vi "单体采集信息-new1.vi"(0 "can卡类型":u8, 1 "设备索引号":u8, 2 "CAN端口":u8, 3 "VIC_Receive":refnum<vi>, 4 "数据":refnum<vi>, 5 "数据位置":refnum<vi>) -> ()   [LabVIEW 2013]
panel:
  out "Life:":dbl=25.0
  in  "213":bool
  in  "一次置位":bool
  in  "刷新":bool
  out "VCI_Receive 2":T1
  in  "板号":u8
  out "电池信息":T2
  in  "电池信息读取":bool
  out "时间":string
  in  "充电均衡":u32(colorbox)=6618880
  in  "放电均衡":u32(colorbox)=16711680
  out "均衡信息":string[][](table)=[["第1串", "1", "单体检测其它故障", "第25串", "1", "单体检测其它故障", "第49串", "1", "单体检测其它故障", "第73串", "1", "单体检测其它故障", "第97串", "1", "单体检测其它故障", "第121串", "1", "单体检测其它故障", "第145串", "1", "单体检测其它故障", "第169串", "1", "单体检测其它故障", "第193串", "1", "单体检测其它故障", "第217串", "1", "单体检测其它故障", "第241串", "1", "单体检测其它故障", "第265串", "1", "单体检测其它故障", "第289串", "1", "单体检测其它故障", ""], ["第2串", "", "", "第26串", "", "", "第50串", "", "", "第74串", "", "", "第98串", "", "", "第122串", "", "", "第146串", "", "", "第170串", "", "", "第194串", "", "", "第218串", "", "", "第242串", "", "", "第266串", "", "", "第290串", "", "", ""], ["第3串", "", "", "第27串", "", "", "第51串", "", "", "第75串", "", "", "第99串", "", "", "第123串", "", "", "第147串", "", "", "第171串", "", "", "第195串", "", "", "第219串", "", "", "第243串", "", "", "第267串", "", "", "第291串", "", "", ""], ["第4串", "", "", "第28串", "", "", "第52串", "", "", "第76串", "", "", "第100串", "", "", "第124串", "", "", "第148串", "", "", "第172串", "", "", "第196串", "", "", "第220串", "", "", "第244串", "", "", "第268串", "", "", "第292串", "", "", ""], ["第5串", "", "", "第29串", "", "", "第53串", "", "", "第77串", "", "", "第101串", "", "", "第125串", "", "", "第149串", "", "", "第173串", "", "", "第197串", "", "", "第221串", "", "", "第245串", "", "", "第269串", "", "", "第293串", "", "", ""], ["第6串", "", "", "第30串", "", "", "第54串", "", "", "第78串", "", "", "第102串", "", "", "第126串", "", "", "第150串", "", "", "第174串", "", "", "第198串", "", "", "第222串", "", "", "第246串", "", "", "第270串", "", "", "第294串", "", "", ""], ["第7串", "", "", "第31串", "", "", "第55串", "", "", "第79串", "", "", "第103串", "", "", "第127串", "", "", "第151串", "", "", "第175串", "", "", "第199串", "", "", "第223串", "", "", "第247串", "", "", "第271串", "", "", "第295串", "", "", ""], ["第8串", "", "", "第32串", "", "", "第56串", "", "", "第80串", "", "", "第104串", "", "", "第128串", "", "", "第152串", "", "", "第176串", "", "", "第200串", "", "", "第224串", "", "", "第248串", "", "", "第272串", "", "", "第296串", "", "", ""], ["第9串", "", "", "第33串", "", "", "第57串", "", "", "第81串", "", "", "第105串", "", "", "第129串", "", "", "第153串", "", "", "第177串", "", "", "第201串", "", "", "第225串", "", "", "第249串", "", "", "第273串", "", "", "第297串", "", "", ""], ["第10串", "", "", "第34串", "", "", "第58串", "", "", "第82串", "", "", "第106串", "", "", "第130串", "", "", "第154串", "", "", "第178串", "", "", "第202串", "", "", "第226串", "", "", "第250串", "", "", "第274串", "", "", "第298串", "", "", ""], ["第11串", "", "", "第35串", "", "", "第59串", "", "", "第83串", "", "", "第107串", "", "", "第131串", "", "", "第155串", "", "", "第179串", "", "", "第203串", "", "", "第227串", "", "", "第251串", "", "", "第275串", "", "", "第299串", "", "", ""], ["第12串", "", "", "第36串", "", "", "第60串", "", "", "第84串", "", "", "第108串", "", "", "第132串", "", "", "第156串", "", "", "第180串", "", "", "第204串", "", "", "第228串", "", "", "第252串", "", "", "第276串", "", "", "第300串", "", "", ""], ["第13串", "", "", "第37串", "", "", "第61串", "", "", "第85串", "", "", "第109串", "", "", "第133串", "", "", "第157串", "", "", "第181串", "", "", "第205串", "", "", "第229串", "", "", "第253串", "", "", "第277串", "", "", "", "", "", ""], ["第14串", "", "", "第38串", "", "", "第62串", "", "", "第86串", "", "", "第110串", "", "", "第134串", "", "", "第158串", "", "", "第182串", "", "", "第206串", "", "", "第230串", "", "", "第254串", "", "", "第278串", "", "", "", "", "", ""], ["第15串", "", "", "第39串", "", "", "第63串", "", "", "第87串", "", "", "第111串", "", "", "第135串", "", "", "第159串", "", "", "第183串", "", "", "第207串", "", "", "第231串", "", "", "第255串", "", "", "第279串", "", "", "", "", "", ""], ["第16串", "", "", "第40串", "", "", "第64串", "", "", "第88串", "", "", "第112串", "", "", "第136串", "", "", "第160串", "", "", "第184串", "", "", "第208串", "", "", "第232串", "", "", "第256串", "", "", "第280串", "", "", "", "", "", ""], ["第17串", "", "", "第41串", "", "", "第65串", "", "", "第89串", "", "", "第113串", "", "", "第137串", "", "", "第161串", "", "", "第185串", "", "", "第209串", "", "", "第233串", "", "", "第257串", "", "", "第281串", "", "", "", "", "", ""], ["第18串", "", "", "第42串", "", "", "第66串", "", "", "第90串", "", "", "第114串", "", "", "第138串", "", "", "第162串", "", "", "第186串", "", "", "第210串", "", "", "第234串", "", "", "第258串", "", "", "第282串", "", "", "", "", "", ""], ["第19串", "", "", "第43串", "", "", "第67串", "", "", "第91串", "", "", "第115串", "", "", "第139串", "", "", "第163串", "", "", "第187串", "", "", "第211串", "", "", "第235串", "", "", "第259串", "", "", "第283串", "", "", "", "", "", ""], ["第20串", "", "", "第44串", "", "", "第68串", "", "", "第92串", "", "", "第116串", "", "", "第140串", "", "", "第164串", "", "", "第188串", "", "", "第212串", "", "", "第236串", "", "", "第260串", "", "", "第284串", "", "", "", "", "", ""], ["第21串", "", "", "第45串", "", "", "第69串", "", "", "第93串", "", "", "第117串", "", "", "第141串", "", "", "第165串", "", "", "第189串", "", "", "第213串", "", "", "第237串", "", "", "第261串", "", "", "第285串", "", "", "", "", "", ""], ["第22串", "", "", "第46串", "", "", "第70串", "", "", "第94串", "", "", "第118串", "", "", "第142串", "", "", "第166串", "", "", "第190串", "", "", "第214串", "", "", "第238串", "", "", "第262串", "", "", "第286串", "", "", "", "", "", ""], ["第23串", "", "", "第47串", "", "", "第71串", "", "", "第95串", "", "", "第119串", "", "", "第143串", "", "", "第167串", "", "", "第191串", "", "", "第215串", "", "", "第239串", "", "", "第263串", "", "", "第287串", "", "", "", "", "", ""], ["第24串", "", "", "第48串", "", "", "第72串", "", "", "第96串", "", "", "第120串", "", "", "第144串", "", "", "第168串", "", "", "第192串", "", "", "第216串", "", "", "第240串", "", "", "第264串", "", "", "第288串", "", "", "", "", "", ""]]
  out "SOC":string[][](table)=[["第1串", "", "", "第25串", "", "", "第49串", "", "", "第73串", "", "", "第97串", "", "", "第121串", "", "", "第145串", "", "", "第169串", "", "", "第193串", "", "", "第217串", "", "", "第241串", "", "", "第265串", "", "", "第289串", "", "", ""], ["第2串", "", "", "第26串", "", "", "第50串", "", "", "第74串", "", "", "第98串", "", "", "第122串", "", "", "第146串", "", "", "第170串", "", "", "第194串", "", "", "第218串", "", "", "第242串", "", "", "第266串", "", "", "第290串", "", "", ""], ["第3串", "", "", "第27串", "", "", "第51串", "", "", "第75串", "", "", "第99串", "", "", "第123串", "", "", "第147串", "", "", "第171串", "", "", "第195串", "", "", "第219串", "", "", "第243串", "", "", "第267串", "", "", "第291串", "", "", ""], ["第4串", "", "", "第28串", "", "", "第52串", "", "", "第76串", "", "", "第100串", "", "", "第124串", "", "", "第148串", "", "", "第172串", "", "", "第196串", "", "", "第220串", "", "", "第244串", "", "", "第268串", "", "", "第292串", "", "", ""], ["第5串", "", "", "第29串", "", "", "第53串", "", "", "第77串", "", "", "第101串", "", "", "第125串", "", "", "第149串", "", "", "第173串", "", "", "第197串", "", "", "第221串", "", "", "第245串", "", "", "第269串", "", "", "第293串", "", "", ""], ["第6串", "", "", "第30串", "", "", "第54串", "", "", "第78串", "", "", "第102串", "", "", "第126串", "", "", "第150串", "", "", "第174串", "", "", "第198串", "", "", "第222串", "", "", "第246串", "", "", "第270串", "", "", "第294串", "", "", ""], ["第7串", "", "", "第31串", "", "", "第55串", "", "", "第79串", "", "", "第103串", "", "", "第127串", "", "", "第151串", "", "", "第175串", "", "", "第199串", "", "", "第223串", "", "", "第247串", "", "", "第271串", "", "", "第295串", "", "", ""], ["第8串", "", "", "第32串", "", "", "第56串", "", "", "第80串", "", "", "第104串", "", "", "第128串", "", "", "第152串", "", "", "第176串", "", "", "第200串", "", "", "第224串", "", "", "第248串", "", "", "第272串", "", "", "第296串", "", "", ""], ["第9串", "", "", "第33串", "", "", "第57串", "", "", "第81串", "", "", "第105串", "", "", "第129串", "", "", "第153串", "", "", "第177串", "", "", "第201串", "", "", "第225串", "", "", "第249串", "", "", "第273串", "", "", "第297串", "", "", ""], ["第10串", "", "", "第34串", "", "", "第58串", "", "", "第82串", "", "", "第106串", "", "", "第130串", "", "", "第154串", "", "", "第178串", "", "", "第202串", "", "", "第226串", "", "", "第250串", "", "", "第274串", "", "", "第298串", "", "", ""], ["第11串", "", "", "第35串", "", "", "第59串", "", "", "第83串", "", "", "第107串", "", "", "第131串", "", "", "第155串", "", "", "第179串", "", "", "第203串", "", "", "第227串", "", "", "第251串", "", "", "第275串", "", "", "第299串", "", "", ""], ["第12串", "", "", "第36串", "", "", "第60串", "", "", "第84串", "", "", "第108串", "", "", "第132串", "", "", "第156串", "", "", "第180串", "", "", "第204串", "", "", "第228串", "", "", "第252串", "", "", "第276串", "", "", "第300串", "", "", ""], ["第13串", "", "", "第37串", "", "", "第61串", "", "", "第85串", "", "", "第109串", "", "", "第133串", "", "", "第157串", "", "", "第181串", "", "", "第205串", "", "", "第229串", "", "", "第253串", "", "", "第277串", "", "", "", "", "", ""], ["第14串", "", "", "第38串", "", "", "第62串", "", "", "第86串", "", "", "第110串", "", "", "第134串", "", "", "第158串", "", "", "第182串", "", "", "第206串", "", "", "第230串", "", "", "第254串", "", "", "第278串", "", "", "", "", "", ""], ["第15串", "", "", "第39串", "", "", "第63串", "", "", "第87串", "", "", "第111串", "", "", "第135串", "", "", "第159串", "", "", "第183串", "", "", "第207串", "", "", "第231串", "", "", "第255串", "", "", "第279串", "", "", "", "", "", ""], ["第16串", "", "", "第40串", "", "", "第64串", "", "", "第88串", "", "", "第112串", "", "", "第136串", "", "", "第160串", "", "", "第184串", "", "", "第208串", "", "", "第232串", "", "", "第256串", "", "", "第280串", "", "", "", "", "", ""], ["第17串", "", "", "第41串", "", "", "第65串", "", "", "第89串", "", "", "第113串", "", "", "第137串", "", "", "第161串", "", "", "第185串", "", "", "第209串", "", "", "第233串", "", "", "第257串", "", "", "第281串", "", "", "", "", "", ""], ["第18串", "", "", "第42串", "", "", "第66串", "", "", "第90串", "", "", "第114串", "", "", "第138串", "", "", "第162串", "", "", "第186串", "", "", "第210串", "", "", "第234串", "", "", "第258串", "", "", "第282串", "", "", "", "", "", ""], ["第19串", "", "", "第43串", "", "", "第67串", "", "", "第91串", "", "", "第115串", "", "", "第139串", "", "", "第163串", "", "", "第187串", "", "", "第211串", "", "", "第235串", "", "", "第259串", "", "", "第283串", "", "", "", "", "", ""], ["第20串", "", "", "第44串", "", "", "第68串", "", "", "第92串", "", "", "第116串", "", "", "第140串", "", "", "第164串", "", "", "第188串", "", "", "第212串", "", "", "第236串", "", "", "第260串", "", "", "第284串", "", "", "", "", "", ""], ["第21串", "", "", "第45串", "", "", "第69串", "", "", "第93串", "", "", "第117串", "", "", "第141串", "", "", "第165串", "", "", "第189串", "", "", "第213串", "", "", "第237串", "", "", "第261串", "", "", "第285串", "", "", "", "", "", ""], ["第22串", "", "", "第46串", "", "", "第70串", "", "", "第94串", "", "", "第118串", "", "", "第142串", "", "", "第166串", "", "", "第190串", "", "", "第214串", "", "", "第238串", "", "", "第262串", "", "", "第286串", "", "", "", "", "", ""], ["第23串", "", "", "第47串", "", "", "第71串", "", "", "第95串", "", "", "第119串", "", "", "第143串", "", "", "第167串", "", "", "第191串", "", "", "第215串", "", "", "第239串", "", "", "第263串", "", "", "第287串", "", "", "", "", "", ""], ["第24串", "", "", "第48串", "", "", "第72串", "", "", "第96串", "", "", "第120串", "", "", "第144串", "", "", "第168串", "", "", "第192串", "", "", "第216串", "", "", "第240串", "", "", "第264串", "", "", "第288串", "", "", "", "", "", ""]]
  out "内阻":string[][](table)=[["第1串", "", "", "第25串", "", "", "第49串", "", "", "第73串", "", "", "第97串", "", "", "第121串", "", "", "第145串", "", "", "第169串", "", "", "第193串", "", "", "第217串", "", "", "第241串", "", "", "第265串", "", "", "第289串", "", "", ""], ["第2串", "", "", "第26串", "", "", "第50串", "", "", "第74串", "", "", "第98串", "", "", "第122串", "", "", "第146串", "", "", "第170串", "", "", "第194串", "", "", "第218串", "", "", "第242串", "", "", "第266串", "", "", "第290串", "", "", ""], ["第3串", "", "", "第27串", "", "", "第51串", "", "", "第75串", "", "", "第99串", "", "", "第123串", "", "", "第147串", "", "", "第171串", "", "", "第195串", "", "", "第219串", "", "", "第243串", "", "", "第267串", "", "", "第291串", "", "", ""], ["第4串", "", "", "第28串", "", "", "第52串", "", "", "第76串", "", "", "第100串", "", "", "第124串", "", "", "第148串", "", "", "第172串", "", "", "第196串", "", "", "第220串", "", "", "第244串", "", "", "第268串", "", "", "第292串", "", "", ""], ["第5串", "", "", "第29串", "", "", "第53串", "", "", "第77串", "", "", "第101串", "", "", "第125串", "", "", "第149串", "", "", "第173串", "", "", "第197串", "", "", "第221串", "", "", "第245串", "", "", "第269串", "", "", "第293串", "", "", ""], ["第6串", "", "", "第30串", "", "", "第54串", "", "", "第78串", "", "", "第102串", "", "", "第126串", "", "", "第150串", "", "", "第174串", "", "", "第198串", "", "", "第222串", "", "", "第246串", "", "", "第270串", "", "", "第294串", "", "", ""], ["第7串", "", "", "第31串", "", "", "第55串", "", "", "第79串", "", "", "第103串", "", "", "第127串", "", "", "第151串", "", "", "第175串", "", "", "第199串", "", "", "第223串", "", "", "第247串", "", "", "第271串", "", "", "第295串", "", "", ""], ["第8串", "", "", "第32串", "", "", "第56串", "", "", "第80串", "", "", "第104串", "", "", "第128串", "", "", "第152串", "", "", "第176串", "", "", "第200串", "", "", "第224串", "", "", "第248串", "", "", "第272串", "", "", "第296串", "", "", ""], ["第9串", "", "", "第33串", "", "", "第57串", "", "", "第81串", "", "", "第105串", "", "", "第129串", "", "", "第153串", "", "", "第177串", "", "", "第201串", "", "", "第225串", "", "", "第249串", "", "", "第273串", "", "", "第297串", "", "", ""], ["第10串", "", "", "第34串", "", "", "第58串", "", "", "第82串", "", "", "第106串", "", "", "第130串", "", "", "第154串", "", "", "第178串", "", "", "第202串", "", "", "第226串", "", "", "第250串", "", "", "第274串", "", "", "第298串", "", "", ""], ["第11串", "", "", "第35串", "", "", "第59串", "", "", "第83串", "", "", "第107串", "", "", "第131串", "", "", "第155串", "", "", "第179串", "", "", "第203串", "", "", "第227串", "", "", "第251串", "", "", "第275串", "", "", "第299串", "", "", ""], ["第12串", "", "", "第36串", "", "", "第60串", "", "", "第84串", "", "", "第108串", "", "", "第132串", "", "", "第156串", "", "", "第180串", "", "", "第204串", "", "", "第228串", "", "", "第252串", "", "", "第276串", "", "", "第300串", "", "", ""], ["第13串", "", "", "第37串", "", "", "第61串", "", "", "第85串", "", "", "第109串", "", "", "第133串", "", "", "第157串", "", "", "第181串", "", "", "第205串", "", "", "第229串", "", "", "第253串", "", "", "第277串", "", "", "", "", "", ""], ["第14串", "", "", "第38串", "", "", "第62串", "", "", "第86串", "", "", "第110串", "", "", "第134串", "", "", "第158串", "", "", "第182串", "", "", "第206串", "", "", "第230串", "", "", "第254串", "", "", "第278串", "", "", "", "", "", ""], ["第15串", "", "", "第39串", "", "", "第63串", "", "", "第87串", "", "", "第111串", "", "", "第135串", "", "", "第159串", "", "", "第183串", "", "", "第207串", "", "", "第231串", "", "", "第255串", "", "", "第279串", "", "", "", "", "", ""], ["第16串", "", "", "第40串", "", "", "第64串", "", "", "第88串", "", "", "第112串", "", "", "第136串", "", "", "第160串", "", "", "第184串", "", "", "第208串", "", "", "第232串", "", "", "第256串", "", "", "第280串", "", "", "", "", "", ""], ["第17串", "", "", "第41串", "", "", "第65串", "", "", "第89串", "", "", "第113串", "", "", "第137串", "", "", "第161串", "", "", "第185串", "", "", "第209串", "", "", "第233串", "", "", "第257串", "", "", "第281串", "", "", "", "", "", ""], ["第18串", "", "", "第42串", "", "", "第66串", "", "", "第90串", "", "", "第114串", "", "", "第138串", "", "", "第162串", "", "", "第186串", "", "", "第210串", "", "", "第234串", "", "", "第258串", "", "", "第282串", "", "", "", "", "", ""], ["第19串", "", "", "第43串", "", "", "第67串", "", "", "第91串", "", "", "第115串", "", "", "第139串", "", "", "第163串", "", "", "第187串", "", "", "第211串", "", "", "第235串", "", "", "第259串", "", "", "第283串", "", "", "", "", "", ""], ["第20串", "", "", "第44串", "", "", "第68串", "", "", "第92串", "", "", "第116串", "", "", "第140串", "", "", "第164串", "", "", "第188串", "", "", "第212串", "", "", "第236串", "", "", "第260串", "", "", "第284串", "", "", "", "", "", ""], ["第21串", "", "", "第45串", "", "", "第69串", "", "", "第93串", "", "", "第117串", "", "", "第141串", "", "", "第165串", "", "", "第189串", "", "", "第213串", "", "", "第237串", "", "", "第261串", "", "", "第285串", "", "", "", "", "", ""], ["第22串", "", "", "第46串", "", "", "第70串", "", "", "第94串", "", "", "第118串", "", "", "第142串", "", "", "第166串", "", "", "第190串", "", "", "第214串", "", "", "第238串", "", "", "第262串", "", "", "第286串", "", "", "", "", "", ""], ["第23串", "", "", "第47串", "", "", "第71串", "", "", "第95串", "", "", "第119串", "", "", "第143串", "", "", "第167串", "", "", "第191串", "", "", "第215串", "", "", "第239串", "", "", "第263串", "", "", "第287串", "", "", "", "", "", ""], ["第24串", "", "", "第48串", "", "", "第72串", "", "", "第96串", "", "", "第120串", "", "", "第144串", "", "", "第168串", "", "", "第192串", "", "", "第216串", "", "", "第240串", "", "", "第264串", "", "", "第288串", "", "", "", "", "", ""]]
  out "温度表格":string[][](table)=[["第1串", "", "", "第25串", "", "", "第49串", "", "", "第73串", "", "", "第97串", "", "", "第121串", "", "", "第145串", "", "", "第169串", "", "", "第193串", "", "", "第217串", "", "", "第241串", "", "", "第265串", "", "", "第289串", "", "", ""], ["第2串", "", "", "第26串", "", "", "第50串", "", "", "第74串", "", "", "第98串", "", "", "第122串", "", "", "第146串", "", "", "第170串", "", "", "第194串", "", "", "第218串", "", "", "第242串", "", "", "第266串", "", "", "第290串", "", "", ""], ["第3串", "", "", "第27串", "", "", "第51串", "", "", "第75串", "", "", "第99串", "", "", "第123串", "", "", "第147串", "", "", "第171串", "", "", "第195串", "", "", "第219串", "", "", "第243串", "", "", "第267串", "", "", "第291串", "", "", ""], ["第4串", "", "", "第28串", "", "", "第52串", "", "", "第76串", "", "", "第100串", "", "", "第124串", "", "", "第148串", "", "", "第172串", "", "", "第196串", "", "", "第220串", "", "", "第244串", "", "", "第268串", "", "", "第292串", "", "", ""], ["第5串", "", "", "第29串", "", "", "第53串", "", "", "第77串", "", "", "第101串", "", "", "第125串", "", "", "第149串", "", "", "第173串", "", "", "第197串", "", "", "第221串", "", "", "第245串", "", "", "第269串", "", "", "第293串", "", "", ""], ["第6串", "", "", "第30串", "", "", "第54串", "", "", "第78串", "", "", "第102串", "", "", "第126串", "", "", "第150串", "", "", "第174串", "", "", "第198串", "", "", "第222串", "", "", "第246串", "", "", "第270串", "", "", "第294串", "", "", ""], ["第7串", "", "", "第31串", "", "", "第55串", "", "", "第79串", "", "", "第103串", "", "", "第127串", "", "", "第151串", "", "", "第175串", "", "", "第199串", "", "", "第223串", "", "", "第247串", "", "", "第271串", "", "", "第295串", "", "", ""], ["第8串", "", "", "第32串", "", "", "第56串", "", "", "第80串", "", "", "第104串", "", "", "第128串", "", "", "第152串", "", "", "第176串", "", "", "第200串", "", "", "第224串", "", "", "第248串", "", "", "第272串", "", "", "第296串", "", "", ""], ["第9串", "", "", "第33串", "", "", "第57串", "", "", "第81串", "", "", "第105串", "", "", "第129串", "", "", "第153串", "", "", "第177串", "", "", "第201串", "", "", "第225串", "", "", "第249串", "", "", "第273串", "", "", "第297串", "", "", ""], ["第10串", "", "", "第34串", "", "", "第58串", "", "", "第82串", "", "", "第106串", "", "", "第130串", "", "", "第154串", "", "", "第178串", "", "", "第202串", "", "", "第226串", "", "", "第250串", "", "", "第274串", "", "", "第298串", "", "", ""], ["第11串", "", "", "第35串", "", "", "第59串", "", "", "第83串", "", "", "第107串", "", "", "第131串", "", "", "第155串", "", "", "第179串", "", "", "第203串", "", "", "第227串", "", "", "第251串", "", "", "第275串", "", "", "第299串", "", "", ""], ["第12串", "", "", "第36串", "", "", "第60串", "", "", "第84串", "", "", "第108串", "", "", "第132串", "", "", "第156串", "", "", "第180串", "", "", "第204串", "", "", "第228串", "", "", "第252串", "", "", "第276串", "", "", "第300串", "", "", ""], ["第13串", "", "", "第37串", "", "", "第61串", "", "", "第85串", "", "", "第109串", "", "", "第133串", "", "", "第157串", "", "", "第181串", "", "", "第205串", "", "", "第229串", "", "", "第253串", "", "", "第277串", "", "", "", "", "", ""], ["第14串", "", "", "第38串", "", "", "第62串", "", "", "第86串", "", "", "第110串", "", "", "第134串", "", "", "第158串", "", "", "第182串", "", "", "第206串", "", "", "第230串", "", "", "第254串", "", "", "第278串", "", "", "", "", "", ""], ["第15串", "", "", "第39串", "", "", "第63串", "", "", "第87串", "", "", "第111串", "", "", "第135串", "", "", "第159串", "", "", "第183串", "", "", "第207串", "", "", "第231串", "", "", "第255串", "", "", "第279串", "", "", "", "", "", ""], ["第16串", "", "", "第40串", "", "", "第64串", "", "", "第88串", "", "", "第112串", "", "", "第136串", "", "", "第160串", "", "", "第184串", "", "", "第208串", "", "", "第232串", "", "", "第256串", "", "", "第280串", "", "", "", "", "", ""], ["第17串", "", "", "第41串", "", "", "第65串", "", "", "第89串", "", "", "第113串", "", "", "第137串", "", "", "第161串", "", "", "第185串", "", "", "第209串", "", "", "第233串", "", "", "第257串", "", "", "第281串", "", "", "", "", "", ""], ["第18串", "", "", "第42串", "", "", "第66串", "", "", "第90串", "", "", "第114串", "", "", "第138串", "", "", "第162串", "", "", "第186串", "", "", "第210串", "", "", "第234串", "", "", "第258串", "", "", "第282串", "", "", "", "", "", ""], ["第19串", "", "", "第43串", "", "", "第67串", "", "", "第91串", "", "", "第115串", "", "", "第139串", "", "", "第163串", "", "", "第187串", "", "", "第211串", "", "", "第235串", "", "", "第259串", "", "", "第283串", "", "", "", "", "", ""], ["第20串", "", "", "第44串", "", "", "第68串", "", "", "第92串", "", "", "第116串", "", "", "第140串", "", "", "第164串", "", "", "第188串", "", "", "第212串", "", "", "第236串", "", "", "第260串", "", "", "第284串", "", "", "", "", "", ""], ["第21串", "", "", "第45串", "", "", "第69串", "", "", "第93串", "", "", "第117串", "", "", "第141串", "", "", "第165串", "", "", "第189串", "", "", "第213串", "", "", "第237串", "", "", "第261串", "", "", "第285串", "", "", "", "", "", ""], ["第22串", "", "", "第46串", "", "", "第70串", "", "", "第94串", "", "", "第118串", "", "", "第142串", "", "", "第166串", "", "", "第190串", "", "", "第214串", "", "", "第238串", "", "", "第262串", "", "", "第286串", "", "", "", "", "", ""], ["第23串", "", "", "第47串", "", "", "第71串", "", "", "第95串", "", "", "第119串", "", "", "第143串", "", "", "第167串", "", "", "第191串", "", "", "第215串", "", "", "第239串", "", "", "第263串", "", "", "第287串", "", "", "", "", "", ""], ["第24串", "", "", "第48串", "", "", "第72串", "", "", "第96串", "", "", "第120串", "", "", "第144串", "", "", "第168串", "", "", "第192串", "", "", "第216串", "", "", "第240串", "", "", "第264串", "", "", "第288串", "", "", "", "", "", ""]]
  in  "主界面选项":T3(radio)
  in  "电池信息选项":enum16{"电池信息", "历史信息"}(ring)
  out "位置":dbl[](array[numeric])
  out "输出数据":dbl[](array[numeric])
  in  "命令":u32=133
  in  "VCI_Receive":T1 {"Rsv3" max=0 format="%x"; "Rsv2" min=101 format="%x"; "Rsv1" format="%x"; "Data8" format="%x"; "Data7" format="%x"; "Data6" format="%x"; "Data5" format="%x"; "Data4" format="%x"; "Data3" format="%x"; "Data2" format="%x"; "Data1" format="%x"; "DataLen" format="%x"; "ExternFlag" format="%x"; "RemoteFlag" format="%x"; "SendType" format="%x"; "TimeFlag" format="%x"; "TimeStamp" format="%x"; "ID" format="%x"}
  out "状态":bool
  in  "停止":bool
  in  "选项卡控件":enum32{"单体电压", "单体温度", "单体内阻", "单体SOC"}(tab)
  in  "偏差":dbl=0.008 format="%.3f"
  in  "基准":dbl=3.3 format="%.3f"
  out "等待均衡":u32(colorbox)=16776770
  in  "故障信息选择按键 2":enum32{"单选选项2", "单选选项2 2", "单选选项2 3", "单选选项1"}(radio)=enum."单选选项1"
  out "电压选择":enum32{"1-96", "97-192", "193-288", "289-300"}(tab)
  out "1":T4={"1 102"={"第1串"=0.0, "第2串"=0.0, "第3串"=0.0, "第4串"=0.0, "第5串"=0.0, "第6串"=0.0, "第7串"=0.0, "第8串"=0.0, "第9串"=0.0, "第10串"=0.0, "第11串"=0.0, "第12串"=0.0, "第一串 2"=0.0, "第一串 4"=0.0, "第一串 6"=0.0, "第一串 8"=0.0, "第一串 10"=0.0, "第一串 12"=0.0, "第一串 14"=0.0, "第一串 16"=0.0, "第一串 18"=0.0, "第一串 20"=0.0, "第一串 22"=0.0, "第一串 24"=0.0}, "1 3"={"第13串"=0.0, "第14串"=0.0, "第15串"=0.0, "第16串"=0.0, "第17串"=0.0, "第18串"=0.0, "第19串"=0.0, "第20串"=0.0, "第21串"=0.0, "第22串"=0.0, "第23串"=0.0, "第24串"=0.0, "第一串 2"=0.0, "第一串 4"=0.0, "第一串 6"=0.0, "第一串 8"=0.0, "第一串 10"=0.0, "第一串 12"=0.0, "第一串 14"=0.0, "第一串 16"=0.0, "第一串 18"=0.0, "第一串 20"=0.0, "第一串 22"=0.0, "第一串 24"=0.0}, "1 4"={"第25串"=0.0, "第26串"=0.0, "第27串"=0.0, "第28串"=0.0, "第29串"=0.0, "第30串"=0.0, "第31串"=0.0, "第32串"=0.0, "第33串"=0.0, "第34串"=0.0, "第35串"=0.0, "第36串"=0.0, "第一串 2"=0.0, "第一串 4"=0.0, "第一串 6"=0.0, "第一串 8"=0.0, "第一串 10"=0.0, "第一串 12"=0.0, "第一串 14"=0.0, "第一串 16"=0.0, "第一串 18"=0.0, "第一串 20"=0.0, "第一串 22"=0.0, "第一串 24"=0.0}, "1 6"={"第37串"=0.0, "第38串"=0.0, "第39串"=0.0, "第40串"=0.0, "第41串"=0.0, "第42串"=0.0, "第43串"=0.0, "第44串"=0.0, "第45串"=0.0, "第46串"=0.0, "第47串"=0.0, "第48串"=0.0, "第一串 2"=0.0, "第一串 4"=0.0, "第一串 6"=0.0, "第一串 8"=0.0, "第一串 10"=0.0, "第一串 12"=0.0, "第一串 14"=0.0, "第一串 16"=0.0, "第一串 18"=0.0, "第一串 20"=0.0, "第一串 22"=0.0, "第一串 24"=0.0}, "1 7"={"第49串"=0.0, "第50串"=0.0, "第51串"=0.0, "第52串"=0.0, "第53串"=0.0, "第54串"=0.0, "第55串"=0.0, "第56串"=0.0, "第57串"=0.0, "第58串"=0.0, "第59串"=0.0, "第60串"=0.0, "第一串 2"=0.0, "第一串 4"=0.0, "第一串 6"=0.0, "第一串 8"=0.0, "第一串 10"=0.0, "第一串 12"=0.0, "第一串 14"=0.0, "第一串 16"=0.0, "第一串 18"=0.0, "第一串 20"=0.0, "第一串 22"=0.0, "第一串 24"=0.0}, "1 8"={"第61串"=0.0, "第62串"=0.0, "第63串"=0.0, "第64串"=0.0, "第65串"=0.0, "第66串"=0.0, "第67串"=0.0, "第68串"=0.0, "第69串"=0.0, "第70串"=0.0, "第71串"=0.0, "第72串"=0.0, "第一串 2"=0.0, "第一串 4"=0.0, "第一串 6"=0.0, "第一串 8"=0.0, "第一串 10"=0.0, "第一串 12"=0.0, "第一串 14"=0.0, "第一串 16"=0.0, "第一串 18"=0.0, "第一串 20"=0.0, "第一串 22"=0.0, "第一串 24"=0.0}, "1 9"={"第73串"=0.0, "第74串"=0.0, "第75串"=0.0, "第76串"=0.0, "第77串"=0.0, "第78串"=0.0, "第79串"=0.0, "第80串"=0.0, "第81串"=0.0, "第82串"=0.0, "第83串"=0.0, "第84串"=0.0, "第一串 2"=0.0, "第一串 4"=0.0, "第一串 6"=0.0, "第一串 8"=0.0, "第一串 10"=0.0, "第一串 12"=0.0, "第一串 14"=0.0, "第一串 16"=0.0, "第一串 18"=0.0, "第一串 20"=0.0, "第一串 22"=0.0, "第一串 24"=0.0}, "1 10"={"第85串"=0.0, "第86串"=0.0, "第87串"=0.0, "第88串"=0.0, "第89串"=0.0, "第90串"=0.0, "第91串"=0.0, "第92串"=0.0, "第93串"=0.0, "第94串"=0.0, "第95串"=0.0, "第96串"=0.0, "第一串 2"=0.0, "第一串 4"=0.0, "第一串 6"=0.0, "第一串 8"=0.0, "第一串 10"=0.0, "第一串 12"=0.0, "第一串 14"=0.0, "第一串 16"=0.0, "第一串 18"=0.0, "第一串 20"=0.0, "第一串 22"=0.0, "第一串 24"=0.0}, "1 12"={"充电1"=13816530, "充电1"=13816530, "充电1"=13816530, "充电1"=13816530, "充电1"=13816530, "充电1"=13816530, "充电1"=13816530, "充电1"=13816530, "充电1"=13816530, "充电1"=13816530, "充电1"=13816530, "充电1"=13816530}, "1 28"={"充电1"=13816530, "充电1"=13816530, "充电1"=13816530, "充电1"=13816530, "充电1"=13816530, "充电1"=13816530, "充电1"=13816530, "充电1"=13816530, "充电1"=13816530, "充电1"=13816530, "充电1"=13816530, "充电1"=13816530}, "1 25"={"充电1"=0, "充电1"=0, "充电1"=0, "充电1"=0, "充电1"=0, "充电1"=0, "充电1"=0, "充电1"=0, "充电1"=0, "充电1"=0, "充电1"=0, "充电1"=0}, "1 31"={"充电1"=0, "充电1"=0, "充电1"=0, "充电1"=0, "充电1"=0, "充电1"=0, "充电1"=0, "充电1"=0, "充电1"=0, "充电1"=0, "充电1"=0, "充电1"=0}, "1 16"={"充电1"=0, "充电1"=0, "充电1"=0, "充电1"=0, "充电1"=0, "充电1"=0, "充电1"=0, "充电1"=0, "充电1"=0, "充电1"=0, "充电1"=0, "充电1"=0}, "1 19"={"充电1"=0, "充电1"=0, "充电1"=0, "充电1"=0, "充电1"=0, "充电1"=0, "充电1"=0, "充电1"=0, "充电1"=0, "充电1"=0, "充电1"=0, "充电1"=0}, "1 22"={"充电1"=0, "充电1"=0, "充电1"=0, "充电1"=0, "充电1"=0, "充电1"=0, "充电1"=0, "充电1"=0, "充电1"=0, "充电1"=0, "充电1"=0, "充电1"=0}, "1 34"={"充电1"=0, "充电1"=0, "充电1"=0, "充电1"=0, "充电1"=0, "充电1"=0, "充电1"=0, "充电1"=0, "充电1"=0, "充电1"=0, "充电1"=0, "充电1"=0}, "1 11"={"充电1"=13816530, "充电1"=13816530, "充电1"=13816530, "充电1"=13816530, "充电1"=13816530, "充电1"=13816530, "充电1"=13816530, "充电1"=13816530, "充电1"=13816530, "充电1"=13816530, "充电1"=13816530, "充电1"=13816530}, "1 27"={"充电1"=0, "充电1"=0, "充电1"=0, "充电1"=0, "充电1"=0, "充电1"=0, "充电1"=0, "充电1"=0, "充电1"=0, "充电1"=0, "充电1"=0, "充电1"=0}, "1 24"={"充电1"=0, "充电1"=0, "充电1"=0, "充电1"=0, "充电1"=0, "充电1"=0, "充电1"=0, "充电1"=0, "充电1"=0, "充电1"=0, "充电1"=0, "充电1"=0}, "1 30"={"充电1"=0, "充电1"=0, "充电1"=0, "充电1"=0, "充电1"=0, "充电1"=0, "充电1"=0, "充电1"=0, "充电1"=0, "充电1"=0, "充电1"=0, "充电1"=0}, "1 15"={"充电1"=0, "充电1"=0, "充电1"=0, "充电1"=0, "充电1"=0, "充电1"=0, "充电1"=0, "充电1"=0, "充电1"=0, "充电1"=0, "充电1"=0, "充电1"=0}, "1 18"={"充电1"=0, "充电1"=0, "充电1"=0, "充电1"=0, "充电1"=0, "充电1"=0, "充电1"=0, "充电1"=0, "充电1"=0, "充电1"=0, "充电1"=0, "充电1"=0}, "1 21"={"充电1"=0, "充电1"=0, "充电1"=0, "充电1"=0, "充电1"=0, "充电1"=0, "充电1"=0, "充电1"=0, "充电1"=0, "充电1"=0, "充电1"=0, "充电1"=0}, "1 33"={"充电1"=0, "充电1"=0, "充电1"=0, "充电1"=0, "充电1"=0, "充电1"=0, "充电1"=0, "充电1"=0, "充电1"=0, "充电1"=0, "充电1"=0, "充电1"=0}, "1 13"={"均衡故障"=0, "均衡故障 2"=0.0, "均衡故障 3"=0.0, "均衡故障 4"=0.0, "均衡故障 5"=0.0, "均衡故障 6"=0.0, "均衡故障 7"=0.0, "均衡故障 8"=0.0, "均衡故障 9"=0.0, "均衡故障 10"=0.0, "均衡故障 11"=0.0, "均衡故障 12"=0.0}, "1 26"={"均衡故障"=0, "均衡故障 2"=0.0, "均衡故障 3"=0.0, "均衡故障 4"=0.0, "均衡故障 5"=0.0, "均衡故障 6"=0.0, "均衡故障 7"=0.0, "均衡故障 8"=0.0, "均衡故障 9"=0.0, "均衡故障 10"=0.0, "均衡故障 11"=0.0, "均衡故障 12"=0.0}, "1 23"={"均衡故障"=0, "均衡故障 2"=0.0, "均衡故障 3"=0.0, "均衡故障 4"=0.0, "均衡故障 5"=0.0, "均衡故障 6"=0.0, "均衡故障 7"=0.0, "均衡故障 8"=0.0, "均衡故障 9"=0.0, "均衡故障 10"=0.0, "均衡故障 11"=0.0, "均衡故障 12"=0.0}, "1 29"={"均衡故障"=0, "均衡故障 2"=0.0, "均衡故障 3"=0.0, "均衡故障 4"=0.0, "均衡故障 5"=0.0, "均衡故障 6"=0.0, "均衡故障 7"=0.0, "均衡故障 8"=0.0, "均衡故障 9"=0.0, "均衡故障 10"=0.0, "均衡故障 11"=0.0, "均衡故障 12"=0.0}, "1 14"={"均衡故障"=0, "均衡故障 2"=0.0, "均衡故障 3"=0.0, "均衡故障 4"=0.0, "均衡故障 5"=0.0, "均衡故障 6"=0.0, "均衡故障 7"=0.0, "均衡故障 8"=0.0, "均衡故障 9"=0.0, "均衡故障 10"=0.0, "均衡故障 11"=0.0, "均衡故障 12"=0.0}, "1 17"={"均衡故障"=0, "均衡故障 2"=0.0, "均衡故障 3"=0.0, "均衡故障 4"=0.0, "均衡故障 5"=0.0, "均衡故障 6"=0.0, "均衡故障 7"=0.0, "均衡故障 8"=0.0, "均衡故障 9"=0.0, "均衡故障 10"=0.0, "均衡故障 11"=0.0, "均衡故障 12"=0.0}, "1 20"={"均衡故障"=0, "均衡故障 2"=0.0, "均衡故障 3"=0.0, "均衡故障 4"=0.0, "均衡故障 5"=0.0, "均衡故障 6"=0.0, "均衡故障 7"=0.0, "均衡故障 8"=0.0, "均衡故障 9"=0.0, "均衡故障 10"=0.0, "均衡故障 11"=0.0, "均衡故障 12"=0.0}, "1 32"={"均衡故障"=0, "均衡故障 2"=0.0, "均衡故障 3"=0.0, "均衡故障 4"=0.0, "均衡故障 5"=0.0, "均衡故障 6"=0.0, "均衡故障 7"=0.0, "均衡故障 8"=0.0, "均衡故障 9"=0.0, "均衡故障 10"=0.0, "均衡故障 11"=0.0, "均衡故障 12"=0.0}} {"1 102"."第一串 24" format="%#.2f"; "1 102"."第12串" format="%.3f"; "1 102"."第一串 22" format="%#.2f"; "1 102"."第11串" format="%.3f"; "1 102"."第一串 20" format="%#.2f"; "1 102"."第10串" format="%.3f"; "1 102"."第一串 18" format="%#.2f"; "1 102"."第9串" format="%.3f"; "1 102"."第一串 16" format="%#.2f"; "1 102"."第8串" format="%.3f"; "1 102"."第一串 14" format="%#.2f"; "1 102"."第7串" format="%.3f"; "1 102"."第一串 12" format="%#.2f"; "1 102"."第6串" format="%.3f"; "1 102"."第一串 10" format="%#.2f"; "1 102"."第5串" format="%.3f"; "1 102"."第一串 8" format="%#.2f"; "1 102"."第4串" format="%.3f"; "1 102"."第一串 6" format="%#.2f"; "1 102"."第3串" format="%.3f"; "1 102"."第一串 4" format="%#.2f"; "1 102"."第2串" format="%.3f"; "1 102"."第一串 2" format="%#.2f"; "1 102"."第1串" format="%.3f"; "1 10"."第96串" format="%.3f"; "1 10"."第95串" format="%.3f"; "1 10"."第94串" format="%.3f"; "1 10"."第93串" format="%.3f"; "1 10"."第92串" format="%.3f"; "1 10"."第91串" format="%.3f"; "1 10"."第90串" format="%.3f"; "1 10"."第89串" format="%.3f"; "1 10"."第88串" format="%.3f"; "1 10"."第87串" format="%.3f"; "1 10"."第86串" format="%.3f"; "1 10"."第85串" format="%.3f"; "1 9"."第84串" format="%.3f"; "1 9"."第83串" format="%.3f"; "1 9"."第82串" format="%.3f"; "1 9"."第81串" format="%.3f"; "1 9"."第80串" format="%.3f"; "1 9"."第79串" format="%.3f"; "1 9"."第78串" format="%.3f"; "1 9"."第77串" format="%.3f"; "1 9"."第76串" format="%.3f"; "1 9"."第75串" format="%.3f"; "1 9"."第74串" format="%.3f"; "1 9"."第73串" format="%.3f"; "1 8"."第72串" format="%.3f"; "1 8"."第71串" format="%.3f"; "1 8"."第70串" format="%.3f"; "1 8"."第69串" format="%.3f"; "1 8"."第68串" format="%.3f"; "1 8"."第67串" format="%.3f"; "1 8"."第66串" format="%.3f"; "1 8"."第65串" format="%.3f"; "1 8"."第64串" format="%.3f"; "1 8"."第63串" format="%.3f"; "1 8"."第62串" format="%.3f"; "1 8"."第61串" format="%.3f"; "1 7"."第60串" format="%.3f"; "1 7"."第59串" format="%.3f"; "1 7"."第58串" format="%.3f"; "1 7"."第57串" format="%.3f"; "1 7"."第56串" format="%.3f"; "1 7"."第55串" format="%.3f"; "1 7"."第54串" format="%.3f"; "1 7"."第53串" format="%.3f"; "1 7"."第52串" format="%.3f"; "1 7"."第51串" format="%.3f"; "1 7"."第50串" format="%.3f"; "1 7"."第49串" format="%.3f"; "1 6"."第48串" format="%.3f"; "1 6"."第47串" format="%.3f"; "1 6"."第46串" format="%.3f"; "1 6"."第45串" format="%.3f"; "1 6"."第44串" format="%.3f"; "1 6"."第43串" format="%.3f"; "1 6"."第42串" format="%.3f"; "1 6"."第41串" format="%.3f"; "1 6"."第40串" format="%.3f"; "1 6"."第39串" format="%.3f"; "1 6"."第38串" format="%.3f"; "1 6"."第37串" format="%.3f"; "1 4"."第36串" format="%.3f"; "1 4"."第35串" format="%.3f"; "1 4"."第34串" format="%.3f"; "1 4"."第33串" format="%.3f"; "1 4"."第32串" format="%.3f"; "1 4"."第31串" format="%.3f"; "1 4"."第30串" format="%.3f"; "1 4"."第29串" format="%.3f"; "1 4"."第28串" format="%.3f"; "1 4"."第27串" format="%.3f"; "1 4"."第26串" format="%.3f"; "1 4"."第25串" format="%.3f"; "1 3"."第24串" format="%.3f"; "1 3"."第23串" format="%.3f"; "1 3"."第22串" format="%.3f"; "1 3"."第21串" format="%.3f"; "1 3"."第20串" format="%.3f"; "1 3"."第19串" format="%.3f"; "1 3"."第18串" format="%.3f"; "1 3"."第17串" format="%.3f"; "1 3"."第16串" format="%.3f"; "1 3"."第15串" format="%.3f"; "1 3"."第14串" format="%.3f"; "1 3"."第13串" format="%.3f"}
  out "2":T5={"1 26"={"第97串"=0.0, "第98串"=0.0, "第99串"=0.0, "第100串"=0.0, "第101串"=0.0, "第102串"=0.0, "第103串"=0.0, "第104串"=0.0, "第105串"=0.0, "第106串"=0.0, "第107串"=0.0, "第108串"=0.0, "第一串 2"=0.0, "第一串 4"=0.0, "第一串 6"=0.0, "第一串 8"=0.0, "第一串 10"=0.0, "第一串 12"=0.0, "第一串 14"=0.0, "第一串 16"=0.0, "第一串 18"=0.0, "第一串 20"=0.0, "第一串 22"=0.0, "第一串 24"=0.0}, "1 27"={"第109串"=0.0, "第110串"=0.0, "第111串"=0.0, "第112串"=0.0, "第113串"=0.0, "第114串"=0.0, "第115串"=0.0, "第116串"=0.0, "第117串"=0.0, "第118串"=0.0, "第119串"=0.0, "第120串"=0.0, "第一串 2"=0.0, "第一串 4"=0.0, "第一串 6"=0.0, "第一串 8"=0.0, "第一串 10"=0.0, "第一串 12"=0.0, "第一串 14"=0.0, "第一串 16"=0.0, "第一串 18"=0.0, "第一串 20"=0.0, "第一串 22"=0.0, "第一串 24"=0.0}, "1 28"={"第121串"=0.0, "第122串"=0.0, "第123串"=0.0, "第124串"=0.0, "第125串"=0.0, "第126串"=0.0, "第127串"=0.0, "第128串"=0.0, "第129串"=0.0, "第130串"=0.0, "第131串"=0.0, "第132串"=0.0, "第一串 2"=0.0, "第一串 4"=0.0, "第一串 6"=0.0, "第一串 8"=0.0, "第一串 10"=0.0, "第一串 12"=0.0, "第一串 14"=0.0, "第一串 16"=0.0, "第一串 18"=0.0, "第一串 20"=0.0, "第一串 22"=0.0, "第一串 24"=0.0}, "1 29"={"第133串"=0.0, "第134串"=0.0, "第135串"=0.0, "第136串"=0.0, "第137串"=0.0, "第138串"=0.0, "第139串"=0.0, "第140串"=0.0, "第141串"=0.0, "第142串"=0.0, "第143串"=0.0, "第144串"=0.0, "第一串 2"=0.0, "第一串 4"=0.0, "第一串 6"=0.0, "第一串 8"=0.0, "第一串 10"=0.0, "第一串 12"=0.0, "第一串 14"=0.0, "第一串 16"=0.0, "第一串 18"=0.0, "第一串 20"=0.0, "第一串 22"=0.0, "第一串 24"=0.0}, "1 30"={"第145串"=0.0, "第146串"=0.0, "第147串"=0.0, "第148串"=0.0, "第149串"=0.0, "第150串"=0.0, "第151串"=0.0, "第152串"=0.0, "第153串"=0.0, "第154串"=0.0, "第155串"=0.0, "第156串"=0.0, "第一串 2"=0.0, "第一串 4"=0.0, "第一串 6"=0.0, "第一串 8"=0.0, "第一串 10"=0.0, "第一串 12"=0.0, "第一串 14"=0.0, "第一串 16"=0.0, "第一串 18"=0.0, "第一串 20"=0.0, "第一串 22"=0.0, "第一串 24"=0.0}, "1 31"={"第157串"=0.0, "第158串"=0.0, "第159串"=0.0, "第160串"=0.0, "第161串"=0.0, "第162串"=0.0, "第163串"=0.0, "第164串"=0.0, "第165串"=0.0, "第166串"=0.0, "第167串"=0.0, "第168串"=0.0, "第一串 2"=0.0, "第一串 4"=0.0, "第一串 6"=0.0, "第一串 8"=0.0, "第一串 10"=0.0, "第一串 12"=0.0, "第一串 14"=0.0, "第一串 16"=0.0, "第一串 18"=0.0, "第一串 20"=0.0, "第一串 22"=0.0, "第一串 24"=0.0}, "1 32"={"第169串"=0.0, "第170串"=0.0, "第171串"=0.0, "第172串"=0.0, "第173串"=0.0, "第174串"=0.0, "第175串"=0.0, "第176串"=0.0, "第177串"=0.0, "第178串"=0.0, "第179串"=0.0, "第180串"=0.0, "第一串 2"=0.0, "第一串 4"=0.0, "第一串 6"=0.0, "第一串 8"=0.0, "第一串 10"=0.0, "第一串 12"=0.0, "第一串 14"=0.0, "第一串 16"=0.0, "第一串 18"=0.0, "第一串 20"=0.0, "第一串 22"=0.0, "第一串 24"=0.0}, "1 33"={"第181串"=0.0, "第182串"=0.0, "第183串"=0.0, "第184串"=0.0, "第185串"=0.0, "第186串"=0.0, "第187串"=0.0, "第188串"=0.0, "第189串"=0.0, "第190串"=0.0, "第191串"=0.0, "第192串"=0.0, "第一串 2"=0.0, "第一串 4"=0.0, "第一串 6"=0.0, "第一串 8"=0.0, "第一串 10"=0.0, "第一串 12"=0.0, "第一串 14"=0.0, "第一串 16"=0.0, "第一串 18"=0.0, "第一串 20"=0.0, "第一串 22"=0.0, "第一串 24"=0.0}, "1 16"={"充电1"=13816530, "充电1"=13816530, "充电1"=13816530, "充电1"=13816530, "充电1"=13816530, "充电1"=13816530, "充电1"=13816530, "充电1"=13816530, "充电1"=13816530, "充电1"=13816530, "充电1"=13816530, "充电1"=13816530}, "1 44"={"充电1"=13816530, "充电1"=13816530, "充电1"=13816530, "充电1"=13816530, "充电1"=13816530, "充电1"=13816530, "充电1"=13816530, "充电1"=13816530, "充电1"=13816530, "充电1"=13816530, "充电1"=13816530, "充电1"=13816530}, "1 36"={"充电1"=13816530, "充电1"=13816530, "充电1"=13816530, "充电1"=13816530, "充电1"=13816530, "充电1"=13816530, "充电1"=13816530, "充电1"=13816530, "充电1"=13816530, "充电1"=13816530, "充电1"=13816530, "充电1"=13816530}, "1 47"={"充电1"=13816530, "充电1"=13816530, "充电1"=13816530, "充电1"=13816530, "充电1"=13816530, "充电1"=13816530, "充电1"=13816530, "充电1"=13816530, "充电1"=13816530, "充电1"=13816530, "充电1"=13816530, "充电1"=13816530}, "1 19"={"充电1"=13816530, "充电1"=13816530, "充电1"=13816530, "充电1"=13816530, "充电1"=13816530, "充电1"=13816530, "充电1"=13816530, "充电1"=13816530, "充电1"=13816530, "充电1"=13816530, "充电1"=13816530, "充电1"=13816530}, "1 38"={"充电1"=13816530, "充电1"=13816530, "充电1"=13816530, "充电1"=13816530, "充电1"=13816530, "充电1"=13816530, "充电1"=13816530, "充电1"=13816530, "充电1"=13816530, "充电1"=13816530, "充电1"=13816530, "充电1"=13816530}, "1 41"={"充电1"=13816530, "充电1"=13816530, "充电1"=13816530, "充电1"=13816530, "充电1"=13816530, "充电1"=13816530, "充电1"=13816530, "充电1"=13816530, "充电1"=13816530, "充电1"=13816530, "充电1"=13816530, "充电1"=13816530}, "1 50"={"充电1"=13816530, "充电1"=13816530, "充电1"=13816530, "充电1"=13816530, "充电1"=13816530, "充电1"=13816530, "充电1"=13816530, "充电1"=13816530, "充电1"=13816530, "充电1"=13816530, "充电1"=13816530, "充电1"=13816530}, "1 15"={"充电1"=13816530, "充电1"=13816530, "充电1"=13816530, "充电1"=13816530, "充电1"=13816530, "充电1"=13816530, "充电1"=13816530, "充电1"=13816530, "充电1"=13816530, "充电1"=13816530, "充电1"=13816530, "充电1"=13816530}, "1 43"={"充电1"=13816530, "充电1"=13816530, "充电1"=13816530, "充电1"=13816530, "充电1"=13816530, "充电1"=13816530, "充电1"=13816530, "充电1"=13816530, "充电1"=13816530, "充电1"=13816530, "充电1"=13816530, "充电1"=13816530}, "1 35"={"充电1"=13816530, "充电1"=13816530, "充电1"=13816530, "充电1"=13816530, "充电1"=13816530, "充电1"=13816530, "充电1"=13816530, "充电1"=13816530, "充电1"=13816530, "充电1"=13816530, "充电1"=13816530, "充电1"=13816530}, "1 46"={"充电1"=13816530, "充电1"=13816530, "充电1"=13816530, "充电1"=13816530, "充电1"=13816530, "充电1"=13816530, "充电1"=13816530, "充电1"=13816530, "充电1"=13816530, "充电1"=13816530, "充电1"=13816530, "充电1"=13816530}, "1 18"={"充电1"=13816530, "充电1"=13816530, "充电1"=13816530, "充电1"=13816530, "充电1"=13816530, "充电1"=13816530, "充电1"=13816530, "充电1"=13816530, "充电1"=13816530, "充电1"=13816530, "充电1"=13816530, "充电1"=13816530}, "1 37"={"充电1"=13816530, "充电1"=13816530, "充电1"=13816530, "充电1"=13816530, "充电1"=13816530, "充电1"=13816530, "充电1"=13816530, "充电1"=13816530, "充电1"=13816530, "充电1"=13816530, "充电1"=13816530, "充电1"=13816530}, "1 40"={"充电1"=13816530, "充电1"=13816530, "充电1"=13816530, "充电1"=13816530, "充电1"=13816530, "充电1"=13816530, "充电1"=13816530, "充电1"=13816530, "充电1"=13816530, "充电1"=13816530, "充电1"=13816530, "充电1"=13816530}, "1 49"={"充电1"=13816530, "充电1"=13816530, "充电1"=13816530, "充电1"=13816530, "充电1"=13816530, "充电1"=13816530, "充电1"=13816530, "充电1"=13816530, "充电1"=13816530, "充电1"=13816530, "充电1"=13816530, "充电1"=13816530}, "1 14"={"均衡故障"=15, "均衡故障 2"=0.0, "均衡故障 3"=0.0, "均衡故障 4"=0.0, "均衡故障 5"=0.0, "均衡故障 6"=0.0, "均衡故障 7"=0.0, "均衡故障 8"=0.0, "均衡故障 9"=0.0, "均衡故障 10"=0.0, "均衡故障 11"=0.0, "均衡故障 12"=0.0}, "1 42"={"均衡故障"=15, "均衡故障 2"=0.0, "均衡故障 3"=0.0, "均衡故障 4"=0.0, "均衡故障 5"=0.0, "均衡故障 6"=0.0, "均衡故障 7"=0.0, "均衡故障 8"=0.0, "均衡故障 9"=0.0, "均衡故障 10"=0.0, "均衡故障 11"=0.0, "均衡故障 12"=0.0}, "1 34"={"均衡故障"=15, "均衡故障 2"=0.0, "均衡故障 3"=0.0, "均衡故障 4"=0.0, "均衡故障 5"=0.0, "均衡故障 6"=0.0, "均衡故障 7"=0.0, "均衡故障 8"=0.0, "均衡故障 9"=0.0, "均衡故障 10"=0.0, "均衡故障 11"=0.0, "均衡故障 12"=0.0}, "1 45"={"均衡故障"=15, "均衡故障 2"=0.0, "均衡故障 3"=0.0, "均衡故障 4"=0.0, "均衡故障 5"=0.0, "均衡故障 6"=0.0, "均衡故障 7"=0.0, "均衡故障 8"=0.0, "均衡故障 9"=0.0, "均衡故障 10"=0.0, "均衡故障 11"=0.0, "均衡故障 12"=0.0}, "1 17"={"均衡故障"=15, "均衡故障 2"=0.0, "均衡故障 3"=0.0, "均衡故障 4"=0.0, "均衡故障 5"=0.0, "均衡故障 6"=0.0, "均衡故障 7"=0.0, "均衡故障 8"=0.0, "均衡故障 9"=0.0, "均衡故障 10"=0.0, "均衡故障 11"=0.0, "均衡故障 12"=0.0}, "1 20"={"均衡故障"=15, "均衡故障 2"=0.0, "均衡故障 3"=0.0, "均衡故障 4"=0.0, "均衡故障 5"=0.0, "均衡故障 6"=0.0, "均衡故障 7"=0.0, "均衡故障 8"=0.0, "均衡故障 9"=0.0, "均衡故障 10"=0.0, "均衡故障 11"=0.0, "均衡故障 12"=0.0}, "1 39"={"均衡故障"=15, "均衡故障 2"=0.0, "均衡故障 3"=0.0, "均衡故障 4"=0.0, "均衡故障 5"=0.0, "均衡故障 6"=0.0, "均衡故障 7"=0.0, "均衡故障 8"=0.0, "均衡故障 9"=0.0, "均衡故障 10"=0.0, "均衡故障 11"=0.0, "均衡故障 12"=0.0}, "1 48"={"均衡故障"=15, "均衡故障 2"=0.0, "均衡故障 3"=0.0, "均衡故障 4"=0.0, "均衡故障 5"=0.0, "均衡故障 6"=0.0, "均衡故障 7"=0.0, "均衡故障 8"=0.0, "均衡故障 9"=0.0, "均衡故障 10"=0.0, "均衡故障 11"=0.0, "均衡故障 12"=0.0}} {"1 33"."第192串" format="%.3f"; "1 33"."第191串" format="%.3f"; "1 33"."第190串" format="%.3f"; "1 33"."第189串" format="%.3f"; "1 33"."第188串" format="%.3f"; "1 33"."第187串" format="%.3f"; "1 33"."第186串" format="%.3f"; "1 33"."第185串" format="%.3f"; "1 33"."第184串" format="%.3f"; "1 33"."第183串" format="%.3f"; "1 33"."第182串" format="%.3f"; "1 33"."第181串" format="%.3f"; "1 32"."第180串" format="%.3f"; "1 32"."第179串" format="%.3f"; "1 32"."第178串" format="%.3f"; "1 32"."第177串" format="%.3f"; "1 32"."第176串" format="%.3f"; "1 32"."第175串" format="%.3f"; "1 32"."第174串" format="%.3f"; "1 32"."第173串" format="%.3f"; "1 32"."第172串" format="%.3f"; "1 32"."第171串" format="%.3f"; "1 32"."第170串" format="%.3f"; "1 32"."第169串" format="%.3f"; "1 31"."第168串" format="%.3f"; "1 31"."第167串" format="%.3f"; "1 31"."第166串" format="%.3f"; "1 31"."第165串" format="%.3f"; "1 31"."第164串" format="%.3f"; "1 31"."第163串" format="%.3f"; "1 31"."第162串" format="%.3f"; "1 31"."第161串" format="%.3f"; "1 31"."第160串" format="%.3f"; "1 31"."第159串" format="%.3f"; "1 31"."第158串" format="%.3f"; "1 31"."第157串" format="%.3f"; "1 30"."第156串" format="%.3f"; "1 30"."第155串" format="%.3f"; "1 30"."第154串" format="%.3f"; "1 30"."第153串" format="%.3f"; "1 30"."第152串" format="%.3f"; "1 30"."第151串" format="%.3f"; "1 30"."第150串" format="%.3f"; "1 30"."第149串" format="%.3f"; "1 30"."第148串" format="%.3f"; "1 30"."第147串" format="%.3f"; "1 30"."第146串" format="%.3f"; "1 30"."第145串" format="%.3f"; "1 29"."第144串" format="%.3f"; "1 29"."第143串" format="%.3f"; "1 29"."第142串" format="%.3f"; "1 29"."第141串" format="%.3f"; "1 29"."第140串" format="%.3f"; "1 29"."第139串" format="%.3f"; "1 29"."第138串" format="%.3f"; "1 29"."第137串" format="%.3f"; "1 29"."第136串" format="%.3f"; "1 29"."第135串" format="%.3f"; "1 29"."第134串" format="%.3f"; "1 29"."第133串" format="%.3f"; "1 28"."第132串" format="%.3f"; "1 28"."第131串" format="%.3f"; "1 28"."第130串" format="%.3f"; "1 28"."第129串" format="%.3f"; "1 28"."第128串" format="%.3f"; "1 28"."第127串" format="%.3f"; "1 28"."第126串" format="%.3f"; "1 28"."第125串" format="%.3f"; "1 28"."第124串" format="%.3f"; "1 28"."第123串" format="%.3f"; "1 28"."第122串" format="%.3f"; "1 28"."第121串" format="%.3f"; "1 27"."第120串" format="%.3f"; "1 27"."第119串" format="%.3f"; "1 27"."第118串" format="%.3f"; "1 27"."第117串" format="%.3f"; "1 27"."第116串" format="%.3f"; "1 27"."第115串" format="%.3f"; "1 27"."第114串" format="%.3f"; "1 27"."第113串" format="%.3f"; "1 27"."第112串" format="%.3f"; "1 27"."第111串" format="%.3f"; "1 27"."第110串" format="%.3f"; "1 27"."第109串" format="%.3f"; "1 26"."第一串 24" format="%#.2f"; "1 26"."第108串" format="%.3f"; "1 26"."第一串 22" format="%#.2f"; "1 26"."第107串" format="%.3f"; "1 26"."第一串 20" format="%#.2f"; "1 26"."第106串" format="%.3f"; "1 26"."第一串 18" format="%#.2f"; "1 26"."第105串" format="%.3f"; "1 26"."第一串 16" format="%#.2f"; "1 26"."第104串" format="%.3f"; "1 26"."第一串 14" format="%#.2f"; "1 26"."第103串" format="%.3f"; "1 26"."第一串 12" format="%#.2f"; "1 26"."第102串" format="%.3f"; "1 26"."第一串 10" format="%#.2f"; "1 26"."第101串" format="%.3f"; "1 26"."第一串 8" format="%#.2f"; "1 26"."第100串" format="%.3f"; "1 26"."第一串 6" format="%#.2f"; "1 26"."第99串" format="%.3f"; "1 26"."第一串 4" format="%#.2f"; "1 26"."第98串" format="%.3f"; "1 26"."第一串 2" format="%#.2f"; "1 26"."第97串" format="%.3f"}
  out "3":T6={"1 18"={"第193串"=0.0, "第194串"=0.0, "第195串"=0.0, "第196串"=0.0, "第197串"=0.0, "第198串"=0.0, "第199串"=0.0, "第200串"=0.0, "第201串"=0.0, "第202串"=0.0, "第203串"=0.0, "第204串"=0.0, "第一串 2"=0.0, "第一串 4"=0.0, "第一串 6"=0.0, "第一串 8"=0.0, "第一串 10"=0.0, "第一串 12"=0.0, "第一串 14"=0.0, "第一串 16"=0.0, "第一串 18"=0.0, "第一串 20"=0.0, "第一串 22"=0.0, "第一串 24"=0.0}, "1 19"={"第205串"=0.0, "第206串"=0.0, "第207串"=0.0, "第208串"=0.0, "第209串"=0.0, "第210串"=0.0, "第211串"=0.0, "第212串"=0.0, "第213串"=0.0, "第214串"=0.0, "第215串"=0.0, "第216串"=0.0, "第一串 2"=0.0, "第一串 4"=0.0, "第一串 6"=0.0, "第一串 8"=0.0, "第一串 10"=0.0, "第一串 12"=0.0, "第一串 14"=0.0, "第一串 16"=0.0, "第一串 18"=0.0, "第一串 20"=0.0, "第一串 22"=0.0, "第一串 24"=0.0}, "1 20"={"第217串"=0.0, "第218串"=0.0, "第219串"=0.0, "第220串"=0.0, "第221串"=0.0, "第222串"=0.0, "第223串"=0.0, "第224串"=0.0, "第225串"=0.0, "第226串"=0.0, "第227串"=0.0, "第228串"=0.0, "第一串 2"=0.0, "第一串 4"=0.0, "第一串 6"=0.0, "第一串 8"=0.0, "第一串 10"=0.0, "第一串 12"=0.0, "第一串 14"=0.0, "第一串 16"=0.0, "第一串 18"=0.0, "第一串 20"=0.0, "第一串 22"=0.0, "第一串 24"=0.0}, "1 21"={"第229串"=0.0, "第230串"=0.0, "第231串"=0.0, "第232串"=0.0, "第233串"=0.0, "第234串"=0.0, "第235串"=0.0, "第236串"=0.0, "第237串"=0.0, "第238串"=0.0, "第239串"=0.0, "第240串"=0.0, "第一串 2"=0.0, "第一串 4"=0.0, "第一串 6"=0.0, "第一串 8"=0.0, "第一串 10"=0.0, "第一串 12"=0.0, "第一串 14"=0.0, "第一串 16"=0.0, "第一串 18"=0.0, "第一串 20"=0.0, "第一串 22"=0.0, "第一串 24"=0.0}, "1 22"={"第241串"=0.0, "第242串"=0.0, "第243串"=0.0, "第244串"=0.0, "第245串"=0.0, "第246串"=0.0, "第247串"=0.0, "第248串"=0.0, "第249串"=0.0, "第250串"=0.0, "第251串"=0.0, "第252串"=0.0, "第一串 2"=0.0, "第一串 4"=0.0, "第一串 6"=0.0, "第一串 8"=0.0, "第一串 10"=0.0, "第一串 12"=0.0, "第一串 14"=0.0, "第一串 16"=0.0, "第一串 18"=0.0, "第一串 20"=0.0, "第一串 22"=0.0, "第一串 24"=0.0}, "1 23"={"第253串"=0.0, "第254串"=0.0, "第255串"=0.0, "第256串"=0.0, "第257串"=0.0, "第258串"=0.0, "第259串"=0.0, "第260串"=0.0, "第261串"=0.0, "第262串"=0.0, "第263串"=0.0, "第264串"=0.0, "第一串 2"=0.0, "第一串 4"=0.0, "第一串 6"=0.0, "第一串 8"=0.0, "第一串 10"=0.0, "第一串 12"=0.0, "第一串 14"=0.0, "第一串 16"=0.0, "第一串 18"=0.0, "第一串 20"=0.0, "第一串 22"=0.0, "第一串 24"=0.0}, "1 24"={"第265串"=0.0, "第266串"=0.0, "第267串"=0.0, "第268串"=0.0, "第269串"=0.0, "第270串"=0.0, "第271串"=0.0, "第272串"=0.0, "第273串"=0.0, "第274串"=0.0, "第275串"=0.0, "第276串"=0.0, "第一串 2"=0.0, "第一串 4"=0.0, "第一串 6"=0.0, "第一串 8"=0.0, "第一串 10"=0.0, "第一串 12"=0.0, "第一串 14"=0.0, "第一串 16"=0.0, "第一串 18"=0.0, "第一串 20"=0.0, "第一串 22"=0.0, "第一串 24"=0.0}, "1 25"={"第277串"=0.0, "第278串"=0.0, "第279串"=0.0, "第280串"=0.0, "第281串"=0.0, "第282串"=0.0, "第283串"=0.0, "第284串"=0.0, "第285串"=0.0, "第286串"=0.0, "第287串"=0.0, "第288串"=0.0, "第一串 2"=0.0, "第一串 4"=0.0, "第一串 6"=0.0, "第一串 8"=0.0, "第一串 10"=0.0, "第一串 12"=0.0, "第一串 14"=0.0, "第一串 16"=0.0, "第一串 18"=0.0, "第一串 20"=0.0, "第一串 22"=0.0, "第一串 24"=0.0}, "1 12"={"充电1"=13816530, "充电1"=13816530, "充电1"=13816530, "充电1"=13816530, "充电1"=13816530, "充电1"=13816530, "充电1"=13816530, "充电1"=13816530, "充电1"=13816530, "充电1"=13816530, "充电1"=13816530, "充电1"=13816530}, "1 39"={"充电1"=13816530, "充电1"=13816530, "充电1"=13816530, "充电1"=13816530, "充电1"=13816530, "充电1"=13816530, "充电1"=13816530, "充电1"=13816530, "充电1"=13816530, "充电1"=13816530, "充电1"=13816530, "充电1"=13816530}, "1 28"={"充电1"=13816530, "充电1"=13816530, "充电1"=13816530, "充电1"=13816530, "充电1"=13816530, "充电1"=13816530, "充电1"=13816530, "充电1"=13816530, "充电1"=13816530, "充电1"=13816530, "充电1"=13816530, "充电1"=13816530}, "1 42"={"充电1"=13816530, "充电1"=13816530, "充电1"=13816530, "充电1"=13816530, "充电1"=13816530, "充电1"=13816530, "充电1"=13816530, "充电1"=13816530, "充电1"=13816530, "充电1"=13816530, "充电1"=13816530, "充电1"=13816530}, "1 16"={"充电1"=13816530, "充电1"=13816530, "充电1"=13816530, "充电1"=13816530, "充电1"=13816530, "充电1"=13816530, "充电1"=13816530, "充电1"=13816530, "充电1"=13816530, "充电1"=13816530, "充电1"=13816530, "充电1"=13816530}, "1 30"={"充电1"=13816530, "充电1"=13816530, "充电1"=13816530, "充电1"=13816530, "充电1"=13816530, "充电1"=13816530, "充电1"=13816530, "充电1"=13816530, "充电1"=13816530, "充电1"=13816530, "充电1"=13816530, "充电1"=13816530}, "1 33"={"充电1"=13816530, "充电1"=13816530, "充电1"=13816530, "充电1"=13816530, "充电1"=13816530, "充电1"=13816530, "充电1"=13816530, "充电1"=13816530, "充电1"=13816530, "充电1"=13816530, "充电1"=13816530, "充电1"=13816530}, "1 36"={"充电1"=13816530, "充电1"=13816530, "充电1"=13816530, "充电1"=13816530, "充电1"=13816530, "充电1"=13816530, "充电1"=13816530, "充电1"=13816530, "充电1"=13816530, "充电1"=13816530, "充电1"=13816530, "充电1"=13816530}, "1 11"={"充电1"=13816530, "充电1"=13816530, "充电1"=13816530, "充电1"=13816530, "充电1"=13816530, "充电1"=13816530, "充电1"=13816530, "充电1"=13816530, "充电1"=13816530, "充电1"=13816530, "充电1"=13816530, "充电1"=13816530}, "1 38"={"充电1"=13816530, "充电1"=13816530, "充电1"=13816530, "充电1"=13816530, "充电1"=13816530, "充电1"=13816530, "充电1"=13816530, "充电1"=13816530, "充电1"=13816530, "充电1"=13816530, "充电1"=13816530, "充电1"=13816530}, "1 27"={"充电1"=13816530, "充电1"=13816530, "充电1"=13816530, "充电1"=13816530, "充电1"=13816530, "充电1"=13816530, "充电1"=13816530, "充电1"=13816530, "充电1"=13816530, "充电1"=13816530, "充电1"=13816530, "充电1"=13816530}, "1 41"={"充电1"=13816530, "充电1"=13816530, "充电1"=13816530, "充电1"=13816530, "充电1"=13816530, "充电1"=13816530, "充电1"=13816530, "充电1"=13816530, "充电1"=13816530, "充电1"=13816530, "充电1"=13816530, "充电1"=13816530}, "1 15"={"充电1"=13816530, "充电1"=13816530, "充电1"=13816530, "充电1"=13816530, "充电1"=13816530, "充电1"=13816530, "充电1"=13816530, "充电1"=13816530, "充电1"=13816530, "充电1"=13816530, "充电1"=13816530, "充电1"=13816530}, "1 29"={"充电1"=13816530, "充电1"=13816530, "充电1"=13816530, "充电1"=13816530, "充电1"=13816530, "充电1"=13816530, "充电1"=13816530, "充电1"=13816530, "充电1"=13816530, "充电1"=13816530, "充电1"=13816530, "充电1"=13816530}, "1 32"={"充电1"=13816530, "充电1"=13816530, "充电1"=13816530, "充电1"=13816530, "充电1"=13816530, "充电1"=13816530, "充电1"=13816530, "充电1"=13816530, "充电1"=13816530, "充电1"=13816530, "充电1"=13816530, "充电1"=13816530}, "1 35"={"充电1"=13816530, "充电1"=13816530, "充电1"=13816530, "充电1"=13816530, "充电1"=13816530, "充电1"=13816530, "充电1"=13816530, "充电1"=13816530, "充电1"=13816530, "充电1"=13816530, "充电1"=13816530, "充电1"=13816530}, "1 13"={"均衡故障"=0, "均衡故障 2"=0.0, "均衡故障 3"=0.0, "均衡故障 4"=0.0, "均衡故障 5"=0.0, "均衡故障 6"=0.0, "均衡故障 7"=0.0, "均衡故障 8"=0.0, "均衡故障 9"=0.0, "均衡故障 10"=0.0, "均衡故障 11"=0.0, "均衡故障 12"=0.0}, "1 37"={"均衡故障"=0, "均衡故障 2"=0.0, "均衡故障 3"=0.0, "均衡故障 4"=0.0, "均衡故障 5"=0.0, "均衡故障 6"=0.0, "均衡故障 7"=0.0, "均衡故障 8"=0.0, "均衡故障 9"=0.0, "均衡故障 10"=0.0, "均衡故障 11"=0.0, "均衡故障 12"=0.0}, "1 26"={"均衡故障"=0, "均衡故障 2"=0.0, "均衡故障 3"=0.0, "均衡故障 4"=0.0, "均衡故障 5"=0.0, "均衡故障 6"=0.0, "均衡故障 7"=0.0, "均衡故障 8"=0.0, "均衡故障 9"=0.0, "均衡故障 10"=0.0, "均衡故障 11"=0.0, "均衡故障 12"=0.0}, "1 40"={"均衡故障"=0, "均衡故障 2"=0.0, "均衡故障 3"=0.0, "均衡故障 4"=0.0, "均衡故障 5"=0.0, "均衡故障 6"=0.0, "均衡故障 7"=0.0, "均衡故障 8"=0.0, "均衡故障 9"=0.0, "均衡故障 10"=0.0, "均衡故障 11"=0.0, "均衡故障 12"=0.0}, "1 14"={"均衡故障"=0, "均衡故障 2"=0.0, "均衡故障 3"=0.0, "均衡故障 4"=0.0, "均衡故障 5"=0.0, "均衡故障 6"=0.0, "均衡故障 7"=0.0, "均衡故障 8"=0.0, "均衡故障 9"=0.0, "均衡故障 10"=0.0, "均衡故障 11"=0.0, "均衡故障 12"=0.0}, "1 17"={"均衡故障"=0, "均衡故障 2"=0.0, "均衡故障 3"=0.0, "均衡故障 4"=0.0, "均衡故障 5"=0.0, "均衡故障 6"=0.0, "均衡故障 7"=0.0, "均衡故障 8"=0.0, "均衡故障 9"=0.0, "均衡故障 10"=0.0, "均衡故障 11"=0.0, "均衡故障 12"=0.0}, "1 31"={"均衡故障"=0, "均衡故障 2"=0.0, "均衡故障 3"=0.0, "均衡故障 4"=0.0, "均衡故障 5"=0.0, "均衡故障 6"=0.0, "均衡故障 7"=0.0, "均衡故障 8"=0.0, "均衡故障 9"=0.0, "均衡故障 10"=0.0, "均衡故障 11"=0.0, "均衡故障 12"=0.0}, "1 34"={"均衡故障"=0, "均衡故障 2"=0.0, "均衡故障 3"=0.0, "均衡故障 4"=0.0, "均衡故障 5"=0.0, "均衡故障 6"=0.0, "均衡故障 7"=0.0, "均衡故障 8"=0.0, "均衡故障 9"=0.0, "均衡故障 10"=0.0, "均衡故障 11"=0.0, "均衡故障 12"=0.0}} {"1 25"."第288串" format="%.3f"; "1 25"."第287串" format="%.3f"; "1 25"."第286串" format="%.3f"; "1 25"."第285串" format="%.3f"; "1 25"."第284串" format="%.3f"; "1 25"."第283串" format="%.3f"; "1 25"."第282串" format="%.3f"; "1 25"."第281串" format="%.3f"; "1 25"."第280串" format="%.3f"; "1 25"."第279串" format="%.3f"; "1 25"."第278串" format="%.3f"; "1 25"."第277串" format="%.3f"; "1 24"."第276串" format="%.3f"; "1 24"."第275串" format="%.3f"; "1 24"."第274串" format="%.3f"; "1 24"."第273串" format="%.3f"; "1 24"."第272串" format="%.3f"; "1 24"."第271串" format="%.3f"; "1 24"."第270串" format="%.3f"; "1 24"."第269串" format="%.3f"; "1 24"."第268串" format="%.3f"; "1 24"."第267串" format="%.3f"; "1 24"."第266串" format="%.3f"; "1 24"."第265串" format="%.3f"; "1 23"."第264串" format="%.3f"; "1 23"."第263串" format="%.3f"; "1 23"."第262串" format="%.3f"; "1 23"."第261串" format="%.3f"; "1 23"."第260串" format="%.3f"; "1 23"."第259串" format="%.3f"; "1 23"."第258串" format="%.3f"; "1 23"."第257串" format="%.3f"; "1 23"."第256串" format="%.3f"; "1 23"."第255串" format="%.3f"; "1 23"."第254串" format="%.3f"; "1 23"."第253串" format="%.3f"; "1 22"."第252串" format="%.3f"; "1 22"."第251串" format="%.3f"; "1 22"."第250串" format="%.3f"; "1 22"."第249串" format="%.3f"; "1 22"."第248串" format="%.3f"; "1 22"."第247串" format="%.3f"; "1 22"."第246串" format="%.3f"; "1 22"."第245串" format="%.3f"; "1 22"."第244串" format="%.3f"; "1 22"."第243串" format="%.3f"; "1 22"."第242串" format="%.3f"; "1 22"."第241串" format="%.3f"; "1 21"."第240串" format="%.3f"; "1 21"."第239串" format="%.3f"; "1 21"."第238串" format="%.3f"; "1 21"."第237串" format="%.3f"; "1 21"."第236串" format="%.3f"; "1 21"."第235串" format="%.3f"; "1 21"."第234串" format="%.3f"; "1 21"."第233串" format="%.3f"; "1 21"."第232串" format="%.3f"; "1 21"."第231串" format="%.3f"; "1 21"."第230串" format="%.3f"; "1 21"."第229串" format="%.3f"; "1 20"."第228串" format="%.3f"; "1 20"."第227串" format="%.3f"; "1 20"."第226串" format="%.3f"; "1 20"."第225串" format="%.3f"; "1 20"."第224串" format="%.3f"; "1 20"."第223串" format="%.3f"; "1 20"."第222串" format="%.3f"; "1 20"."第221串" format="%.3f"; "1 20"."第220串" format="%.3f"; "1 20"."第219串" format="%.3f"; "1 20"."第218串" format="%.3f"; "1 20"."第217串" format="%.3f"; "1 19"."第216串" format="%.3f"; "1 19"."第215串" format="%.3f"; "1 19"."第214串" format="%.3f"; "1 19"."第213串" format="%.3f"; "1 19"."第212串" format="%.3f"; "1 19"."第211串" format="%.3f"; "1 19"."第210串" format="%.3f"; "1 19"."第209串" format="%.3f"; "1 19"."第208串" format="%.3f"; "1 19"."第207串" format="%.3f"; "1 19"."第206串" format="%.3f"; "1 19"."第205串" format="%.3f"; "1 18"."第一串 24" format="%#.2f"; "1 18"."第204串" format="%.3f"; "1 18"."第一串 22" format="%#.2f"; "1 18"."第203串" format="%.3f"; "1 18"."第一串 20" format="%#.2f"; "1 18"."第202串" format="%.3f"; "1 18"."第一串 18" format="%#.2f"; "1 18"."第201串" format="%.3f"; "1 18"."第一串 16" format="%#.2f"; "1 18"."第200串" format="%.3f"; "1 18"."第一串 14" format="%#.2f"; "1 18"."第199串" format="%.3f"; "1 18"."第一串 12" format="%#.2f"; "1 18"."第198串" format="%.3f"; "1 18"."第一串 10" format="%#.2f"; "1 18"."第197串" format="%.3f"; "1 18"."第一串 8" format="%#.2f"; "1 18"."第196串" format="%.3f"; "1 18"."第一串 6" format="%#.2f"; "1 18"."第195串" format="%.3f"; "1 18"."第一串 4" format="%#.2f"; "1 18"."第194串" format="%.3f"; "1 18"."第一串 2" format="%#.2f"; "1 18"."第193串" format="%.3f"}
  out "1 5":T7 {"第一串 24" format="%#.2f"; "第300串" format="%.3f"; "第一串 22" format="%#.2f"; "第299串" format="%.3f"; "第一串 20" format="%#.2f"; "第298串" format="%.3f"; "第一串 18" format="%#.2f"; "第297串" format="%.3f"; "第一串 16" format="%#.2f"; "第296串" format="%.3f"; "第一串 14" format="%#.2f"; "第295串" format="%.3f"; "第一串 12" format="%#.2f"; "第294串" format="%.3f"; "第一串 10" format="%#.2f"; "第293串" format="%.3f"; "第一串 8" format="%#.2f"; "第292串" format="%.3f"; "第一串 6" format="%#.2f"; "第291串" format="%.3f"; "第一串 4" format="%#.2f"; "第290串" format="%.3f"; "第一串 2" format="%#.2f"; "第289串" format="%.3f"}
  out "1 13":T8
  out "放电均衡":T9={"充电1"=13816530, "充电1"=13816530, "充电1"=13816530, "充电1"=13816530, "充电1"=13816530, "充电1"=13816530, "充电1"=13816530, "充电1"=13816530, "充电1"=13816530, "充电1"=13816530, "充电1"=13816530, "充电1"=13816530}
  out "充电均衡":T9={"充电1"=13816530, "充电1"=13816530, "充电1"=13816530, "充电1"=13816530, "充电1"=13816530, "充电1"=13816530, "充电1"=13816530, "充电1"=13816530, "充电1"=13816530, "充电1"=13816530, "充电1"=13816530, "充电1"=13816530}
  out "放电均衡":u32(colorbox)=6618880
  out "充电均衡":u32(colorbox)=16860
  in  "布尔":bool caption="判定"
  in  "故障信息选择按键 3":enum32{"单选选项2", "单选选项2 2", "单选选项2 3", "单选选项1"}(radio)=enum."单选选项1"
  out "电压选择 2":enum32{"1-96", "97-192", "193-288", "289-300"}(tab)
  out "4":T10 {"1 102"."第一串 24" format="%#.2f"; "1 102"."第12串" format="%#.2f"; "1 102"."第一串 22" format="%#.2f"; "1 102"."第11串" format="%#.2f"; "1 102"."第一串 20" format="%#.2f"; "1 102"."第10串" format="%#.2f"; "1 102"."第一串 18" format="%#.2f"; "1 102"."第9串" format="%#.2f"; "1 102"."第一串 16" format="%#.2f"; "1 102"."第8串" format="%#.2f"; "1 102"."第一串 14" format="%#.2f"; "1 102"."第7串" format="%#.2f"; "1 102"."第一串 12" format="%#.2f"; "1 102"."第6串" format="%#.2f"; "1 102"."第一串 10" format="%#.2f"; "1 102"."第5串" format="%#.2f"; "1 102"."第一串 8" format="%#.2f"; "1 102"."第4串" format="%#.2f"; "1 102"."第一串 6" format="%#.2f"; "1 102"."第3串" format="%#.2f"; "1 102"."第一串 4" format="%#.2f"; "1 102"."第2串" format="%#.2f"; "1 102"."第一串 2" format="%#.2f"; "1 102"."第1串" format="%#.2f"}
  out "5":T11 {"1 26"."第一串 24" format="%#.2f"; "1 26"."第108串" format="%#.2f"; "1 26"."第一串 22" format="%#.2f"; "1 26"."第107串" format="%#.2f"; "1 26"."第一串 20" format="%#.2f"; "1 26"."第106串" format="%#.2f"; "1 26"."第一串 18" format="%#.2f"; "1 26"."第105串" format="%#.2f"; "1 26"."第一串 16" format="%#.2f"; "1 26"."第104串" format="%#.2f"; "1 26"."第一串 14" format="%#.2f"; "1 26"."第103串" format="%#.2f"; "1 26"."第一串 12" format="%#.2f"; "1 26"."第102串" format="%#.2f"; "1 26"."第一串 10" format="%#.2f"; "1 26"."第101串" format="%#.2f"; "1 26"."第一串 8" format="%#.2f"; "1 26"."第100串" format="%#.2f"; "1 26"."第一串 6" format="%#.2f"; "1 26"."第99串" format="%#.2f"; "1 26"."第一串 4" format="%#.2f"; "1 26"."第98串" format="%#.2f"; "1 26"."第一串 2" format="%#.2f"; "1 26"."第97串" format="%#.2f"}
  out "6":T12 {"1 18"."第一串 24" format="%#.2f"; "1 18"."第204串" format="%#.2f"; "1 18"."第一串 22" format="%#.2f"; "1 18"."第203串" format="%#.2f"; "1 18"."第一串 20" format="%#.2f"; "1 18"."第202串" format="%#.2f"; "1 18"."第一串 18" format="%#.2f"; "1 18"."第201串" format="%#.2f"; "1 18"."第一串 16" format="%#.2f"; "1 18"."第200串" format="%#.2f"; "1 18"."第一串 14" format="%#.2f"; "1 18"."第199串" format="%#.2f"; "1 18"."第一串 12" format="%#.2f"; "1 18"."第198串" format="%#.2f"; "1 18"."第一串 10" format="%#.2f"; "1 18"."第197串" format="%#.2f"; "1 18"."第一串 8" format="%#.2f"; "1 18"."第196串" format="%#.2f"; "1 18"."第一串 6" format="%#.2f"; "1 18"."第195串" format="%#.2f"; "1 18"."第一串 4" format="%#.2f"; "1 18"."第194串" format="%#.2f"; "1 18"."第一串 2" format="%#.2f"; "1 18"."第193串" format="%#.2f"}
  out "1 6":T7 {"第一串 24" format="%#.2f"; "第300串" format="%#.2f"; "第一串 22" format="%#.2f"; "第299串" format="%#.2f"; "第一串 20" format="%#.2f"; "第298串" format="%#.2f"; "第一串 18" format="%#.2f"; "第297串" format="%#.2f"; "第一串 16" format="%#.2f"; "第296串" format="%#.2f"; "第一串 14" format="%#.2f"; "第295串" format="%#.2f"; "第一串 12" format="%#.2f"; "第294串" format="%#.2f"; "第一串 10" format="%#.2f"; "第293串" format="%#.2f"; "第一串 8" format="%#.2f"; "第292串" format="%#.2f"; "第一串 6" format="%#.2f"; "第291串" format="%#.2f"; "第一串 4" format="%#.2f"; "第290串" format="%#.2f"; "第一串 2" format="%#.2f"; "第289串" format="%#.2f"}
  in  "偏差":dbl=2.0 format="%#.0f"
  in  "基准":dbl=25.0 format="%#.0f"
  in  "布尔 2":bool caption="判定"
  in  "故障信息选择按键 4":enum32{"单选选项2", "单选选项2 2", "单选选项2 3", "单选选项1"}(radio)=enum."单选选项1"
  out "电压选择 3":enum32{"1-96", "97-192", "193-288", "289-300"}(tab)
  out "1 106":T13 {"1 102"."第一串 24" format="%#.2f"; "1 102"."第12串" format="%#.2f"; "1 102"."第一串 22" format="%#.2f"; "1 102"."第11串" format="%#.2f"; "1 102"."第一串 20" format="%#.2f"; "1 102"."第10串" format="%#.2f"; "1 102"."第一串 18" format="%#.2f"; "1 102"."第9串" format="%#.2f"; "1 102"."第一串 16" format="%#.2f"; "1 102"."第8串" format="%#.2f"; "1 102"."第一串 14" format="%#.2f"; "1 102"."第7串" format="%#.2f"; "1 102"."第一串 12" format="%#.2f"; "1 102"."第6串" format="%#.2f"; "1 102"."第一串 10" format="%#.2f"; "1 102"."第5串" format="%#.2f"; "1 102"."第一串 8" format="%#.2f"; "1 102"."第4串" format="%#.2f"; "1 102"."第一串 6" format="%#.2f"; "1 102"."第3串" format="%#.2f"; "1 102"."第一串 4" format="%#.2f"; "1 102"."第2串" format="%#.2f"; "1 102"."第一串 2" format="%#.2f"; "1 102"."第1串" format="%#.2f"}
  out "1 107":T11 {"1 26"."第一串 24" format="%#.2f"; "1 26"."第108串" format="%#.2f"; "1 26"."第一串 22" format="%#.2f"; "1 26"."第107串" format="%#.2f"; "1 26"."第一串 20" format="%#.2f"; "1 26"."第106串" format="%#.2f"; "1 26"."第一串 18" format="%#.2f"; "1 26"."第105串" format="%#.2f"; "1 26"."第一串 16" format="%#.2f"; "1 26"."第104串" format="%#.2f"; "1 26"."第一串 14" format="%#.2f"; "1 26"."第103串" format="%#.2f"; "1 26"."第一串 12" format="%#.2f"; "1 26"."第102串" format="%#.2f"; "1 26"."第一串 10" format="%#.2f"; "1 26"."第101串" format="%#.2f"; "1 26"."第一串 8" format="%#.2f"; "1 26"."第100串" format="%#.2f"; "1 26"."第一串 6" format="%#.2f"; "1 26"."第99串" format="%#.2f"; "1 26"."第一串 4" format="%#.2f"; "1 26"."第98串" format="%#.2f"; "1 26"."第一串 2" format="%#.2f"; "1 26"."第97串" format="%#.2f"}
  out "1 28":T12 {"1 18"."第一串 24" format="%#.2f"; "1 18"."第204串" format="%#.2f"; "1 18"."第一串 22" format="%#.2f"; "1 18"."第203串" format="%#.2f"; "1 18"."第一串 20" format="%#.2f"; "1 18"."第202串" format="%#.2f"; "1 18"."第一串 18" format="%#.2f"; "1 18"."第201串" format="%#.2f"; "1 18"."第一串 16" format="%#.2f"; "1 18"."第200串" format="%#.2f"; "1 18"."第一串 14" format="%#.2f"; "1 18"."第199串" format="%#.2f"; "1 18"."第一串 12" format="%#.2f"; "1 18"."第198串" format="%#.2f"; "1 18"."第一串 10" format="%#.2f"; "1 18"."第197串" format="%#.2f"; "1 18"."第一串 8" format="%#.2f"; "1 18"."第196串" format="%#.2f"; "1 18"."第一串 6" format="%#.2f"; "1 18"."第195串" format="%#.2f"; "1 18"."第一串 4" format="%#.2f"; "1 18"."第194串" format="%#.2f"; "1 18"."第一串 2" format="%#.2f"; "1 18"."第193串" format="%#.2f"}
  out "1 7":T7 {"第一串 24" format="%#.2f"; "第300串" format="%#.2f"; "第一串 22" format="%#.2f"; "第299串" format="%#.2f"; "第一串 20" format="%#.2f"; "第298串" format="%#.2f"; "第一串 18" format="%#.2f"; "第297串" format="%#.2f"; "第一串 16" format="%#.2f"; "第296串" format="%#.2f"; "第一串 14" format="%#.2f"; "第295串" format="%#.2f"; "第一串 12" format="%#.2f"; "第294串" format="%#.2f"; "第一串 10" format="%#.2f"; "第293串" format="%#.2f"; "第一串 8" format="%#.2f"; "第292串" format="%#.2f"; "第一串 6" format="%#.2f"; "第291串" format="%#.2f"; "第一串 4" format="%#.2f"; "第290串" format="%#.2f"; "第一串 2" format="%#.2f"; "第289串" format="%#.2f"}
  in  "故障信息选择按键 5":enum32{"单选选项2", "单选选项2 2", "单选选项2 3", "单选选项1"}(radio)=enum."单选选项1"
  out "电压选择 4":enum32{"1-96", "97-192", "193-288", "289-300"}(tab)
  out "1 108":T13 {"1 102"."第一串 24" format="%#.2f"; "1 102"."第12串" format="%#.2f"; "1 102"."第一串 22" format="%#.2f"; "1 102"."第11串" format="%#.2f"; "1 102"."第一串 20" format="%#.2f"; "1 102"."第10串" format="%#.2f"; "1 102"."第一串 18" format="%#.2f"; "1 102"."第9串" format="%#.2f"; "1 102"."第一串 16" format="%#.2f"; "1 102"."第8串" format="%#.2f"; "1 102"."第一串 14" format="%#.2f"; "1 102"."第7串" format="%#.2f"; "1 102"."第一串 12" format="%#.2f"; "1 102"."第6串" format="%#.2f"; "1 102"."第一串 10" format="%#.2f"; "1 102"."第5串" format="%#.2f"; "1 102"."第一串 8" format="%#.2f"; "1 102"."第4串" format="%#.2f"; "1 102"."第一串 6" format="%#.2f"; "1 102"."第3串" format="%#.2f"; "1 102"."第一串 4" format="%#.2f"; "1 102"."第2串" format="%#.2f"; "1 102"."第一串 2" format="%#.2f"; "1 102"."第1串" format="%#.2f"}
  out "1 109":T11 {"1 26"."第一串 24" format="%#.2f"; "1 26"."第108串" format="%#.2f"; "1 26"."第一串 22" format="%#.2f"; "1 26"."第107串" format="%#.2f"; "1 26"."第一串 20" format="%#.2f"; "1 26"."第106串" format="%#.2f"; "1 26"."第一串 18" format="%#.2f"; "1 26"."第105串" format="%#.2f"; "1 26"."第一串 16" format="%#.2f"; "1 26"."第104串" format="%#.2f"; "1 26"."第一串 14" format="%#.2f"; "1 26"."第103串" format="%#.2f"; "1 26"."第一串 12" format="%#.2f"; "1 26"."第102串" format="%#.2f"; "1 26"."第一串 10" format="%#.2f"; "1 26"."第101串" format="%#.2f"; "1 26"."第一串 8" format="%#.2f"; "1 26"."第100串" format="%#.2f"; "1 26"."第一串 6" format="%#.2f"; "1 26"."第99串" format="%#.2f"; "1 26"."第一串 4" format="%#.2f"; "1 26"."第98串" format="%#.2f"; "1 26"."第一串 2" format="%#.2f"; "1 26"."第97串" format="%#.2f"}
  out "1 29":T12 {"1 18"."第一串 24" format="%#.2f"; "1 18"."第204串" format="%#.2f"; "1 18"."第一串 22" format="%#.2f"; "1 18"."第203串" format="%#.2f"; "1 18"."第一串 20" format="%#.2f"; "1 18"."第202串" format="%#.2f"; "1 18"."第一串 18" format="%#.2f"; "1 18"."第201串" format="%#.2f"; "1 18"."第一串 16" format="%#.2f"; "1 18"."第200串" format="%#.2f"; "1 18"."第一串 14" format="%#.2f"; "1 18"."第199串" format="%#.2f"; "1 18"."第一串 12" format="%#.2f"; "1 18"."第198串" format="%#.2f"; "1 18"."第一串 10" format="%#.2f"; "1 18"."第197串" format="%#.2f"; "1 18"."第一串 8" format="%#.2f"; "1 18"."第196串" format="%#.2f"; "1 18"."第一串 6" format="%#.2f"; "1 18"."第195串" format="%#.2f"; "1 18"."第一串 4" format="%#.2f"; "1 18"."第194串" format="%#.2f"; "1 18"."第一串 2" format="%#.2f"; "1 18"."第193串" format="%#.2f"}
  out "1 8":T7 {"第一串 24" format="%#.2f"; "第300串" format="%#.2f"; "第一串 22" format="%#.2f"; "第299串" format="%#.2f"; "第一串 20" format="%#.2f"; "第298串" format="%#.2f"; "第一串 18" format="%#.2f"; "第297串" format="%#.2f"; "第一串 16" format="%#.2f"; "第296串" format="%#.2f"; "第一串 14" format="%#.2f"; "第295串" format="%#.2f"; "第一串 12" format="%#.2f"; "第294串" format="%#.2f"; "第一串 10" format="%#.2f"; "第293串" format="%#.2f"; "第一串 8" format="%#.2f"; "第292串" format="%#.2f"; "第一串 6" format="%#.2f"; "第291串" format="%#.2f"; "第一串 4" format="%#.2f"; "第290串" format="%#.2f"; "第一串 2" format="%#.2f"; "第289串" format="%#.2f"}
  out "单选选项2":bool
  # "主板详细信息"
  # "主板详细信息"
  # "监控上位机"
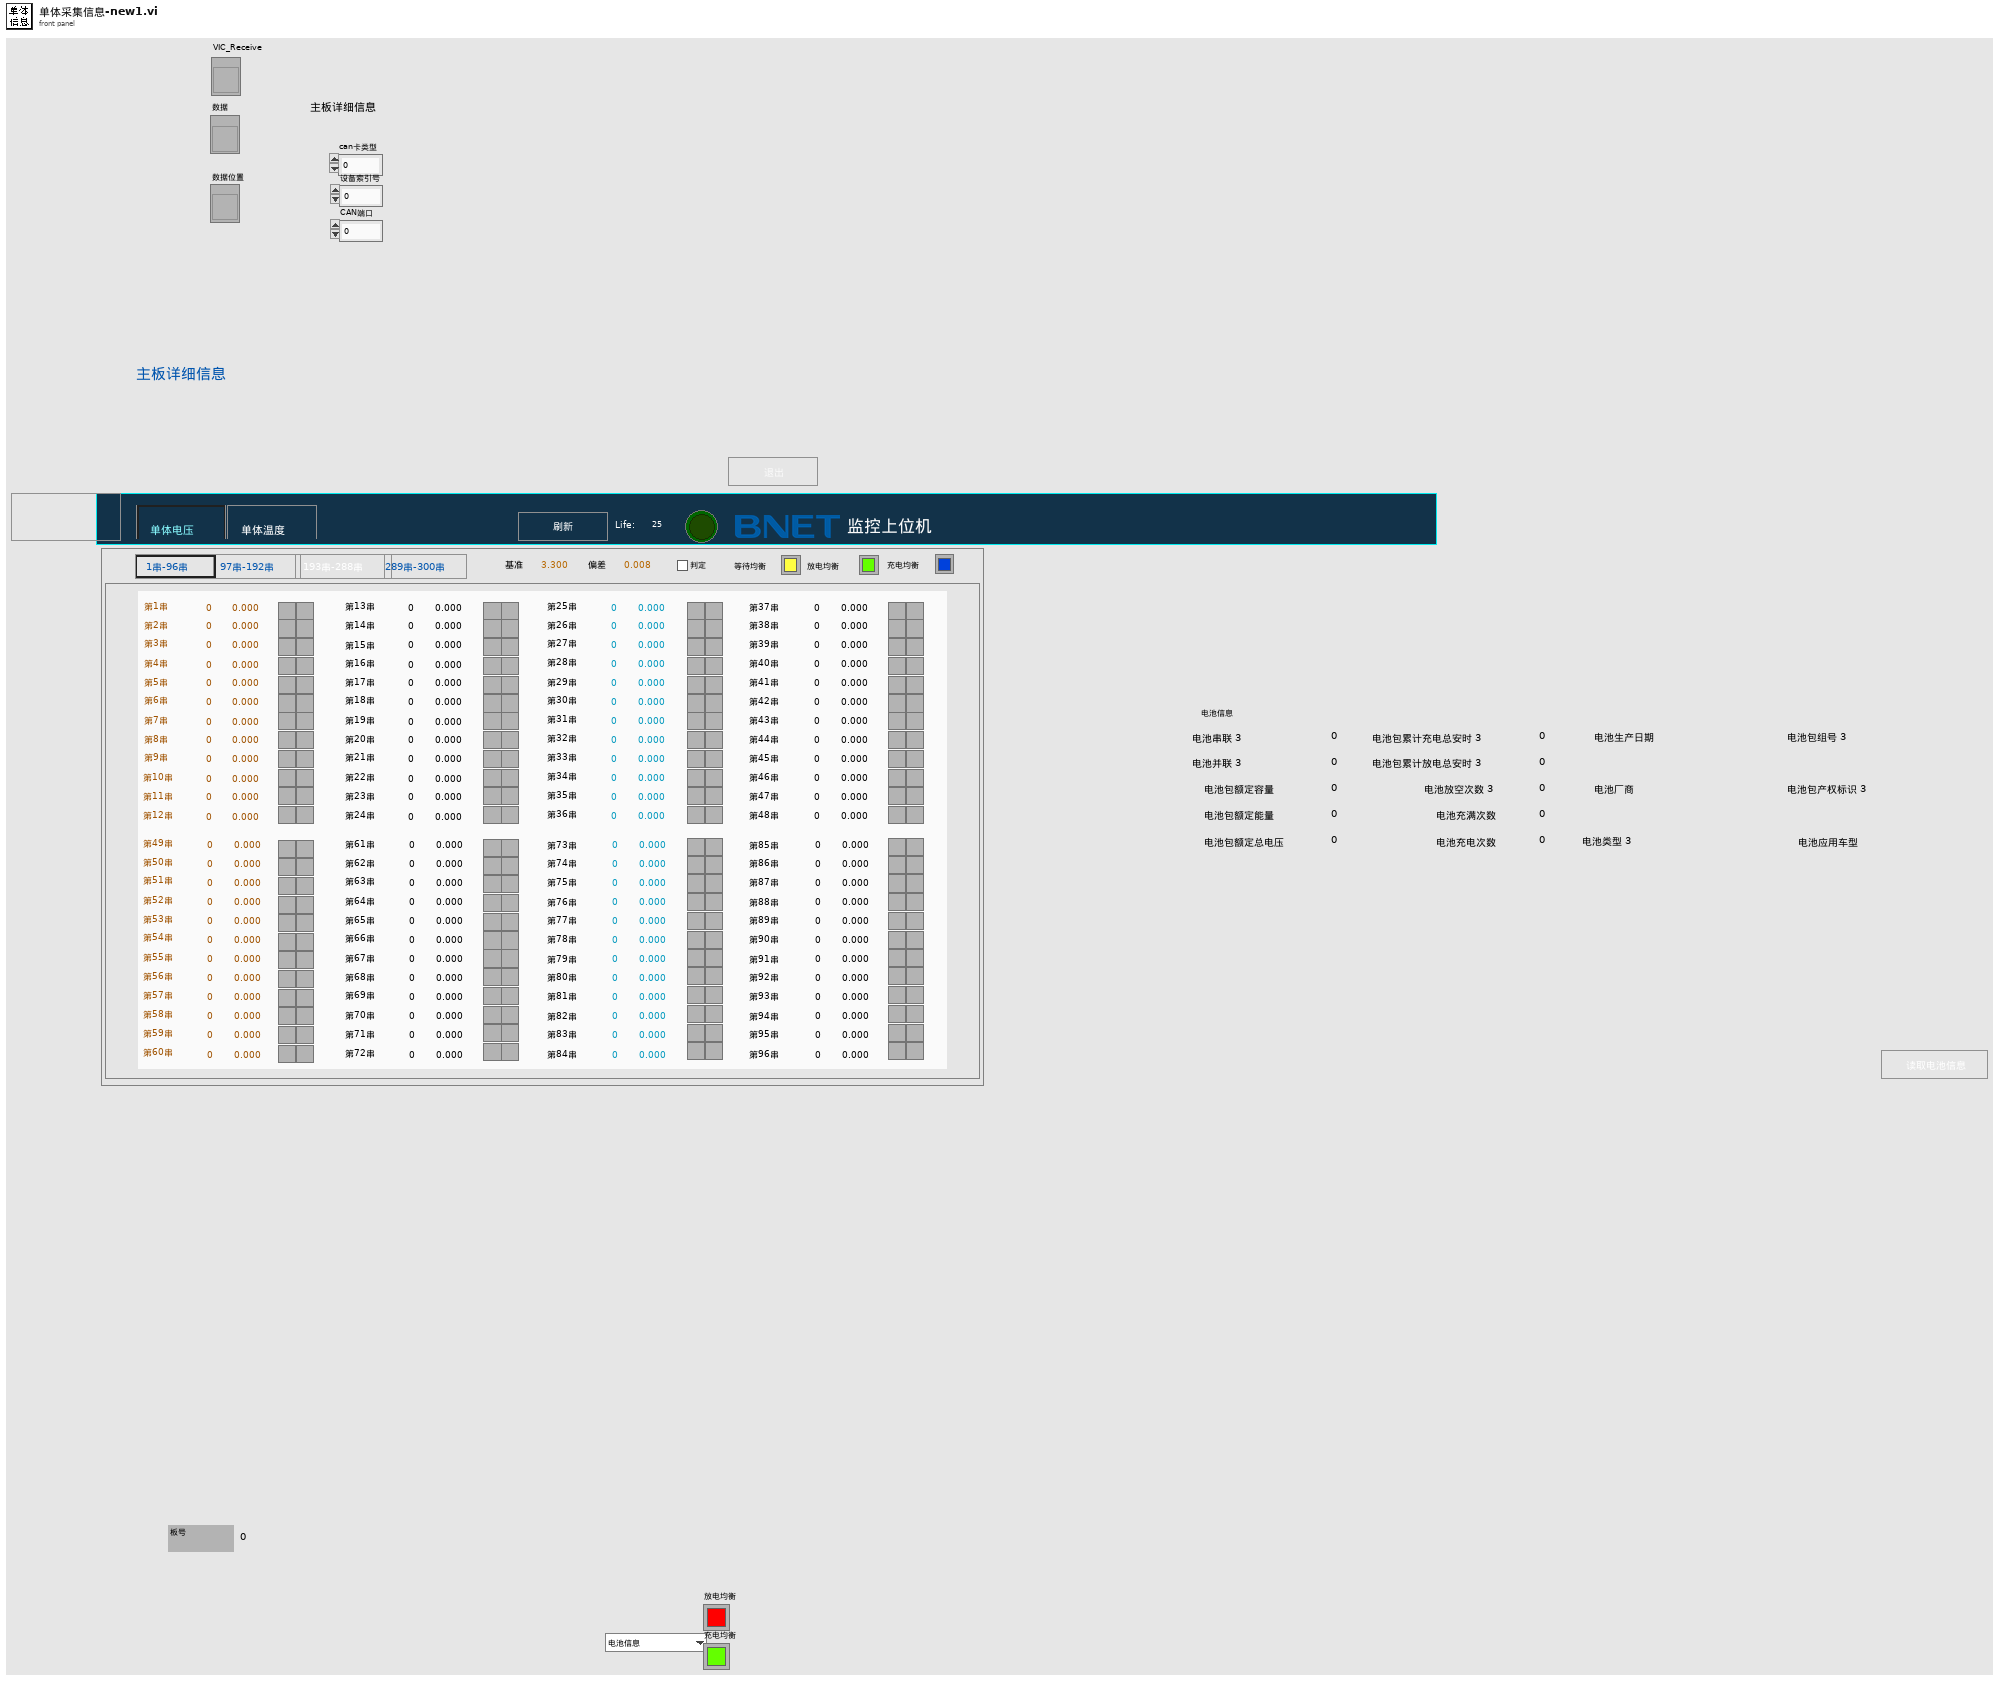
[diagram p1: front panel]
types:
  T1 = cluster{"ID":u32, "TimeStamp":u32, "TimeFlag":u8, "SendType":u8, "RemoteFlag":u8, "ExternFlag":u8, "DataLen":u8, "Data1":u8, "Data2":u8, "Data3":u8, "Data4":u8, "Data5":u8, "Data6":u8, "Data7":u8, "Data8":u8, "Rsv1":u8, "Rsv2":u8, "Rsv3":u8}
  T2 = cluster{"电池串联 3":dbl, "电池并联 3":dbl, "电池包累计放电总安时 3":dbl, "电池包额定容量":dbl, "电池包额定能量":dbl, "电池包额定总电压":dbl, "电池包累计充电总安时 3":dbl, "电池充满次数":dbl, "电池放空次数 3":dbl, "电池充电次数":dbl, "电池生产日期":string, "电池厂商":string, "电池类型 3":string, "电池包组号 3":string, "电池包产权标识 3":string, "电池应用车型":string}
  T3 = enum32{"单选选项2 5", "单选选项2 6", "单选选项2 7", "单选选项2 8"}
  T4 = cluster{"1 102":cluster{"第1串":dbl, "第2串":dbl, "第3串":dbl, "第4串":dbl, "第5串":dbl, "第6串":dbl, "第7串":dbl, "第8串":dbl, "第9串":dbl, "第10串":dbl, "第11串":dbl, "第12串":dbl, "第一串 2":dbl, "第一串 4":dbl, "第一串 6":dbl, "第一串 8":dbl, "第一串 10":dbl, "第一串 12":dbl, "第一串 14":dbl, "第一串 16":dbl, "第一串 18":dbl, "第一串 20":dbl, "第一串 22":dbl, "第一串 24":dbl}, "1 3":cluster{"第13串":dbl, "第14串":dbl, "第15串":dbl, "第16串":dbl, "第17串":dbl, "第18串":dbl, "第19串":dbl, "第20串":dbl, "第21串":dbl, "第22串":dbl, "第23串":dbl, "第24串":dbl, "第一串 2":dbl, "第一串 4":dbl, "第一串 6":dbl, "第一串 8":dbl, "第一串 10":dbl, "第一串 12":dbl, "第一串 14":dbl, "第一串 16":dbl, "第一串 18":dbl, "第一串 20":dbl, "第一串 22":dbl, "第一串 24":dbl}, "1 4":cluster{"第25串":dbl, "第26串":dbl, "第27串":dbl, "第28串":dbl, "第29串":dbl, "第30串":dbl, "第31串":dbl, "第32串":dbl, "第33串":dbl, "第34串":dbl, "第35串":dbl, "第36串":dbl, "第一串 2":dbl, "第一串 4":dbl, "第一串 6":dbl, "第一串 8":dbl, "第一串 10":dbl, "第一串 12":dbl, "第一串 14":dbl, "第一串 16":dbl, "第一串 18":dbl, "第一串 20":dbl, "第一串 22":dbl, "第一串 24":dbl}, "1 6":cluster{"第37串":dbl, "第38串":dbl, "第39串":dbl, "第40串":dbl, "第41串":dbl, "第42串":dbl, "第43串":dbl, "第44串":dbl, "第45串":dbl, "第46串":dbl, "第47串":dbl, "第48串":dbl, "第一串 2":dbl, "第一串 4":dbl, "第一串 6":dbl, "第一串 8":dbl, "第一串 10":dbl, "第一串 12":dbl, "第一串 14":dbl, "第一串 16":dbl, "第一串 18":dbl, "第一串 20":dbl, "第一串 22":dbl, "第一串 24":dbl}, "1 7":cluster{"第49串":dbl, "第50串":dbl, "第51串":dbl, "第52串":dbl, "第53串":dbl, "第54串":dbl, "第55串":dbl, "第56串":dbl, "第57串":dbl, "第58串":dbl, "第59串":dbl, "第60串":dbl, "第一串 2":dbl, "第一串 4":dbl, "第一串 6":dbl, "第一串 8":dbl, "第一串 10":dbl, "第一串 12":dbl, "第一串 14":dbl, "第一串 16":dbl, "第一串 18":dbl, "第一串 20":dbl, "第一串 22":dbl, "第一串 24":dbl}, "1 8":cluster{"第61串":dbl, "第62串":dbl, "第63串":dbl, "第64串":dbl, "第65串":dbl, "第66串":dbl, "第67串":dbl, "第68串":dbl, "第69串":dbl, "第70串":dbl, "第71串":dbl, "第72串":dbl, "第一串 2":dbl, "第一串 4":dbl, "第一串 6":dbl, "第一串 8":dbl, "第一串 10":dbl, "第一串 12":dbl, "第一串 14":dbl, "第一串 16":dbl, "第一串 18":dbl, "第一串 20":dbl, "第一串 22":dbl, "第一串 24":dbl}, "1 9":cluster{"第73串":dbl, "第74串":dbl, "第75串":dbl, "第76串":dbl, "第77串":dbl, "第78串":dbl, "第79串":dbl, "第80串":dbl, "第81串":dbl, "第82串":dbl, "第83串":dbl, "第84串":dbl, "第一串 2":dbl, "第一串 4":dbl, "第一串 6":dbl, "第一串 8":dbl, "第一串 10":dbl, "第一串 12":dbl, "第一串 14":dbl, "第一串 16":dbl, "第一串 18":dbl, "第一串 20":dbl, "第一串 22":dbl, "第一串 24":dbl}, "1 10":cluster{"第85串":dbl, "第86串":dbl, "第87串":dbl, "第88串":dbl, "第89串":dbl, "第90串":dbl, "第91串":dbl, "第92串":dbl, "第93串":dbl, "第94串":dbl, "第95串":dbl, "第96串":dbl, "第一串 2":dbl, "第一串 4":dbl, "第一串 6":dbl, "第一串 8":dbl, "第一串 10":dbl, "第一串 12":dbl, "第一串 14":dbl, "第一串 16":dbl, "第一串 18":dbl, "第一串 20":dbl, "第一串 22":dbl, "第一串 24":dbl}, "1 12":cluster{"充电1":u32, "充电1":u32, "充电1":u32, "充电1":u32, "充电1":u32, "充电1":u32, "充电1":u32, "充电1":u32, "充电1":u32, "充电1":u32, "充电1":u32, "充电1":u32}, "1 28":cluster{"充电1":u32, "充电1":u32, "充电1":u32, "充电1":u32, "充电1":u32, "充电1":u32, "充电1":u32, "充电1":u32, "充电1":u32, "充电1":u32, "充电1":u32, "充电1":u32}, "1 25":cluster{"充电1":u32, "充电1":u32, "充电1":u32, "充电1":u32, "充电1":u32, "充电1":u32, "充电1":u32, "充电1":u32, "充电1":u32, "充电1":u32, "充电1":u32, "充电1":u32}, "1 31":cluster{"充电1":u32, "充电1":u32, "充电1":u32, "充电1":u32, "充电1":u32, "充电1":u32, "充电1":u32, "充电1":u32, "充电1":u32, "充电1":u32, "充电1":u32, "充电1":u32}, "1 16":cluster{"充电1":u32, "充电1":u32, "充电1":u32, "充电1":u32, "充电1":u32, "充电1":u32, "充电1":u32, "充电1":u32, "充电1":u32, "充电1":u32, "充电1":u32, "充电1":u32}, "1 19":cluster{"充电1":u32, "充电1":u32, "充电1":u32, "充电1":u32, "充电1":u32, "充电1":u32, "充电1":u32, "充电1":u32, "充电1":u32, "充电1":u32, "充电1":u32, "充电1":u32}, "1 22":cluster{"充电1":u32, "充电1":u32, "充电1":u32, "充电1":u32, "充电1":u32, "充电1":u32, "充电1":u32, "充电1":u32, "充电1":u32, "充电1":u32, "充电1":u32, "充电1":u32}, "1 34":cluster{"充电1":u32, "充电1":u32, "充电1":u32, "充电1":u32, "充电1":u32, "充电1":u32, "充电1":u32, "充电1":u32, "充电1":u32, "充电1":u32, "充电1":u32, "充电1":u32}, "1 11":cluster{"充电1":u32, "充电1":u32, "充电1":u32, "充电1":u32, "充电1":u32, "充电1":u32, "充电1":u32, "充电1":u32, "充电1":u32, "充电1":u32, "充电1":u32, "充电1":u32}, "1 27":cluster{"充电1":u32, "充电1":u32, "充电1":u32, "充电1":u32, "充电1":u32, "充电1":u32, "充电1":u32, "充电1":u32, "充电1":u32, "充电1":u32, "充电1":u32, "充电1":u32}, "1 24":cluster{"充电1":u32, "充电1":u32, "充电1":u32, "充电1":u32, "充电1":u32, "充电1":u32, "充电1":u32, "充电1":u32, "充电1":u32, "充电1":u32, "充电1":u32, "充电1":u32}, "1 30":cluster{"充电1":u32, "充电1":u32, "充电1":u32, "充电1":u32, "充电1":u32, "充电1":u32, "充电1":u32, "充电1":u32, "充电1":u32, "充电1":u32, "充电1":u32, "充电1":u32}, "1 15":cluster{"充电1":u32, "充电1":u32, "充电1":u32, "充电1":u32, "充电1":u32, "充电1":u32, "充电1":u32, "充电1":u32, "充电1":u32, "充电1":u32, "充电1":u32, "充电1":u32}, "1 18":cluster{"充电1":u32, "充电1":u32, "充电1":u32, "充电1":u32, "充电1":u32, "充电1":u32, "充电1":u32, "充电1":u32, "充电1":u32, "充电1":u32, "充电1":u32, "充电1":u32}, "1 21":cluster{"充电1":u32, "充电1":u32, "充电1":u32, "充电1":u32, "充电1":u32, "充电1":u32, "充电1":u32, "充电1":u32, "充电1":u32, "充电1":u32, "充电1":u32, "充电1":u32}, "1 33":cluster{"充电1":u32, "充电1":u32, "充电1":u32, "充电1":u32, "充电1":u32, "充电1":u32, "充电1":u32, "充电1":u32, "充电1":u32, "充电1":u32, "充电1":u32, "充电1":u32}, "1 13":cluster{"均衡故障":i32, "均衡故障 2":dbl, "均衡故障 3":dbl, "均衡故障 4":dbl, "均衡故障 5":dbl, "均衡故障 6":dbl, "均衡故障 7":dbl, "均衡故障 8":dbl, "均衡故障 9":dbl, "均衡故障 10":dbl, "均衡故障 11":dbl, "均衡故障 12":dbl}, "1 26":cluster{"均衡故障":i32, "均衡故障 2":dbl, "均衡故障 3":dbl, "均衡故障 4":dbl, "均衡故障 5":dbl, "均衡故障 6":dbl, "均衡故障 7":dbl, "均衡故障 8":dbl, "均衡故障 9":dbl, "均衡故障 10":dbl, "均衡故障 11":dbl, "均衡故障 12":dbl}, "1 23":cluster{"均衡故障":i32, "均衡故障 2":dbl, "均衡故障 3":dbl, "均衡故障 4":dbl, "均衡故障 5":dbl, "均衡故障 6":dbl, "均衡故障 7":dbl, "均衡故障 8":dbl, "均衡故障 9":dbl, "均衡故障 10":dbl, "均衡故障 11":dbl, "均衡故障 12":dbl}, "1 29":cluster{"均衡故障":i32, "均衡故障 2":dbl, "均衡故障 3":dbl, "均衡故障 4":dbl, "均衡故障 5":dbl, "均衡故障 6":dbl, "均衡故障 7":dbl, "均衡故障 8":dbl, "均衡故障 9":dbl, "均衡故障 10":dbl, "均衡故障 11":dbl, "均衡故障 12":dbl}, "1 14":cluster{"均衡故障":i32, "均衡故障 2":dbl, "均衡故障 3":dbl, "均衡故障 4":dbl, "均衡故障 5":dbl, "均衡故障 6":dbl, "均衡故障 7":dbl, "均衡故障 8":dbl, "均衡故障 9":dbl, "均衡故障 10":dbl, "均衡故障 11":dbl, "均衡故障 12":dbl}, "1 17":cluster{"均衡故障":i32, "均衡故障 2":dbl, "均衡故障 3":dbl, "均衡故障 4":dbl, "均衡故障 5":dbl, "均衡故障 6":dbl, "均衡故障 7":dbl, "均衡故障 8":dbl, "均衡故障 9":dbl, "均衡故障 10":dbl, "均衡故障 11":dbl, "均衡故障 12":dbl}, "1 20":cluster{"均衡故障":i32, "均衡故障 2":dbl, "均衡故障 3":dbl, "均衡故障 4":dbl, "均衡故障 5":dbl, "均衡故障 6":dbl, "均衡故障 7":dbl, "均衡故障 8":dbl, "均衡故障 9":dbl, "均衡故障 10":dbl, "均衡故障 11":dbl, "均衡故障 12":dbl}, "1 32":cluster{"均衡故障":i32, "均衡故障 2":dbl, "均衡故障 3":dbl, "均衡故障 4":dbl, "均衡故障 5":dbl, "均衡故障 6":dbl, "均衡故障 7":dbl, "均衡故障 8":dbl, "均衡故障 9":dbl, "均衡故障 10":dbl, "均衡故障 11":dbl, "均衡故障 12":dbl}}
  T5 = cluster{"1 26":cluster{"第97串":dbl, "第98串":dbl, "第99串":dbl, "第100串":dbl, "第101串":dbl, "第102串":dbl, "第103串":dbl, "第104串":dbl, "第105串":dbl, "第106串":dbl, "第107串":dbl, "第108串":dbl, "第一串 2":dbl, "第一串 4":dbl, "第一串 6":dbl, "第一串 8":dbl, "第一串 10":dbl, "第一串 12":dbl, "第一串 14":dbl, "第一串 16":dbl, "第一串 18":dbl, "第一串 20":dbl, "第一串 22":dbl, "第一串 24":dbl}, "1 27":cluster{"第109串":dbl, "第110串":dbl, "第111串":dbl, "第112串":dbl, "第113串":dbl, "第114串":dbl, "第115串":dbl, "第116串":dbl, "第117串":dbl, "第118串":dbl, "第119串":dbl, "第120串":dbl, "第一串 2":dbl, "第一串 4":dbl, "第一串 6":dbl, "第一串 8":dbl, "第一串 10":dbl, "第一串 12":dbl, "第一串 14":dbl, "第一串 16":dbl, "第一串 18":dbl, "第一串 20":dbl, "第一串 22":dbl, "第一串 24":dbl}, "1 28":cluster{"第121串":dbl, "第122串":dbl, "第123串":dbl, "第124串":dbl, "第125串":dbl, "第126串":dbl, "第127串":dbl, "第128串":dbl, "第129串":dbl, "第130串":dbl, "第131串":dbl, "第132串":dbl, "第一串 2":dbl, "第一串 4":dbl, "第一串 6":dbl, "第一串 8":dbl, "第一串 10":dbl, "第一串 12":dbl, "第一串 14":dbl, "第一串 16":dbl, "第一串 18":dbl, "第一串 20":dbl, "第一串 22":dbl, "第一串 24":dbl}, "1 29":cluster{"第133串":dbl, "第134串":dbl, "第135串":dbl, "第136串":dbl, "第137串":dbl, "第138串":dbl, "第139串":dbl, "第140串":dbl, "第141串":dbl, "第142串":dbl, "第143串":dbl, "第144串":dbl, "第一串 2":dbl, "第一串 4":dbl, "第一串 6":dbl, "第一串 8":dbl, "第一串 10":dbl, "第一串 12":dbl, "第一串 14":dbl, "第一串 16":dbl, "第一串 18":dbl, "第一串 20":dbl, "第一串 22":dbl, "第一串 24":dbl}, "1 30":cluster{"第145串":dbl, "第146串":dbl, "第147串":dbl, "第148串":dbl, "第149串":dbl, "第150串":dbl, "第151串":dbl, "第152串":dbl, "第153串":dbl, "第154串":dbl, "第155串":dbl, "第156串":dbl, "第一串 2":dbl, "第一串 4":dbl, "第一串 6":dbl, "第一串 8":dbl, "第一串 10":dbl, "第一串 12":dbl, "第一串 14":dbl, "第一串 16":dbl, "第一串 18":dbl, "第一串 20":dbl, "第一串 22":dbl, "第一串 24":dbl}, "1 31":cluster{"第157串":dbl, "第158串":dbl, "第159串":dbl, "第160串":dbl, "第161串":dbl, "第162串":dbl, "第163串":dbl, "第164串":dbl, "第165串":dbl, "第166串":dbl, "第167串":dbl, "第168串":dbl, "第一串 2":dbl, "第一串 4":dbl, "第一串 6":dbl, "第一串 8":dbl, "第一串 10":dbl, "第一串 12":dbl, "第一串 14":dbl, "第一串 16":dbl, "第一串 18":dbl, "第一串 20":dbl, "第一串 22":dbl, "第一串 24":dbl}, "1 32":cluster{"第169串":dbl, "第170串":dbl, "第171串":dbl, "第172串":dbl, "第173串":dbl, "第174串":dbl, "第175串":dbl, "第176串":dbl, "第177串":dbl, "第178串":dbl, "第179串":dbl, "第180串":dbl, "第一串 2":dbl, "第一串 4":dbl, "第一串 6":dbl, "第一串 8":dbl, "第一串 10":dbl, "第一串 12":dbl, "第一串 14":dbl, "第一串 16":dbl, "第一串 18":dbl, "第一串 20":dbl, "第一串 22":dbl, "第一串 24":dbl}, "1 33":cluster{"第181串":dbl, "第182串":dbl, "第183串":dbl, "第184串":dbl, "第185串":dbl, "第186串":dbl, "第187串":dbl, "第188串":dbl, "第189串":dbl, "第190串":dbl, "第191串":dbl, "第192串":dbl, "第一串 2":dbl, "第一串 4":dbl, "第一串 6":dbl, "第一串 8":dbl, "第一串 10":dbl, "第一串 12":dbl, "第一串 14":dbl, "第一串 16":dbl, "第一串 18":dbl, "第一串 20":dbl, "第一串 22":dbl, "第一串 24":dbl}, "1 16":cluster{"充电1":u32, "充电1":u32, "充电1":u32, "充电1":u32, "充电1":u32, "充电1":u32, "充电1":u32, "充电1":u32, "充电1":u32, "充电1":u32, "充电1":u32, "充电1":u32}, "1 44":cluster{"充电1":u32, "充电1":u32, "充电1":u32, "充电1":u32, "充电1":u32, "充电1":u32, "充电1":u32, "充电1":u32, "充电1":u32, "充电1":u32, "充电1":u32, "充电1":u32}, "1 36":cluster{"充电1":u32, "充电1":u32, "充电1":u32, "充电1":u32, "充电1":u32, "充电1":u32, "充电1":u32, "充电1":u32, "充电1":u32, "充电1":u32, "充电1":u32, "充电1":u32}, "1 47":cluster{"充电1":u32, "充电1":u32, "充电1":u32, "充电1":u32, "充电1":u32, "充电1":u32, "充电1":u32, "充电1":u32, "充电1":u32, "充电1":u32, "充电1":u32, "充电1":u32}, "1 19":cluster{"充电1":u32, "充电1":u32, "充电1":u32, "充电1":u32, "充电1":u32, "充电1":u32, "充电1":u32, "充电1":u32, "充电1":u32, "充电1":u32, "充电1":u32, "充电1":u32}, "1 38":cluster{"充电1":u32, "充电1":u32, "充电1":u32, "充电1":u32, "充电1":u32, "充电1":u32, "充电1":u32, "充电1":u32, "充电1":u32, "充电1":u32, "充电1":u32, "充电1":u32}, "1 41":cluster{"充电1":u32, "充电1":u32, "充电1":u32, "充电1":u32, "充电1":u32, "充电1":u32, "充电1":u32, "充电1":u32, "充电1":u32, "充电1":u32, "充电1":u32, "充电1":u32}, "1 50":cluster{"充电1":u32, "充电1":u32, "充电1":u32, "充电1":u32, "充电1":u32, "充电1":u32, "充电1":u32, "充电1":u32, "充电1":u32, "充电1":u32, "充电1":u32, "充电1":u32}, "1 15":cluster{"充电1":u32, "充电1":u32, "充电1":u32, "充电1":u32, "充电1":u32, "充电1":u32, "充电1":u32, "充电1":u32, "充电1":u32, "充电1":u32, "充电1":u32, "充电1":u32}, "1 43":cluster{"充电1":u32, "充电1":u32, "充电1":u32, "充电1":u32, "充电1":u32, "充电1":u32, "充电1":u32, "充电1":u32, "充电1":u32, "充电1":u32, "充电1":u32, "充电1":u32}, "1 35":cluster{"充电1":u32, "充电1":u32, "充电1":u32, "充电1":u32, "充电1":u32, "充电1":u32, "充电1":u32, "充电1":u32, "充电1":u32, "充电1":u32, "充电1":u32, "充电1":u32}, "1 46":cluster{"充电1":u32, "充电1":u32, "充电1":u32, "充电1":u32, "充电1":u32, "充电1":u32, "充电1":u32, "充电1":u32, "充电1":u32, "充电1":u32, "充电1":u32, "充电1":u32}, "1 18":cluster{"充电1":u32, "充电1":u32, "充电1":u32, "充电1":u32, "充电1":u32, "充电1":u32, "充电1":u32, "充电1":u32, "充电1":u32, "充电1":u32, "充电1":u32, "充电1":u32}, "1 37":cluster{"充电1":u32, "充电1":u32, "充电1":u32, "充电1":u32, "充电1":u32, "充电1":u32, "充电1":u32, "充电1":u32, "充电1":u32, "充电1":u32, "充电1":u32, "充电1":u32}, "1 40":cluster{"充电1":u32, "充电1":u32, "充电1":u32, "充电1":u32, "充电1":u32, "充电1":u32, "充电1":u32, "充电1":u32, "充电1":u32, "充电1":u32, "充电1":u32, "充电1":u32}, "1 49":cluster{"充电1":u32, "充电1":u32, "充电1":u32, "充电1":u32, "充电1":u32, "充电1":u32, "充电1":u32, "充电1":u32, "充电1":u32, "充电1":u32, "充电1":u32, "充电1":u32}, "1 14":cluster{"均衡故障":i32, "均衡故障 2":dbl, "均衡故障 3":dbl, "均衡故障 4":dbl, "均衡故障 5":dbl, "均衡故障 6":dbl, "均衡故障 7":dbl, "均衡故障 8":dbl, "均衡故障 9":dbl, "均衡故障 10":dbl, "均衡故障 11":dbl, "均衡故障 12":dbl}, "1 42":cluster{"均衡故障":i32, "均衡故障 2":dbl, "均衡故障 3":dbl, "均衡故障 4":dbl, "均衡故障 5":dbl, "均衡故障 6":dbl, "均衡故障 7":dbl, "均衡故障 8":dbl, "均衡故障 9":dbl, "均衡故障 10":dbl, "均衡故障 11":dbl, "均衡故障 12":dbl}, "1 34":cluster{"均衡故障":i32, "均衡故障 2":dbl, "均衡故障 3":dbl, "均衡故障 4":dbl, "均衡故障 5":dbl, "均衡故障 6":dbl, "均衡故障 7":dbl, "均衡故障 8":dbl, "均衡故障 9":dbl, "均衡故障 10":dbl, "均衡故障 11":dbl, "均衡故障 12":dbl}, "1 45":cluster{"均衡故障":i32, "均衡故障 2":dbl, "均衡故障 3":dbl, "均衡故障 4":dbl, "均衡故障 5":dbl, "均衡故障 6":dbl, "均衡故障 7":dbl, "均衡故障 8":dbl, "均衡故障 9":dbl, "均衡故障 10":dbl, "均衡故障 11":dbl, "均衡故障 12":dbl}, "1 17":cluster{"均衡故障":i32, "均衡故障 2":dbl, "均衡故障 3":dbl, "均衡故障 4":dbl, "均衡故障 5":dbl, "均衡故障 6":dbl, "均衡故障 7":dbl, "均衡故障 8":dbl, "均衡故障 9":dbl, "均衡故障 10":dbl, "均衡故障 11":dbl, "均衡故障 12":dbl}, "1 20":cluster{"均衡故障":i32, "均衡故障 2":dbl, "均衡故障 3":dbl, "均衡故障 4":dbl, "均衡故障 5":dbl, "均衡故障 6":dbl, "均衡故障 7":dbl, "均衡故障 8":dbl, "均衡故障 9":dbl, "均衡故障 10":dbl, "均衡故障 11":dbl, "均衡故障 12":dbl}, "1 39":cluster{"均衡故障":i32, "均衡故障 2":dbl, "均衡故障 3":dbl, "均衡故障 4":dbl, "均衡故障 5":dbl, "均衡故障 6":dbl, "均衡故障 7":dbl, "均衡故障 8":dbl, "均衡故障 9":dbl, "均衡故障 10":dbl, "均衡故障 11":dbl, "均衡故障 12":dbl}, "1 48":cluster{"均衡故障":i32, "均衡故障 2":dbl, "均衡故障 3":dbl, "均衡故障 4":dbl, "均衡故障 5":dbl, "均衡故障 6":dbl, "均衡故障 7":dbl, "均衡故障 8":dbl, "均衡故障 9":dbl, "均衡故障 10":dbl, "均衡故障 11":dbl, "均衡故障 12":dbl}}
  T6 = cluster{"1 18":cluster{"第193串":dbl, "第194串":dbl, "第195串":dbl, "第196串":dbl, "第197串":dbl, "第198串":dbl, "第199串":dbl, "第200串":dbl, "第201串":dbl, "第202串":dbl, "第203串":dbl, "第204串":dbl, "第一串 2":dbl, "第一串 4":dbl, "第一串 6":dbl, "第一串 8":dbl, "第一串 10":dbl, "第一串 12":dbl, "第一串 14":dbl, "第一串 16":dbl, "第一串 18":dbl, "第一串 20":dbl, "第一串 22":dbl, "第一串 24":dbl}, "1 19":cluster{"第205串":dbl, "第206串":dbl, "第207串":dbl, "第208串":dbl, "第209串":dbl, "第210串":dbl, "第211串":dbl, "第212串":dbl, "第213串":dbl, "第214串":dbl, "第215串":dbl, "第216串":dbl, "第一串 2":dbl, "第一串 4":dbl, "第一串 6":dbl, "第一串 8":dbl, "第一串 10":dbl, "第一串 12":dbl, "第一串 14":dbl, "第一串 16":dbl, "第一串 18":dbl, "第一串 20":dbl, "第一串 22":dbl, "第一串 24":dbl}, "1 20":cluster{"第217串":dbl, "第218串":dbl, "第219串":dbl, "第220串":dbl, "第221串":dbl, "第222串":dbl, "第223串":dbl, "第224串":dbl, "第225串":dbl, "第226串":dbl, "第227串":dbl, "第228串":dbl, "第一串 2":dbl, "第一串 4":dbl, "第一串 6":dbl, "第一串 8":dbl, "第一串 10":dbl, "第一串 12":dbl, "第一串 14":dbl, "第一串 16":dbl, "第一串 18":dbl, "第一串 20":dbl, "第一串 22":dbl, "第一串 24":dbl}, "1 21":cluster{"第229串":dbl, "第230串":dbl, "第231串":dbl, "第232串":dbl, "第233串":dbl, "第234串":dbl, "第235串":dbl, "第236串":dbl, "第237串":dbl, "第238串":dbl, "第239串":dbl, "第240串":dbl, "第一串 2":dbl, "第一串 4":dbl, "第一串 6":dbl, "第一串 8":dbl, "第一串 10":dbl, "第一串 12":dbl, "第一串 14":dbl, "第一串 16":dbl, "第一串 18":dbl, "第一串 20":dbl, "第一串 22":dbl, "第一串 24":dbl}, "1 22":cluster{"第241串":dbl, "第242串":dbl, "第243串":dbl, "第244串":dbl, "第245串":dbl, "第246串":dbl, "第247串":dbl, "第248串":dbl, "第249串":dbl, "第250串":dbl, "第251串":dbl, "第252串":dbl, "第一串 2":dbl, "第一串 4":dbl, "第一串 6":dbl, "第一串 8":dbl, "第一串 10":dbl, "第一串 12":dbl, "第一串 14":dbl, "第一串 16":dbl, "第一串 18":dbl, "第一串 20":dbl, "第一串 22":dbl, "第一串 24":dbl}, "1 23":cluster{"第253串":dbl, "第254串":dbl, "第255串":dbl, "第256串":dbl, "第257串":dbl, "第258串":dbl, "第259串":dbl, "第260串":dbl, "第261串":dbl, "第262串":dbl, "第263串":dbl, "第264串":dbl, "第一串 2":dbl, "第一串 4":dbl, "第一串 6":dbl, "第一串 8":dbl, "第一串 10":dbl, "第一串 12":dbl, "第一串 14":dbl, "第一串 16":dbl, "第一串 18":dbl, "第一串 20":dbl, "第一串 22":dbl, "第一串 24":dbl}, "1 24":cluster{"第265串":dbl, "第266串":dbl, "第267串":dbl, "第268串":dbl, "第269串":dbl, "第270串":dbl, "第271串":dbl, "第272串":dbl, "第273串":dbl, "第274串":dbl, "第275串":dbl, "第276串":dbl, "第一串 2":dbl, "第一串 4":dbl, "第一串 6":dbl, "第一串 8":dbl, "第一串 10":dbl, "第一串 12":dbl, "第一串 14":dbl, "第一串 16":dbl, "第一串 18":dbl, "第一串 20":dbl, "第一串 22":dbl, "第一串 24":dbl}, "1 25":cluster{"第277串":dbl, "第278串":dbl, "第279串":dbl, "第280串":dbl, "第281串":dbl, "第282串":dbl, "第283串":dbl, "第284串":dbl, "第285串":dbl, "第286串":dbl, "第287串":dbl, "第288串":dbl, "第一串 2":dbl, "第一串 4":dbl, "第一串 6":dbl, "第一串 8":dbl, "第一串 10":dbl, "第一串 12":dbl, "第一串 14":dbl, "第一串 16":dbl, "第一串 18":dbl, "第一串 20":dbl, "第一串 22":dbl, "第一串 24":dbl}, "1 12":cluster{"充电1":u32, "充电1":u32, "充电1":u32, "充电1":u32, "充电1":u32, "充电1":u32, "充电1":u32, "充电1":u32, "充电1":u32, "充电1":u32, "充电1":u32, "充电1":u32}, "1 39":cluster{"充电1":u32, "充电1":u32, "充电1":u32, "充电1":u32, "充电1":u32, "充电1":u32, "充电1":u32, "充电1":u32, "充电1":u32, "充电1":u32, "充电1":u32, "充电1":u32}, "1 28":cluster{"充电1":u32, "充电1":u32, "充电1":u32, "充电1":u32, "充电1":u32, "充电1":u32, "充电1":u32, "充电1":u32, "充电1":u32, "充电1":u32, "充电1":u32, "充电1":u32}, "1 42":cluster{"充电1":u32, "充电1":u32, "充电1":u32, "充电1":u32, "充电1":u32, "充电1":u32, "充电1":u32, "充电1":u32, "充电1":u32, "充电1":u32, "充电1":u32, "充电1":u32}, "1 16":cluster{"充电1":u32, "充电1":u32, "充电1":u32, "充电1":u32, "充电1":u32, "充电1":u32, "充电1":u32, "充电1":u32, "充电1":u32, "充电1":u32, "充电1":u32, "充电1":u32}, "1 30":cluster{"充电1":u32, "充电1":u32, "充电1":u32, "充电1":u32, "充电1":u32, "充电1":u32, "充电1":u32, "充电1":u32, "充电1":u32, "充电1":u32, "充电1":u32, "充电1":u32}, "1 33":cluster{"充电1":u32, "充电1":u32, "充电1":u32, "充电1":u32, "充电1":u32, "充电1":u32, "充电1":u32, "充电1":u32, "充电1":u32, "充电1":u32, "充电1":u32, "充电1":u32}, "1 36":cluster{"充电1":u32, "充电1":u32, "充电1":u32, "充电1":u32, "充电1":u32, "充电1":u32, "充电1":u32, "充电1":u32, "充电1":u32, "充电1":u32, "充电1":u32, "充电1":u32}, "1 11":cluster{"充电1":u32, "充电1":u32, "充电1":u32, "充电1":u32, "充电1":u32, "充电1":u32, "充电1":u32, "充电1":u32, "充电1":u32, "充电1":u32, "充电1":u32, "充电1":u32}, "1 38":cluster{"充电1":u32, "充电1":u32, "充电1":u32, "充电1":u32, "充电1":u32, "充电1":u32, "充电1":u32, "充电1":u32, "充电1":u32, "充电1":u32, "充电1":u32, "充电1":u32}, "1 27":cluster{"充电1":u32, "充电1":u32, "充电1":u32, "充电1":u32, "充电1":u32, "充电1":u32, "充电1":u32, "充电1":u32, "充电1":u32, "充电1":u32, "充电1":u32, "充电1":u32}, "1 41":cluster{"充电1":u32, "充电1":u32, "充电1":u32, "充电1":u32, "充电1":u32, "充电1":u32, "充电1":u32, "充电1":u32, "充电1":u32, "充电1":u32, "充电1":u32, "充电1":u32}, "1 15":cluster{"充电1":u32, "充电1":u32, "充电1":u32, "充电1":u32, "充电1":u32, "充电1":u32, "充电1":u32, "充电1":u32, "充电1":u32, "充电1":u32, "充电1":u32, "充电1":u32}, "1 29":cluster{"充电1":u32, "充电1":u32, "充电1":u32, "充电1":u32, "充电1":u32, "充电1":u32, "充电1":u32, "充电1":u32, "充电1":u32, "充电1":u32, "充电1":u32, "充电1":u32}, "1 32":cluster{"充电1":u32, "充电1":u32, "充电1":u32, "充电1":u32, "充电1":u32, "充电1":u32, "充电1":u32, "充电1":u32, "充电1":u32, "充电1":u32, "充电1":u32, "充电1":u32}, "1 35":cluster{"充电1":u32, "充电1":u32, "充电1":u32, "充电1":u32, "充电1":u32, "充电1":u32, "充电1":u32, "充电1":u32, "充电1":u32, "充电1":u32, "充电1":u32, "充电1":u32}, "1 13":cluster{"均衡故障":i32, "均衡故障 2":dbl, "均衡故障 3":dbl, "均衡故障 4":dbl, "均衡故障 5":dbl, "均衡故障 6":dbl, "均衡故障 7":dbl, "均衡故障 8":dbl, "均衡故障 9":dbl, "均衡故障 10":dbl, "均衡故障 11":dbl, "均衡故障 12":dbl}, "1 37":cluster{"均衡故障":i32, "均衡故障 2":dbl, "均衡故障 3":dbl, "均衡故障 4":dbl, "均衡故障 5":dbl, "均衡故障 6":dbl, "均衡故障 7":dbl, "均衡故障 8":dbl, "均衡故障 9":dbl, "均衡故障 10":dbl, "均衡故障 11":dbl, "均衡故障 12":dbl}, "1 26":cluster{"均衡故障":i32, "均衡故障 2":dbl, "均衡故障 3":dbl, "均衡故障 4":dbl, "均衡故障 5":dbl, "均衡故障 6":dbl, "均衡故障 7":dbl, "均衡故障 8":dbl, "均衡故障 9":dbl, "均衡故障 10":dbl, "均衡故障 11":dbl, "均衡故障 12":dbl}, "1 40":cluster{"均衡故障":i32, "均衡故障 2":dbl, "均衡故障 3":dbl, "均衡故障 4":dbl, "均衡故障 5":dbl, "均衡故障 6":dbl, "均衡故障 7":dbl, "均衡故障 8":dbl, "均衡故障 9":dbl, "均衡故障 10":dbl, "均衡故障 11":dbl, "均衡故障 12":dbl}, "1 14":cluster{"均衡故障":i32, "均衡故障 2":dbl, "均衡故障 3":dbl, "均衡故障 4":dbl, "均衡故障 5":dbl, "均衡故障 6":dbl, "均衡故障 7":dbl, "均衡故障 8":dbl, "均衡故障 9":dbl, "均衡故障 10":dbl, "均衡故障 11":dbl, "均衡故障 12":dbl}, "1 17":cluster{"均衡故障":i32, "均衡故障 2":dbl, "均衡故障 3":dbl, "均衡故障 4":dbl, "均衡故障 5":dbl, "均衡故障 6":dbl, "均衡故障 7":dbl, "均衡故障 8":dbl, "均衡故障 9":dbl, "均衡故障 10":dbl, "均衡故障 11":dbl, "均衡故障 12":dbl}, "1 31":cluster{"均衡故障":i32, "均衡故障 2":dbl, "均衡故障 3":dbl, "均衡故障 4":dbl, "均衡故障 5":dbl, "均衡故障 6":dbl, "均衡故障 7":dbl, "均衡故障 8":dbl, "均衡故障 9":dbl, "均衡故障 10":dbl, "均衡故障 11":dbl, "均衡故障 12":dbl}, "1 34":cluster{"均衡故障":i32, "均衡故障 2":dbl, "均衡故障 3":dbl, "均衡故障 4":dbl, "均衡故障 5":dbl, "均衡故障 6":dbl, "均衡故障 7":dbl, "均衡故障 8":dbl, "均衡故障 9":dbl, "均衡故障 10":dbl, "均衡故障 11":dbl, "均衡故障 12":dbl}}
  T7 = cluster{"第289串":dbl, "第290串":dbl, "第291串":dbl, "第292串":dbl, "第293串":dbl, "第294串":dbl, "第295串":dbl, "第296串":dbl, "第297串":dbl, "第298串":dbl, "第299串":dbl, "第300串":dbl, "第一串 2":dbl, "第一串 4":dbl, "第一串 6":dbl, "第一串 8":dbl, "第一串 10":dbl, "第一串 12":dbl, "第一串 14":dbl, "第一串 16":dbl, "第一串 18":dbl, "第一串 20":dbl, "第一串 22":dbl, "第一串 24":dbl}
  T8 = cluster{"均衡故障":i32, "均衡故障 2":dbl, "均衡故障 3":dbl, "均衡故障 4":dbl, "均衡故障 5":dbl, "均衡故障 6":dbl, "均衡故障 7":dbl, "均衡故障 8":dbl, "均衡故障 9":dbl, "均衡故障 10":dbl, "均衡故障 11":dbl, "均衡故障 12":dbl}
  T9 = cluster{"充电1":u32, "充电1":u32, "充电1":u32, "充电1":u32, "充电1":u32, "充电1":u32, "充电1":u32, "充电1":u32, "充电1":u32, "充电1":u32, "充电1":u32, "充电1":u32}
  T10 = cluster{"1 102":cluster{"第1串":dbl, "第2串":dbl, "第3串":dbl, "第4串":dbl, "第5串":dbl, "第6串":dbl, "第7串":dbl, "第8串":dbl, "第9串":dbl, "第10串":dbl, "第11串":dbl, "第12串":dbl, "第一串 2":dbl, "第一串 4":dbl, "第一串 6":dbl, "第一串 8":dbl, "第一串 10":dbl, "第一串 12":dbl, "第一串 14":dbl, "第一串 16":dbl, "第一串 18":dbl, "第一串 20":dbl, "第一串 22":dbl, "第一串 24":dbl}, "1 3":cluster{"第13串":dbl, "第14串":dbl, "第15串":dbl, "第16串":dbl, "第17串":dbl, "第18串":dbl, "第19串":dbl, "第20串":dbl, "第21串":dbl, "第22串":dbl, "第23串":dbl, "第24串":dbl, "第一串 2":dbl, "第一串 4":dbl, "第一串 6":dbl, "第一串 8":dbl, "第一串 10":dbl, "第一串 12":dbl, "第一串 14":dbl, "第一串 16":dbl, "第一串 18":dbl, "第一串 20":dbl, "第一串 22":dbl, "第一串 24":dbl}, "1 4":cluster{"第25串":dbl, "第26串":dbl, "第27串":dbl, "第28串":dbl, "第29串":dbl, "第30串":dbl, "第31串":dbl, "第32串":dbl, "第33串":dbl, "第34串":dbl, "第35串":dbl, "第36串":dbl, "第一串 2":dbl, "第一串 4":dbl, "第一串 6":dbl, "第一串 8":dbl, "第一串 10":dbl, "第一串 12":dbl, "第一串 14":dbl, "第一串 16":dbl, "第一串 18":dbl, "第一串 20":dbl, "第一串 22":dbl, "第一串 24":dbl}, "1 6":cluster{"第37串":dbl, "第38串":dbl, "第39串":dbl, "第40串":dbl, "第41串":dbl, "第42串":dbl, "第43串":dbl, "第44串":dbl, "第45串":dbl, "第46串":dbl, "第47串":dbl, "第48串":dbl, "第一串 2":dbl, "第一串 4":dbl, "第一串 6":dbl, "第一串 8":dbl, "第一串 10":dbl, "第一串 12":dbl, "第一串 14":dbl, "第一串 16":dbl, "第一串 18":dbl, "第一串 20":dbl, "第一串 22":dbl, "第一串 24":dbl}, "1 7":cluster{"第49串":dbl, "第50串":dbl, "第51串":dbl, "第52串":dbl, "第53串":dbl, "第54串":dbl, "第55串":dbl, "第56串":dbl, "第57串":dbl, "第58串":dbl, "第59串":dbl, "第60串":dbl, "第一串 2":dbl, "第一串 4":dbl, "第一串 6":dbl, "第一串 8":dbl, "第一串 10":dbl, "第一串 12":dbl, "第一串 14":dbl, "第一串 16":dbl, "第一串 18":dbl, "第一串 20":dbl, "第一串 22":dbl, "第一串 24":dbl}, "1 8":cluster{"第61串":dbl, "第62串":dbl, "第63串":dbl, "第64串":dbl, "第65串":dbl, "第66串":dbl, "第67串":dbl, "第68串":dbl, "第69串":dbl, "第70串":dbl, "第71串":dbl, "第72串":dbl, "第一串 2":dbl, "第一串 4":dbl, "第一串 6":dbl, "第一串 8":dbl, "第一串 10":dbl, "第一串 12":dbl, "第一串 14":dbl, "第一串 16":dbl, "第一串 18":dbl, "第一串 20":dbl, "第一串 22":dbl, "第一串 24":dbl}, "1 9":cluster{"第73串":dbl, "第74串":dbl, "第75串":dbl, "第76串":dbl, "第77串":dbl, "第78串":dbl, "第79串":dbl, "第80串":dbl, "第81串":dbl, "第82串":dbl, "第83串":dbl, "第84串":dbl, "第一串 2":dbl, "第一串 4":dbl, "第一串 6":dbl, "第一串 8":dbl, "第一串 10":dbl, "第一串 12":dbl, "第一串 14":dbl, "第一串 16":dbl, "第一串 18":dbl, "第一串 20":dbl, "第一串 22":dbl, "第一串 24":dbl}, "1 10":cluster{"第85串":dbl, "第86串":dbl, "第87串":dbl, "第88串":dbl, "第89串":dbl, "第90串":dbl, "第91串":dbl, "第92串":dbl, "第93串":dbl, "第94串":dbl, "第95串":dbl, "第96串":dbl, "第一串 2":dbl, "第一串 4":dbl, "第一串 6":dbl, "第一串 8":dbl, "第一串 10":dbl, "第一串 12":dbl, "第一串 14":dbl, "第一串 16":dbl, "第一串 18":dbl, "第一串 20":dbl, "第一串 22":dbl, "第一串 24":dbl}}
  T11 = cluster{"1 26":cluster{"第97串":dbl, "第98串":dbl, "第99串":dbl, "第100串":dbl, "第101串":dbl, "第102串":dbl, "第103串":dbl, "第104串":dbl, "第105串":dbl, "第106串":dbl, "第107串":dbl, "第108串":dbl, "第一串 2":dbl, "第一串 4":dbl, "第一串 6":dbl, "第一串 8":dbl, "第一串 10":dbl, "第一串 12":dbl, "第一串 14":dbl, "第一串 16":dbl, "第一串 18":dbl, "第一串 20":dbl, "第一串 22":dbl, "第一串 24":dbl}, "1 27":cluster{"第109串":dbl, "第110串":dbl, "第111串":dbl, "第112串":dbl, "第113串":dbl, "第114串":dbl, "第115串":dbl, "第116串":dbl, "第117串":dbl, "第118串":dbl, "第119串":dbl, "第120串":dbl, "第一串 2":dbl, "第一串 4":dbl, "第一串 6":dbl, "第一串 8":dbl, "第一串 10":dbl, "第一串 12":dbl, "第一串 14":dbl, "第一串 16":dbl, "第一串 18":dbl, "第一串 20":dbl, "第一串 22":dbl, "第一串 24":dbl}, "1 28":cluster{"第121串":dbl, "第122串":dbl, "第123串":dbl, "第124串":dbl, "第125串":dbl, "第126串":dbl, "第127串":dbl, "第128串":dbl, "第129串":dbl, "第130串":dbl, "第131串":dbl, "第132串":dbl, "第一串 2":dbl, "第一串 4":dbl, "第一串 6":dbl, "第一串 8":dbl, "第一串 10":dbl, "第一串 12":dbl, "第一串 14":dbl, "第一串 16":dbl, "第一串 18":dbl, "第一串 20":dbl, "第一串 22":dbl, "第一串 24":dbl}, "1 29":cluster{"第133串":dbl, "第134串":dbl, "第135串":dbl, "第136串":dbl, "第137串":dbl, "第138串":dbl, "第139串":dbl, "第140串":dbl, "第141串":dbl, "第142串":dbl, "第143串":dbl, "第144串":dbl, "第一串 2":dbl, "第一串 4":dbl, "第一串 6":dbl, "第一串 8":dbl, "第一串 10":dbl, "第一串 12":dbl, "第一串 14":dbl, "第一串 16":dbl, "第一串 18":dbl, "第一串 20":dbl, "第一串 22":dbl, "第一串 24":dbl}, "1 30":cluster{"第145串":dbl, "第146串":dbl, "第147串":dbl, "第148串":dbl, "第149串":dbl, "第150串":dbl, "第151串":dbl, "第152串":dbl, "第153串":dbl, "第154串":dbl, "第155串":dbl, "第156串":dbl, "第一串 2":dbl, "第一串 4":dbl, "第一串 6":dbl, "第一串 8":dbl, "第一串 10":dbl, "第一串 12":dbl, "第一串 14":dbl, "第一串 16":dbl, "第一串 18":dbl, "第一串 20":dbl, "第一串 22":dbl, "第一串 24":dbl}, "1 31":cluster{"第157串":dbl, "第158串":dbl, "第159串":dbl, "第160串":dbl, "第161串":dbl, "第162串":dbl, "第163串":dbl, "第164串":dbl, "第165串":dbl, "第166串":dbl, "第167串":dbl, "第168串":dbl, "第一串 2":dbl, "第一串 4":dbl, "第一串 6":dbl, "第一串 8":dbl, "第一串 10":dbl, "第一串 12":dbl, "第一串 14":dbl, "第一串 16":dbl, "第一串 18":dbl, "第一串 20":dbl, "第一串 22":dbl, "第一串 24":dbl}, "1 32":cluster{"第169串":dbl, "第170串":dbl, "第171串":dbl, "第172串":dbl, "第173串":dbl, "第174串":dbl, "第175串":dbl, "第176串":dbl, "第177串":dbl, "第178串":dbl, "第179串":dbl, "第180串":dbl, "第一串 2":dbl, "第一串 4":dbl, "第一串 6":dbl, "第一串 8":dbl, "第一串 10":dbl, "第一串 12":dbl, "第一串 14":dbl, "第一串 16":dbl, "第一串 18":dbl, "第一串 20":dbl, "第一串 22":dbl, "第一串 24":dbl}, "1 33":cluster{"第181串":dbl, "第182串":dbl, "第183串":dbl, "第184串":dbl, "第185串":dbl, "第186串":dbl, "第187串":dbl, "第188串":dbl, "第189串":dbl, "第190串":dbl, "第191串":dbl, "第192串":dbl, "第一串 2":dbl, "第一串 4":dbl, "第一串 6":dbl, "第一串 8":dbl, "第一串 10":dbl, "第一串 12":dbl, "第一串 14":dbl, "第一串 16":dbl, "第一串 18":dbl, "第一串 20":dbl, "第一串 22":dbl, "第一串 24":dbl}}
  T12 = cluster{"1 18":cluster{"第193串":dbl, "第194串":dbl, "第195串":dbl, "第196串":dbl, "第197串":dbl, "第198串":dbl, "第199串":dbl, "第200串":dbl, "第201串":dbl, "第202串":dbl, "第203串":dbl, "第204串":dbl, "第一串 2":dbl, "第一串 4":dbl, "第一串 6":dbl, "第一串 8":dbl, "第一串 10":dbl, "第一串 12":dbl, "第一串 14":dbl, "第一串 16":dbl, "第一串 18":dbl, "第一串 20":dbl, "第一串 22":dbl, "第一串 24":dbl}, "1 19":cluster{"第205串":dbl, "第206串":dbl, "第207串":dbl, "第208串":dbl, "第209串":dbl, "第210串":dbl, "第211串":dbl, "第212串":dbl, "第213串":dbl, "第214串":dbl, "第215串":dbl, "第216串":dbl, "第一串 2":dbl, "第一串 4":dbl, "第一串 6":dbl, "第一串 8":dbl, "第一串 10":dbl, "第一串 12":dbl, "第一串 14":dbl, "第一串 16":dbl, "第一串 18":dbl, "第一串 20":dbl, "第一串 22":dbl, "第一串 24":dbl}, "1 20":cluster{"第217串":dbl, "第218串":dbl, "第219串":dbl, "第220串":dbl, "第221串":dbl, "第222串":dbl, "第223串":dbl, "第224串":dbl, "第225串":dbl, "第226串":dbl, "第227串":dbl, "第228串":dbl, "第一串 2":dbl, "第一串 4":dbl, "第一串 6":dbl, "第一串 8":dbl, "第一串 10":dbl, "第一串 12":dbl, "第一串 14":dbl, "第一串 16":dbl, "第一串 18":dbl, "第一串 20":dbl, "第一串 22":dbl, "第一串 24":dbl}, "1 21":cluster{"第229串":dbl, "第230串":dbl, "第231串":dbl, "第232串":dbl, "第233串":dbl, "第234串":dbl, "第235串":dbl, "第236串":dbl, "第237串":dbl, "第238串":dbl, "第239串":dbl, "第240串":dbl, "第一串 2":dbl, "第一串 4":dbl, "第一串 6":dbl, "第一串 8":dbl, "第一串 10":dbl, "第一串 12":dbl, "第一串 14":dbl, "第一串 16":dbl, "第一串 18":dbl, "第一串 20":dbl, "第一串 22":dbl, "第一串 24":dbl}, "1 22":cluster{"第241串":dbl, "第242串":dbl, "第243串":dbl, "第244串":dbl, "第245串":dbl, "第246串":dbl, "第247串":dbl, "第248串":dbl, "第249串":dbl, "第250串":dbl, "第251串":dbl, "第252串":dbl, "第一串 2":dbl, "第一串 4":dbl, "第一串 6":dbl, "第一串 8":dbl, "第一串 10":dbl, "第一串 12":dbl, "第一串 14":dbl, "第一串 16":dbl, "第一串 18":dbl, "第一串 20":dbl, "第一串 22":dbl, "第一串 24":dbl}, "1 23":cluster{"第253串":dbl, "第254串":dbl, "第255串":dbl, "第256串":dbl, "第257串":dbl, "第258串":dbl, "第259串":dbl, "第260串":dbl, "第261串":dbl, "第262串":dbl, "第263串":dbl, "第264串":dbl, "第一串 2":dbl, "第一串 4":dbl, "第一串 6":dbl, "第一串 8":dbl, "第一串 10":dbl, "第一串 12":dbl, "第一串 14":dbl, "第一串 16":dbl, "第一串 18":dbl, "第一串 20":dbl, "第一串 22":dbl, "第一串 24":dbl}, "1 24":cluster{"第265串":dbl, "第266串":dbl, "第267串":dbl, "第268串":dbl, "第269串":dbl, "第270串":dbl, "第271串":dbl, "第272串":dbl, "第273串":dbl, "第274串":dbl, "第275串":dbl, "第276串":dbl, "第一串 2":dbl, "第一串 4":dbl, "第一串 6":dbl, "第一串 8":dbl, "第一串 10":dbl, "第一串 12":dbl, "第一串 14":dbl, "第一串 16":dbl, "第一串 18":dbl, "第一串 20":dbl, "第一串 22":dbl, "第一串 24":dbl}, "1 25":cluster{"第277串":dbl, "第278串":dbl, "第279串":dbl, "第280串":dbl, "第281串":dbl, "第282串":dbl, "第283串":dbl, "第284串":dbl, "第285串":dbl, "第286串":dbl, "第287串":dbl, "第288串":dbl, "第一串 2":dbl, "第一串 4":dbl, "第一串 6":dbl, "第一串 8":dbl, "第一串 10":dbl, "第一串 12":dbl, "第一串 14":dbl, "第一串 16":dbl, "第一串 18":dbl, "第一串 20":dbl, "第一串 22":dbl, "第一串 24":dbl}}
  T13 = cluster{"1 3":cluster{"第13串":dbl, "第14串":dbl, "第15串":dbl, "第16串":dbl, "第17串":dbl, "第18串":dbl, "第19串":dbl, "第20串":dbl, "第21串":dbl, "第22串":dbl, "第23串":dbl, "第24串":dbl, "第一串 2":dbl, "第一串 4":dbl, "第一串 6":dbl, "第一串 8":dbl, "第一串 10":dbl, "第一串 12":dbl, "第一串 14":dbl, "第一串 16":dbl, "第一串 18":dbl, "第一串 20":dbl, "第一串 22":dbl, "第一串 24":dbl}, "1 4":cluster{"第25串":dbl, "第26串":dbl, "第27串":dbl, "第28串":dbl, "第29串":dbl, "第30串":dbl, "第31串":dbl, "第32串":dbl, "第33串":dbl, "第34串":dbl, "第35串":dbl, "第36串":dbl, "第一串 2":dbl, "第一串 4":dbl, "第一串 6":dbl, "第一串 8":dbl, "第一串 10":dbl, "第一串 12":dbl, "第一串 14":dbl, "第一串 16":dbl, "第一串 18":dbl, "第一串 20":dbl, "第一串 22":dbl, "第一串 24":dbl}, "1 6":cluster{"第37串":dbl, "第38串":dbl, "第39串":dbl, "第40串":dbl, "第41串":dbl, "第42串":dbl, "第43串":dbl, "第44串":dbl, "第45串":dbl, "第46串":dbl, "第47串":dbl, "第48串":dbl, "第一串 2":dbl, "第一串 4":dbl, "第一串 6":dbl, "第一串 8":dbl, "第一串 10":dbl, "第一串 12":dbl, "第一串 14":dbl, "第一串 16":dbl, "第一串 18":dbl, "第一串 20":dbl, "第一串 22":dbl, "第一串 24":dbl}, "1 7":cluster{"第49串":dbl, "第50串":dbl, "第51串":dbl, "第52串":dbl, "第53串":dbl, "第54串":dbl, "第55串":dbl, "第56串":dbl, "第57串":dbl, "第58串":dbl, "第59串":dbl, "第60串":dbl, "第一串 2":dbl, "第一串 4":dbl, "第一串 6":dbl, "第一串 8":dbl, "第一串 10":dbl, "第一串 12":dbl, "第一串 14":dbl, "第一串 16":dbl, "第一串 18":dbl, "第一串 20":dbl, "第一串 22":dbl, "第一串 24":dbl}, "1 8":cluster{"第61串":dbl, "第62串":dbl, "第63串":dbl, "第64串":dbl, "第65串":dbl, "第66串":dbl, "第67串":dbl, "第68串":dbl, "第69串":dbl, "第70串":dbl, "第71串":dbl, "第72串":dbl, "第一串 2":dbl, "第一串 4":dbl, "第一串 6":dbl, "第一串 8":dbl, "第一串 10":dbl, "第一串 12":dbl, "第一串 14":dbl, "第一串 16":dbl, "第一串 18":dbl, "第一串 20":dbl, "第一串 22":dbl, "第一串 24":dbl}, "1 9":cluster{"第73串":dbl, "第74串":dbl, "第75串":dbl, "第76串":dbl, "第77串":dbl, "第78串":dbl, "第79串":dbl, "第80串":dbl, "第81串":dbl, "第82串":dbl, "第83串":dbl, "第84串":dbl, "第一串 2":dbl, "第一串 4":dbl, "第一串 6":dbl, "第一串 8":dbl, "第一串 10":dbl, "第一串 12":dbl, "第一串 14":dbl, "第一串 16":dbl, "第一串 18":dbl, "第一串 20":dbl, "第一串 22":dbl, "第一串 24":dbl}, "1 10":cluster{"第85串":dbl, "第86串":dbl, "第87串":dbl, "第88串":dbl, "第89串":dbl, "第90串":dbl, "第91串":dbl, "第92串":dbl, "第93串":dbl, "第94串":dbl, "第95串":dbl, "第96串":dbl, "第一串 2":dbl, "第一串 4":dbl, "第一串 6":dbl, "第一串 8":dbl, "第一串 10":dbl, "第一串 12":dbl, "第一串 14":dbl, "第一串 16":dbl, "第一串 18":dbl, "第一串 20":dbl, "第一串 22":dbl, "第一串 24":dbl}, "1 102":cluster{"第1串":dbl, "第2串":dbl, "第3串":dbl, "第4串":dbl, "第5串":dbl, "第6串":dbl, "第7串":dbl, "第8串":dbl, "第9串":dbl, "第10串":dbl, "第11串":dbl, "第12串":dbl, "第一串 2":dbl, "第一串 4":dbl, "第一串 6":dbl, "第一串 8":dbl, "第一串 10":dbl, "第一串 12":dbl, "第一串 14":dbl, "第一串 16":dbl, "第一串 18":dbl, "第一串 20":dbl, "第一串 22":dbl, "第一串 24":dbl}}
  T14 = cluster{"[0]":u32, "[1]":u32, "[2]":u32, "[3]":u32, "[4]":u32, "[5]":u32, "[6]":u32, "[7]":u32, "[8]":u32, "[9]":u32, "[10]":u32, "[11]":u32}
  T15 = cluster{"[0]":dbl, "[1]":dbl, "[2]":dbl, "[3]":dbl, "[4]":dbl, "[5]":dbl, "[6]":dbl, "[7]":dbl, "[8]":dbl, "[9]":dbl, "[10]":dbl, "[11]":dbl}
  T16 = cluster{"[0]":dbl, "[1]":dbl, "[2]":dbl, "[3]":dbl, "[4]":dbl, "[5]":dbl, "[6]":dbl, "[7]":dbl, "[8]":dbl, "[9]":dbl, "[10]":dbl, "[11]":dbl, "[12]":dbl, "[13]":dbl, "[14]":dbl, "[15]":dbl, "[16]":dbl, "[17]":dbl, "[18]":dbl, "[19]":dbl, "[20]":dbl, "[21]":dbl, "[22]":dbl, "[23]":dbl}
  T17 = enum32{"Invalid", "Standard", "Closed", "Hidden", "Minimized", "Maximized"}
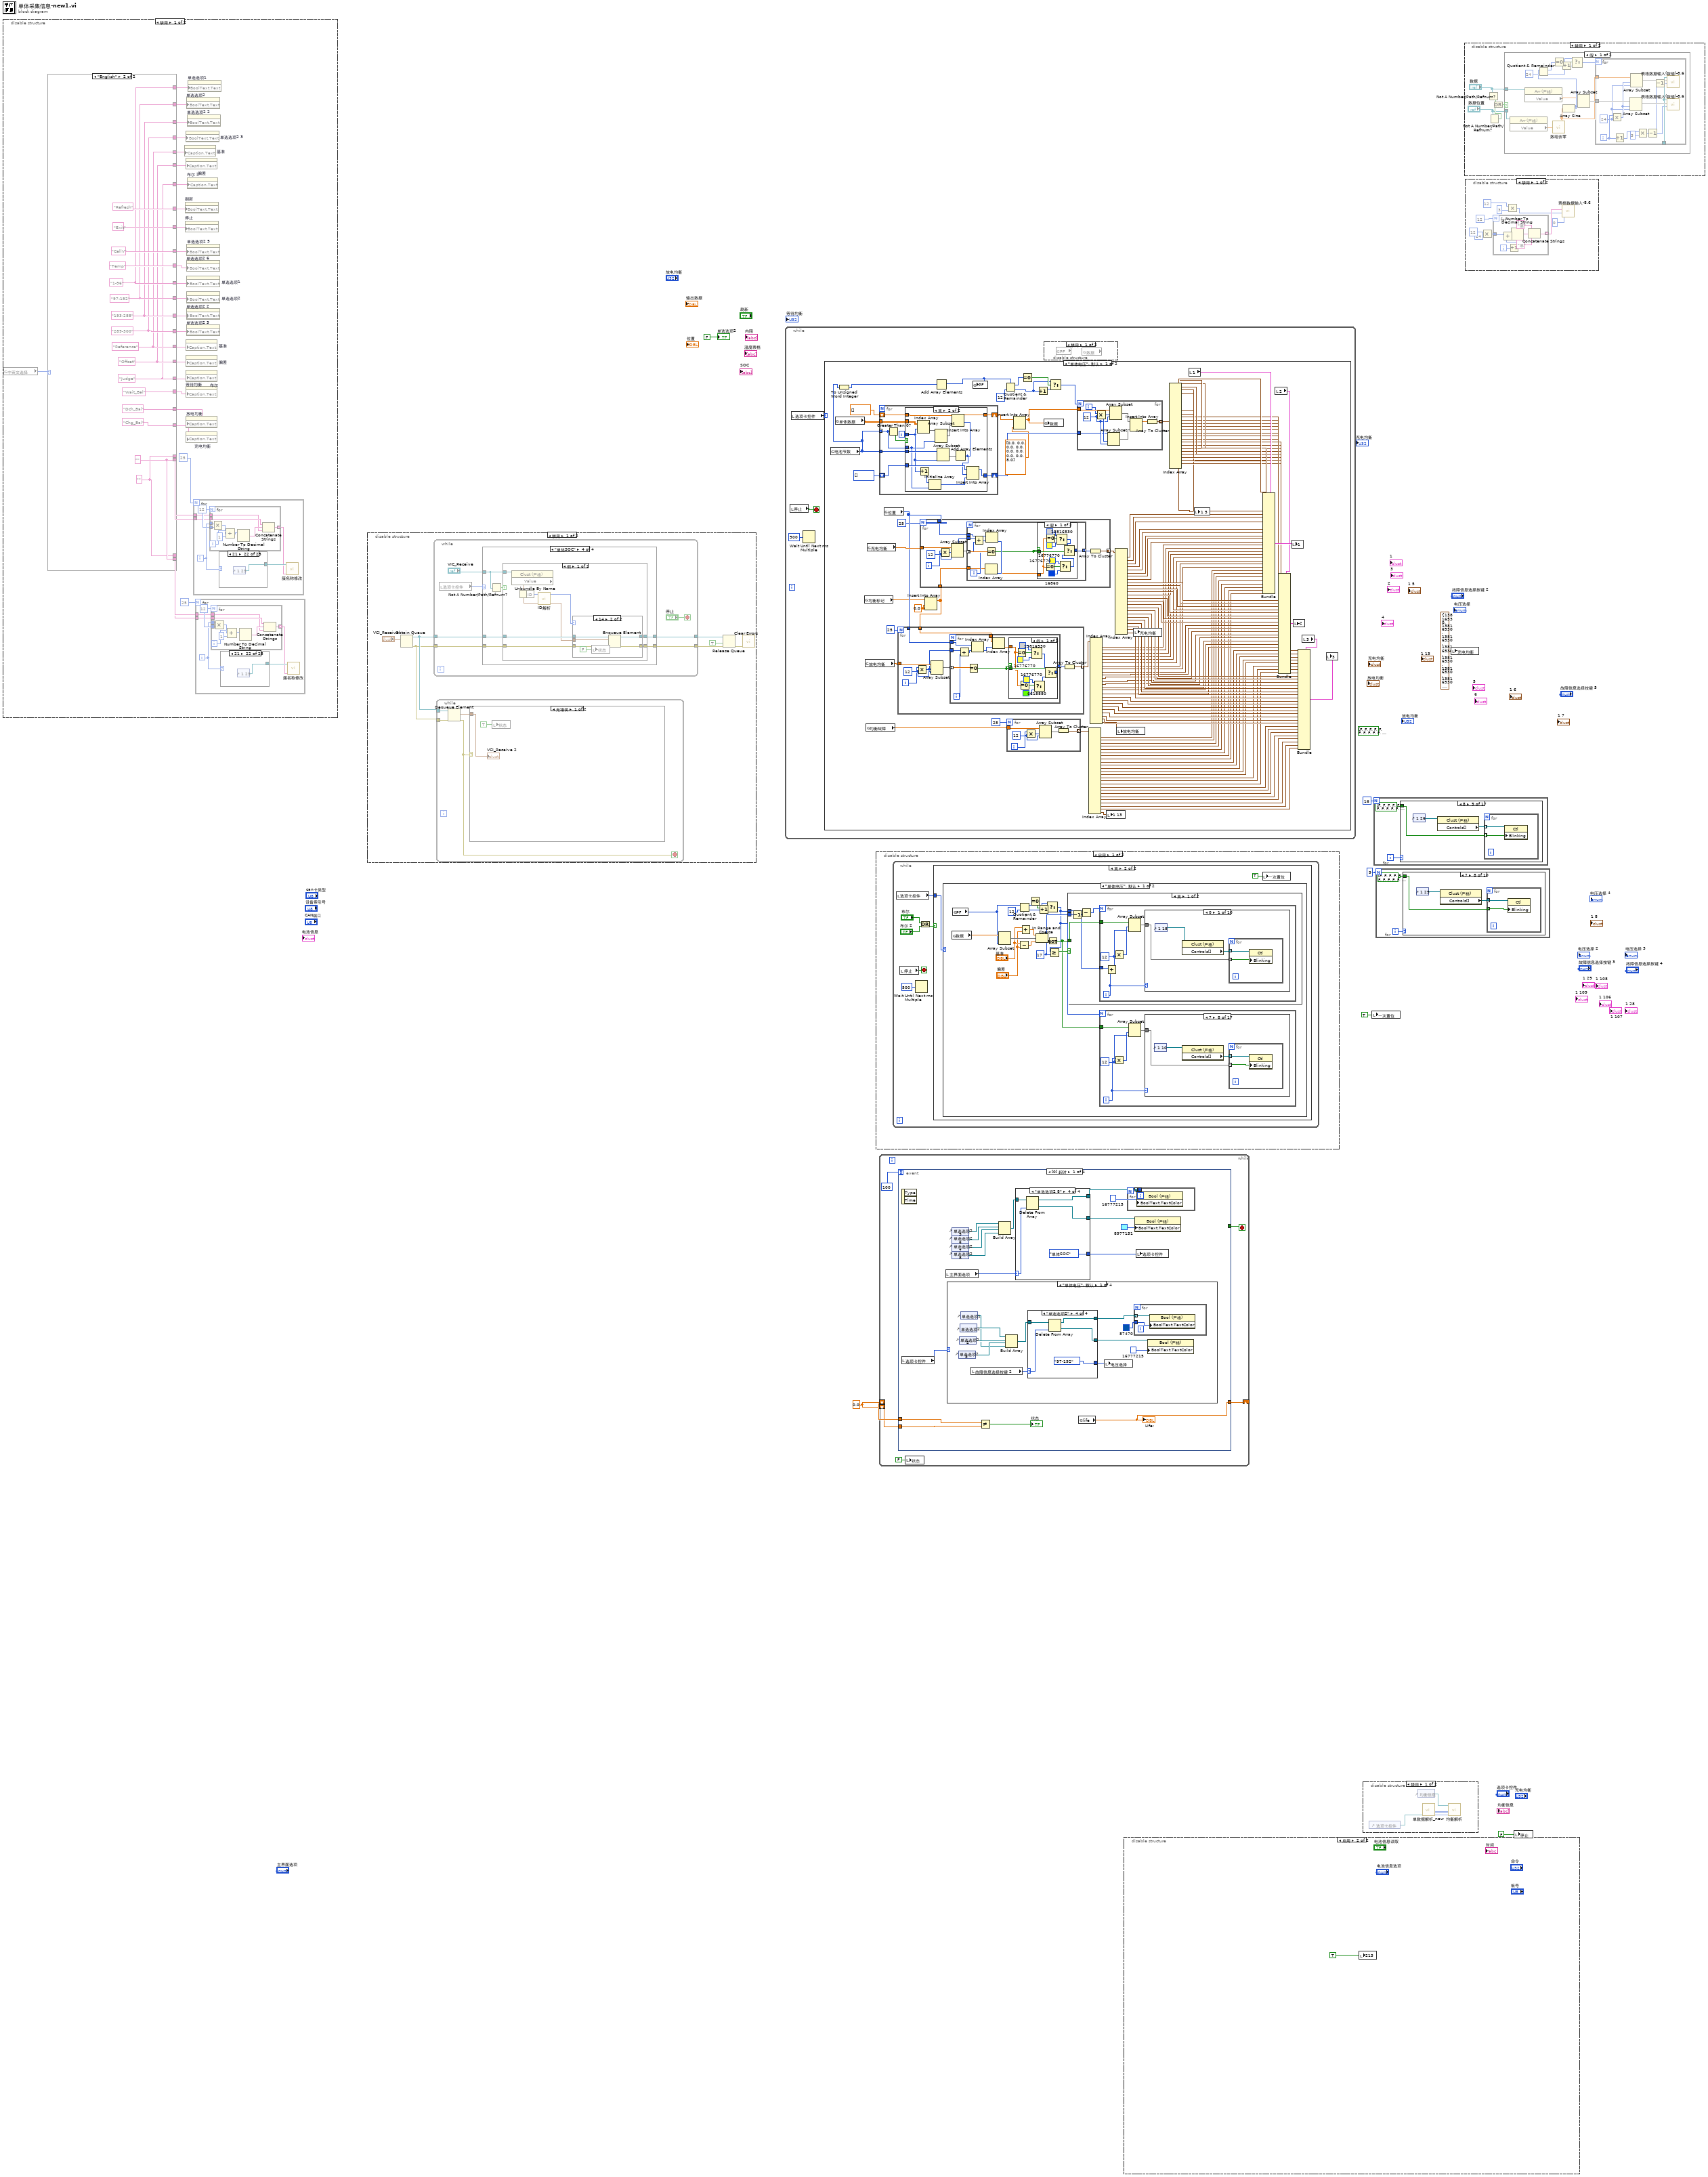
[diagram p0: block diagram]
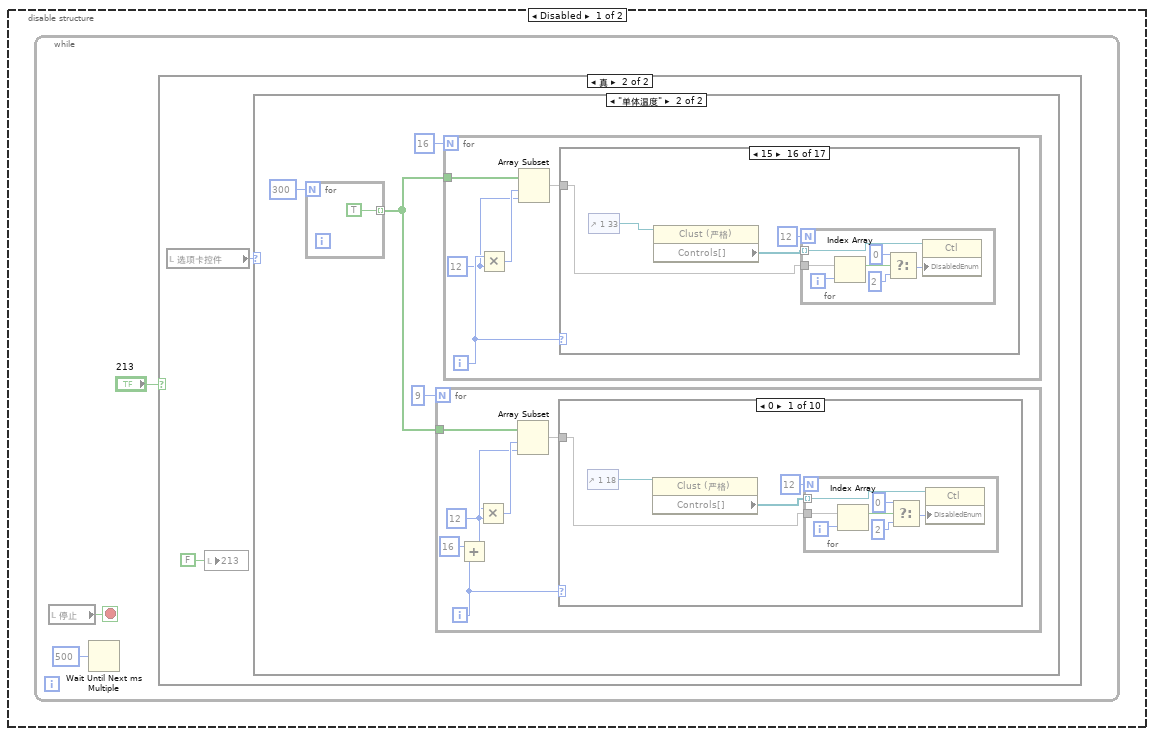
[diagram p2: hidden frame]
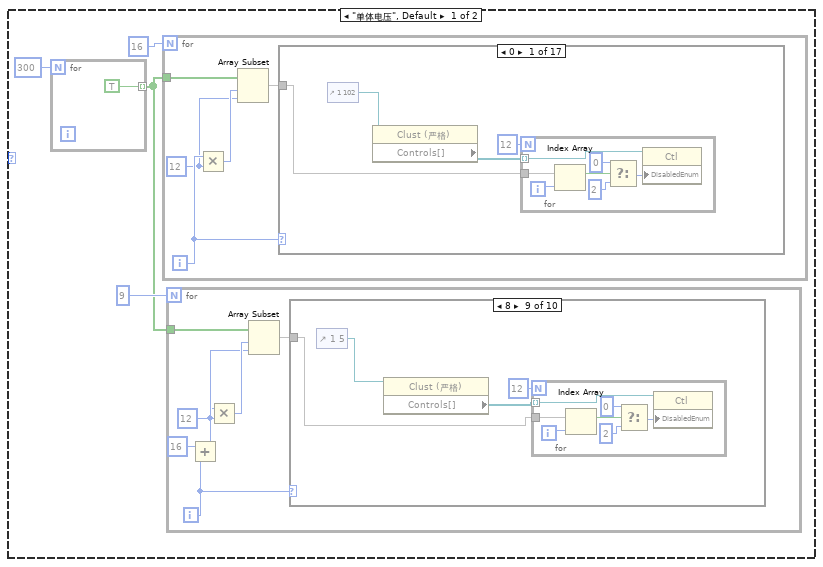
[diagram p4: hidden frame]
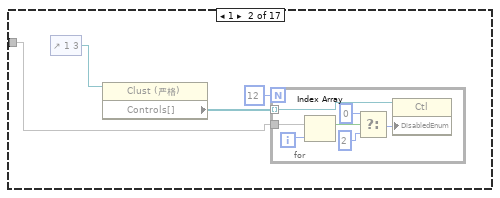
[diagram p5: hidden frame]
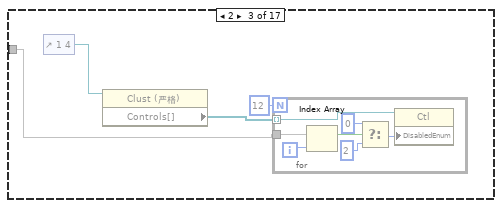
[diagram p6: hidden frame]
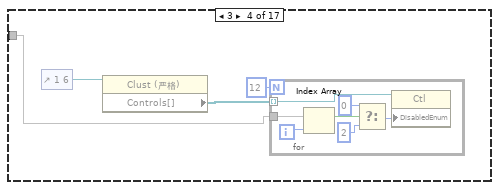
[diagram p7: hidden frame]
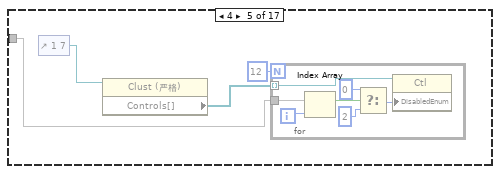
[diagram p8: hidden frame]
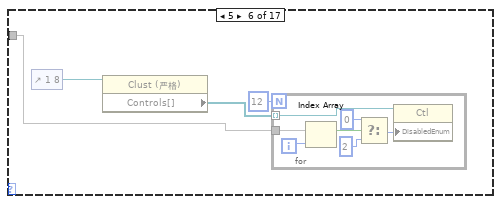
[diagram p9: hidden frame]
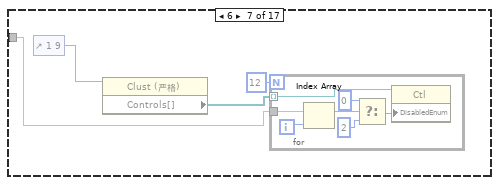
[diagram p10: hidden frame]
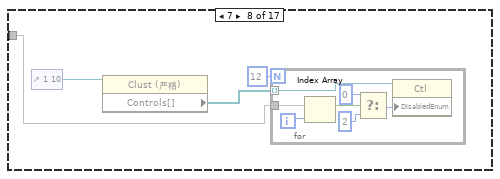
[diagram p11: hidden frame]
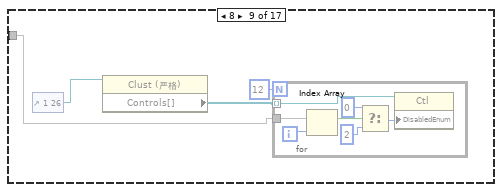
[diagram p12: hidden frame]
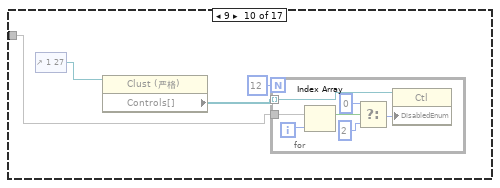
[diagram p13: hidden frame]
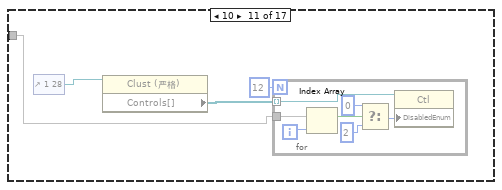
[diagram p14: hidden frame]
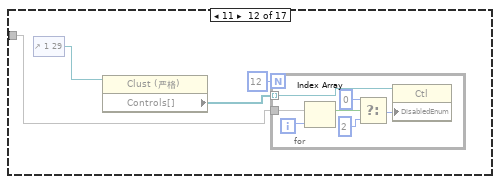
[diagram p15: hidden frame]
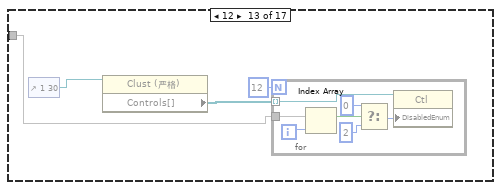
[diagram p16: hidden frame]
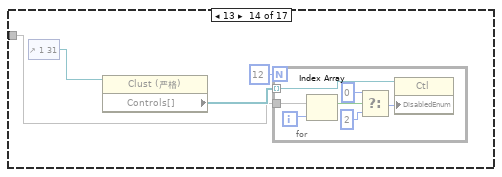
[diagram p17: hidden frame]
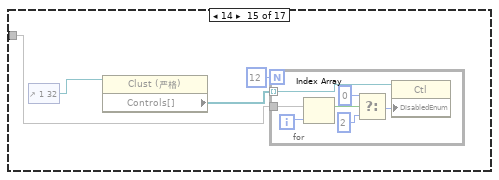
[diagram p18: hidden frame]
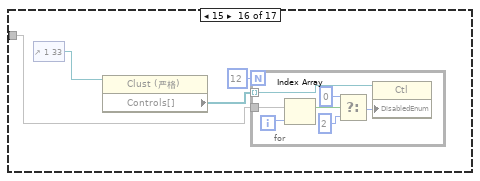
[diagram p19: hidden frame]
diagram:
  w1 = 0.0 ("life")
  (unwired) bool[] [FALSE, FALSE, FALSE, FALSE, FALSE, FALSE, FALSE, FALSE, FALSE, FALSE, FALSE, FALSE, FALSE]
  n1 = disable-structure shown="禁用" {
    frame Disabled {
      n2 = global read "中英文全局.vi" "中英文选择"() -> (w36:enum32{"中文", "English"})
      n3 = case shown="\"English\"" w36 {
        tunnel: ["单体电压" "CellV"] -> w35
        tunnel: ["单体温度" "Temp"] -> w34
        tunnel: [w125 w141] -> w33
        tunnel: [w124 w140] -> w32
        tunnel: [w123 w139] -> w31
        tunnel: [w122 w138] -> w30
        tunnel: [w121 w137] -> w29
        tunnel: [w120 w136] -> w28
        tunnel: [w119 w135] -> w27
        tunnel: ["等待均衡" "Wait_Bal"] -> w26
        tunnel: ["放电均衡" "Dch_Bal"] -> w25
        tunnel: ["充电均衡" "Chg_Bal"] -> w24
        tunnel: [w129 w145] -> w22
        tunnel: [w128 w144] -> w21
        tunnel: [w129 w145] -> w19
        tunnel: [w128 w144] -> w20
        tunnel: ["刷新" "Refresh"] -> w17
        tunnel: ["退出" "Exit"] -> w16
        tunnel: [w125 w141] -> w15
        tunnel: [w124 w140] -> w14
        tunnel: [w123 w139] -> w13
        tunnel: [w122 w138] -> w12
        tunnel: [w121 w137] -> w11
        tunnel: [w120 w136] -> w10
        tunnel: [w119 w135] -> w9
        frame "中文", Default {
          w128 = "串"
          w129 = "第"
          w119 = "判定"
          w120 = "偏差"
          w121 = "基准"
          w122 = "289串-300串"
          w123 = "193串-288串"
          w124 = "97串-192串"
          w125 = "1串-96串"
        }
        frame "English" {
          w144 = ""
          w145 = ""
          w135 = "Judge"
          w136 = "Offset"
          w137 = "Reference"
          w138 = "289-300"
          w139 = "193-288"
          w140 = "97-192"
          w141 = "1-96"
        }
      }
      n4 = property on="基准" class="DigNum (严格)"("Caption.Text"=w11) -> ()  [unwired: 2 in, 2 out]
      n5 = property on="刷新" class="Bool (严格)"("BoolText.Text"=w17) -> ()  [unwired: 2 in, 2 out]
      n6 = property on="停止" class="Bool (严格)"("BoolText.Text"=w16) -> ()  [unwired: 2 in, 2 out]
      n7 = property on="单选选项2 3" class="Bool (严格)"("BoolText.Text"=w12) -> ()  [unwired: 2 in, 2 out]
      n8 = property on="偏差" class="DigNum (严格)"("Caption.Text"=w10) -> ()  [unwired: 2 in, 2 out]
      n9 = property on="基准" class="DigNum (严格)"("Caption.Text"=w29) -> ()  [unwired: 2 in, 2 out]
      n10 = property on="偏差" class="DigNum (严格)"("Caption.Text"=w28) -> ()  [unwired: 2 in, 2 out]
      n11 = property on="布尔" class="Bool (严格)"("Caption.Text"=w27) -> ()  [unwired: 2 in, 2 out]
      n12 = property on="等待均衡" class="ColBox"("Caption.Text"=w26) -> ()  [unwired: 2 in, 2 out]
      n13 = property on="放电均衡" class="ColBox"("Caption.Text"=w25) -> ()  [unwired: 2 in, 2 out]
      n14 = property on="充电均衡" class="ColBox"("Caption.Text"=w24) -> ()  [unwired: 2 in, 2 out]
      n15 = property on="单选选项2" class="Bool (严格)"("BoolText.Text"=w14) -> ()  [unwired: 2 in, 2 out]
      n16 = property on="单选选项2 5" class="Bool (严格)"("BoolText.Text"=w35) -> ()  [unwired: 2 in, 2 out]
      n17 = property on="单选选项2 6" class="Bool (严格)"("BoolText.Text"=w34) -> ()  [unwired: 2 in, 2 out]
      n18 = property on="单选选项1" class="Bool (严格)"("BoolText.Text"=w33) -> ()  [unwired: 2 in, 2 out]
      n19 = property on="单选选项2" class="Bool (严格)"("BoolText.Text"=w32) -> ()  [unwired: 2 in, 2 out]
      n20 = property on="单选选项2 2" class="Bool (严格)"("BoolText.Text"=w31) -> ()  [unwired: 2 in, 2 out]
      n21 = property on="单选选项2 3" class="Bool (严格)"("BoolText.Text"=w30) -> ()  [unwired: 2 in, 2 out]
      n22 = property on="单选选项2 2" class="Bool (严格)"("BoolText.Text"=w13) -> ()  [unwired: 2 in, 2 out]
      n23 = property on="布尔 2" class="Bool (严格)"("Caption.Text"=w9) -> ()  [unwired: 2 in, 2 out]
      n24 = property on="单选选项1" class="Bool (严格)"("BoolText.Text"=w15) -> ()  [unwired: 2 in, 2 out]
      n25 = for {
        N: 25 -> [_]
        tunnel: w22 -> [w79]
        tunnel: w21 -> [w78]
        i -> [w80]
        w83 = 12
        n26 = for {
          N: w83 -> [_]
          tunnel: [w117] -> w81 mode=indexing
          tunnel: w80 -> [w114]
          tunnel: w83 -> [w113]
          tunnel: w79 -> [w110]
          tunnel: w78 -> [w109]
          i -> [w116]
          n27 = Multiply(x=w114, y=w113) -> (x*y=w115:i32)
          n28 = Compound Arithmetic op=ADD(w116, w115, 1 ("值")) -> (w111:i32)
          n29 = Number To Decimal String(number=w111) -> (decimal integer string=w118:string)  [unwired: 1 in]
          n30 = Concatenate Strings(w110, w118, w109) -> (w117:string)
        }
        n31 = case shown="21" w80 {
          tunnel: [w84 w85 w86 w87 w88 w89 w90 w91 w92 w93 w94 w95 w96 w97 w98 w99 w100 w101 w102 w103 w104 w105 w106 w107 w108] -> w82
          frame 0, Default {
            n32 = control-ref of="1 102"() -> (w84:refnum<vi>)
          }
          frame 1 {
            n33 = control-ref of="1 3"() -> (w85:refnum<vi>)
          }
          frame 2 {
            n34 = control-ref of="1 4"() -> (w86:refnum<vi>)
          }
          frame 3 {
            n35 = control-ref of="1 6"() -> (w87:refnum<vi>)
          }
          frame 4 {
            n36 = control-ref of="1 7"() -> (w88:refnum<vi>)
          }
          frame 5 {
            n37 = control-ref of="1 8"() -> (w89:refnum<vi>)
          }
          frame 6 {
            n38 = control-ref of="1 9"() -> (w90:refnum<vi>)
          }
          frame 7 {
            n39 = control-ref of="1 10"() -> (w91:refnum<vi>)
          }
          frame 8 {
            n40 = control-ref of="1 26"() -> (w92:refnum<vi>)
          }
          frame 9 {
            n41 = control-ref of="1 27"() -> (w93:refnum<vi>)
          }
          frame 10 {
            n42 = control-ref of="1 28"() -> (w94:refnum<vi>)
          }
          frame 11 {
            n43 = control-ref of="1 29"() -> (w95:refnum<vi>)
          }
          frame 12 {
            n44 = control-ref of="1 30"() -> (w96:refnum<vi>)
          }
          frame 13 {
            n45 = control-ref of="1 31"() -> (w97:refnum<vi>)
          }
          frame 14 {
            n46 = control-ref of="1 32"() -> (w98:refnum<vi>)
          }
          frame 15 {
            n47 = control-ref of="1 33"() -> (w99:refnum<vi>)
          }
          frame 16 {
            n48 = control-ref of="1 18"() -> (w100:refnum<vi>)
          }
          frame 17 {
            n49 = control-ref of="1 19"() -> (w101:refnum<vi>)
          }
          frame 18 {
            n50 = control-ref of="1 20"() -> (w102:refnum<vi>)
          }
          frame 19 {
            n51 = control-ref of="1 21"() -> (w103:refnum<vi>)
          }
          frame 20 {
            n52 = control-ref of="1 22"() -> (w104:refnum<vi>)
          }
          frame 21 {
            n53 = control-ref of="1 23"() -> (w105:refnum<vi>)
          }
          frame 22 {
            n54 = control-ref of="1 24"() -> (w106:refnum<vi>)
          }
          frame 23 {
            n55 = control-ref of="1 25"() -> (w107:refnum<vi>)
          }
          frame 24 {
            n56 = control-ref of="1 5"() -> (w108:refnum<vi>)
          }
        }
        n57 = call "簇名称修改.vi"("输入名称"=w81, "簇引用"=w82) -> ()  [unwired: 10 in]
      }
      n58 = for {
        N: 25 -> [_]
        tunnel: w19 -> [w38]
        tunnel: w20 -> [w37]
        i -> [w39]
        w42 = 12
        n59 = for {
          N: w42 -> [_]
          tunnel: [w76] -> w40 mode=indexing
          tunnel: w39 -> [w73]
          tunnel: w42 -> [w72]
          tunnel: w38 -> [w69]
          tunnel: w37 -> [w68]
          i -> [w75]
          n60 = Multiply(x=w73, y=w72) -> (x*y=w74:i32)
          n61 = Compound Arithmetic op=ADD(w75, w74, 1 ("值")) -> (w70:i32)
          n62 = Number To Decimal String(number=w70) -> (decimal integer string=w77:string)  [unwired: 1 in]
          n63 = Concatenate Strings(w69, w77, w68) -> (w76:string)
        }
        n64 = case shown="21" w39 {
          tunnel: [w43 w44 w45 w46 w47 w48 w49 w50 w51 w52 w53 w54 w55 w56 w57 w58 w59 w60 w61 w62 w63 w64 w65 w66 w67] -> w41
          frame 0, Default {
            n65 = control-ref of="1 102"() -> (w43:refnum<vi>)
          }
          frame 1 {
            n66 = control-ref of="1 3"() -> (w44:refnum<vi>)
          }
          frame 2 {
            n67 = control-ref of="1 4"() -> (w45:refnum<vi>)
          }
          frame 3 {
            n68 = control-ref of="1 6"() -> (w46:refnum<vi>)
          }
          frame 4 {
            n69 = control-ref of="1 7"() -> (w47:refnum<vi>)
          }
          frame 5 {
            n70 = control-ref of="1 8"() -> (w48:refnum<vi>)
          }
          frame 6 {
            n71 = control-ref of="1 9"() -> (w49:refnum<vi>)
          }
          frame 7 {
            n72 = control-ref of="1 10"() -> (w50:refnum<vi>)
          }
          frame 8 {
            n73 = control-ref of="1 26"() -> (w51:refnum<vi>)
          }
          frame 9 {
            n74 = control-ref of="1 27"() -> (w52:refnum<vi>)
          }
          frame 10 {
            n75 = control-ref of="1 28"() -> (w53:refnum<vi>)
          }
          frame 11 {
            n76 = control-ref of="1 29"() -> (w54:refnum<vi>)
          }
          frame 12 {
            n77 = control-ref of="1 30"() -> (w55:refnum<vi>)
          }
          frame 13 {
            n78 = control-ref of="1 31"() -> (w56:refnum<vi>)
          }
          frame 14 {
            n79 = control-ref of="1 32"() -> (w57:refnum<vi>)
          }
          frame 15 {
            n80 = control-ref of="1 33"() -> (w58:refnum<vi>)
          }
          frame 16 {
            n81 = control-ref of="1 18"() -> (w59:refnum<vi>)
          }
          frame 17 {
            n82 = control-ref of="1 19"() -> (w60:refnum<vi>)
          }
          frame 18 {
            n83 = control-ref of="1 20"() -> (w61:refnum<vi>)
          }
          frame 19 {
            n84 = control-ref of="1 21"() -> (w62:refnum<vi>)
          }
          frame 20 {
            n85 = control-ref of="1 22"() -> (w63:refnum<vi>)
          }
          frame 21 {
            n86 = control-ref of="1 23"() -> (w64:refnum<vi>)
          }
          frame 22 {
            n87 = control-ref of="1 24"() -> (w65:refnum<vi>)
          }
          frame 23 {
            n88 = control-ref of="1 25"() -> (w66:refnum<vi>)
          }
          frame 24 {
            n89 = control-ref of="1 6"() -> (w67:refnum<vi>)
          }
        }
        n90 = call "簇名称修改.vi"("输入名称"=w40, "簇引用"=w41) -> ()  [unwired: 10 in]
      }
    }
    frame Enabled {
    }
  }
  n91 = disable-structure shown="禁用" {
    frame Disabled {
      n92 = Obtain Queue(element data type="VCI_Receive") -> (queue out=w156:refnum<queue>, error out=w155:errorcluster)  [unwired: 4 in, 1 out]
      n93 = while {
        tunnel: w156 -> [w167]
        tunnel: w155 -> [w166]
        tunnel: [w165] -> w154
        tunnel: [w164] -> w153
        stop <- "停止" stop-if-true
        n94 = local read "选项卡控件"() -> (w168:enum32{"单体电压", "单体温度", "单体内阻", "单体SOC"})
        n95 = case shown="\"单体SOC\"" w168 {
          tunnel: "VIC_Receive" -> [w172 w196 w220 w244]
          tunnel: w167 -> [w176 w200 w224 w248]
          tunnel: w166 -> [w175 w199 w223 w247]
          tunnel: [w174 w198 w222 w246] -> w165
          tunnel: [w173 w197 w221 w245] -> w164
          frame "单体电压", Default {
            n96 = Not A Number/Path/Refnum?(number/path/refnum=w172) -> (NaN/Path/Refnum?=w171:bool)
            n97 = case shown="假" w171 {
              tunnel: w176 -> [w183 w194]
              tunnel: w175 -> [w182 w193]
              tunnel: [w180 w194] -> w174
              tunnel: [w179 w193] -> w173
              tunnel: w172 -> [w178 _]
              frame False {
                n98 = property class="Clust (严格)"(reference=w178) -> ("Value"=w181:T1)  [unwired: 1 in, 2 out]
                n99 = Unbundle By Name(w181) -> ("ID"=w184:u32)
                n100 = call "ID解析.vi"("ID"=w184) -> ("PDU(1)"=w177:i32)  [unwired: 10 out]
                n101 = case shown="8" w177 {
                  tunnel: w183 -> [w186 w192]
                  tunnel: w182 -> [w185 w191]
                  tunnel: w181 -> [_ w190]
                  tunnel: [w186 w189] -> w180
                  tunnel: [w185 w188] -> w179
                  frame 0, Default {
                  }
                  frame 8 {
                    n102 = local write "状态"(FALSE ("状态")) -> ()
                    n103 = Enqueue Element(queue=w192, element=w190, error in (no error)=w191) -> (queue out=w189:refnum<queue>, error out=w188:errorcluster)  [unwired: 2 out]
                  }
                }
              }
              frame True {
              }
            }
          }
          frame "单体温度" {
            n104 = Not A Number/Path/Refnum?(number/path/refnum=w196) -> (NaN/Path/Refnum?=w195:bool)
            n105 = case shown="假" w195 {
              tunnel: w200 -> [w207 w218]
              tunnel: w199 -> [w206 w217]
              tunnel: [w205 w218] -> w198
              tunnel: [w204 w217] -> w197
              tunnel: w196 -> [w203 _]
              frame False {
                n106 = property class="Clust (严格)"(reference=w203) -> ("Value"=w201:T1)  [unwired: 1 in, 2 out]
                n107 = Unbundle By Name(w201) -> ("ID"=w208:u32)
                n108 = call "ID解析.vi"("ID"=w208) -> ("PDU(1)"=w202:i32)  [unwired: 10 out]
                n109 = case shown="10" w202 {
                  tunnel: w207 -> [w210 w216]
                  tunnel: w206 -> [w209 w215]
                  tunnel: w201 -> [_ w214]
                  tunnel: [w210 w213] -> w205
                  tunnel: [w209 w212] -> w204
                  frame 0, Default {
                  }
                  frame 16 {
                    n110 = local write "状态"(FALSE ("状态")) -> ()
                    n111 = Enqueue Element(queue=w216, element=w214, error in (no error)=w215) -> (queue out=w213:refnum<queue>, error out=w212:errorcluster)  [unwired: 2 out]
                  }
                }
              }
              frame True {
              }
            }
          }
          frame "单体内阻" {
            n112 = Not A Number/Path/Refnum?(number/path/refnum=w220) -> (NaN/Path/Refnum?=w219:bool)
            n113 = case shown="假" w219 {
              tunnel: w224 -> [w231 w242]
              tunnel: w223 -> [w230 w241]
              tunnel: [w228 w242] -> w222
              tunnel: [w227 w241] -> w221
              tunnel: w220 -> [w226 _]
              frame False {
                n114 = property class="Clust (严格)"(reference=w226) -> ("Value"=w229:T1)  [unwired: 1 in, 2 out]
                n115 = Unbundle By Name(w229) -> ("ID"=w232:u32)
                n116 = call "ID解析.vi"("ID"=w232) -> ("PDU(1)"=w225:i32)  [unwired: 10 out]
                n117 = case shown="C" w225 {
                  tunnel: w231 -> [w234 w240]
                  tunnel: w230 -> [w233 w239]
                  tunnel: w229 -> [_ w238]
                  tunnel: [w234 w237] -> w228
                  tunnel: [w233 w236] -> w227
                  frame 0, Default {
                  }
                  frame 12 {
                    n118 = local write "状态"(FALSE ("状态")) -> ()
                    n119 = Enqueue Element(queue=w240, element=w238, error in (no error)=w239) -> (queue out=w237:refnum<queue>, error out=w236:errorcluster)  [unwired: 2 out]
                  }
                }
              }
              frame True {
              }
            }
          }
          frame "单体SOC" {
            n120 = Not A Number/Path/Refnum?(number/path/refnum=w244) -> (NaN/Path/Refnum?=w243:bool)
            n121 = case shown="假" w243 {
              tunnel: w248 -> [w255 w266]
              tunnel: w247 -> [w254 w265]
              tunnel: [w252 w266] -> w246
              tunnel: [w251 w265] -> w245
              tunnel: w244 -> [w250 _]
              frame False {
                n122 = property class="Clust (严格)"(reference=w250) -> ("Value"=w253:T1)  [unwired: 1 in, 2 out]
                n123 = Unbundle By Name(w253) -> ("ID"=w256:u32)
                n124 = call "ID解析.vi"("ID"=w256) -> ("PDU(1)"=w249:i32)  [unwired: 10 out]
                n125 = case shown="14" w249 {
                  tunnel: w255 -> [w258 w264]
                  tunnel: w254 -> [w257 w263]
                  tunnel: w253 -> [_ w262]
                  tunnel: [w258 w261] -> w252
                  tunnel: [w257 w260] -> w251
                  frame 0, Default {
                  }
                  frame 20 {
                    n126 = local write "状态"(FALSE ("状态")) -> ()
                    n127 = Enqueue Element(queue=w264, element=w262, error in (no error)=w263) -> (queue out=w261:refnum<queue>, error out=w260:errorcluster)  [unwired: 2 out]
                  }
                }
              }
              frame True {
              }
            }
          }
        }
      }
      n128 = while {
        tunnel: w156 -> [w160]
        tunnel: w155 -> [w159]
        stop <- w161 stop-if-true
        n129 = Dequeue Element(queue=w160, error in (no error)=w159) -> (element=w158:T1, error out=w161:errorcluster)  [unwired: 3 out]
        n130 = case shown="无错误" w161 {
          tunnel: w158 -> [w162 _]
          frame No Error {
            n131 = local write "状态"(TRUE ("状态")) -> ()
            "VCI_Receive 2" <- w162
          }
          frame Error {
          }
        }
      }
      n132 = Release Queue(queue=w154, force destroy? (F)=TRUE ("强制销毁？(F)"), error in (no error)=w153) -> (error out=w152:errorcluster)  [unwired: 2 out]
      n133 = call <vilib>:"Clear Errors.vi"("error in (no error)"=w152) -> ()  [unwired: 7 out]
    }
    frame Enabled {
    }
  }
  n134 = while {
    stop <- w267 stop-if-true
    n135 = local read "停止"() -> (w267:bool)
    n136 = local read "选项卡控件"() -> (w269:enum32{"单体电压", "单体温度", "单体内阻", "单体SOC"})
    n137 = Wait Until Next ms Multiple(millisecond multiple=u32 500 ("毫秒倍数")) -> ()  [unwired: 1 out]
    n138 = case shown="\"单体电压\", 默认" w269 {
      frame "单体电压", Default {
        w280 = 0.0 ("新元素/子数组")
        n139 = global read "从板全局变量.vi" "电池节数"() -> (w271:u8[])
        n140 = global read "单体信息全局.vi" "单体数据"() -> (w279:dbl[][])
        n141 = To Unsigned Word Integer(number=w271) -> (unsigned 16bit integer=w270:u16[])
        n142 = global read "从板全局变量.vi" "均衡标记"() -> (w282:dbl[])
        n143 = global read "单体信息全局.vi" "放电均衡"() -> (w341:dbl[])
        n144 = global read "单体信息全局.vi" "均衡故障"() -> (w315:dbl[])
        n145 = global read "单体信息全局.vi" "充电均衡"() -> (w368:dbl[])
        n146 = for {
          tunnel: w271 -> [w411] mode=indexing
          tunnel: w279 -> [w414]
          shift-right: [w409] -> w274
          shift-left: dbl[] [] -> [w410]
          tunnel: w271 -> [w408]
          shift-right: [w406] -> w276
          shift-left: u16[] [] -> [w407]
          i -> [w413]
          n147 = Greater Than 0?(x=w411) -> (x > 0?=w412:bool)
          n148 = case shown="真" w412 {
            tunnel: w414 -> [_ w430]
            tunnel: w413 -> [_ w419]
            tunnel: w411 -> [_ w418]
            tunnel: w410 -> [w416 w427]
            tunnel: [w416 w428] -> w409
            tunnel: w408 -> [_ w425]
            tunnel: w407 -> [w415 w422]
            tunnel: [w415 w421] -> w406
            frame False {
            }
            frame True {
              n149 = Index Array(array=w430, index (row)=w419) -> (element=w429:dbl[])  [unwired: 1 in]
              n150 = Increment(x=w419) -> (x+1=w423:i32)
              n151 = Initialize Array(w423, w418) -> (w417:i32[])
              n152 = Array Subset(array=w429, length=w418) -> (w426:dbl[])  [unwired: 1 in]
              n153 = Array Subset(array=w425, length=w419) -> (w424:u8[])  [unwired: 1 in]
              n154 = Add Array Elements(numeric array=w424) -> (sum=w420:u8)
              n155 = Insert Into Array(array=w427, index=w420, new element=w426) -> (w428:dbl[])
              n156 = Insert Into Array(array=w422, index=w420, new element=w417) -> (w421:u16[])
            }
          }
        }
        n157 = global read "单体信息全局.vi" "位置"() -> (w286:i32[])
        n158 = Insert Into Array(array=w282, index=w280, new element=w280) -> (w281:dbl[])
        n159 = for {
          N: 25 -> [_]
          tunnel: w341 -> [w445]
          tunnel: [w441] -> w340 mode=indexing
          tunnel: w281 -> [w437]
          tunnel: w286 -> [w438]
          i -> [w440]
          w444 = 12 ("y")
          n160 = Multiply(x=w440, y=w444) -> (x*y=w439:i32)
          n161 = Array Subset(array=w445, index=w439, length=w444) -> (w443:dbl[])
          n162 = for {
            tunnel: w443 -> [w454] mode=indexing
            tunnel: [w455] -> w442 mode=indexing
            tunnel: w439 -> [w453]
            tunnel: w438 -> [w451]
            tunnel: w437 -> [w449]
            i -> [w452]
            n163 = Add(x=w453, y=w452) -> (x+y=w450:i32)
            n164 = Equal To 0?(x=w454) -> (x = 0?=w446:bool)
            n165 = Index Array(array=w451, index=w450) -> (element=w448:i32)
            n166 = Index Array(array=w449, index=w448) -> (element=w447:dbl)
            n167 = case shown="假" w446 {
              tunnel: w446 -> [w466 _]
              tunnel: [w465 u32 13816530] -> w455
              tunnel: w447 -> [w456 _]
              frame False {
                n168 = Equal To 0?(x=w456) -> (x = 0?=w464:bool)
                n169 = Equal To 0?(x=w456) -> (x = 0?=w460:bool)
                n170 = Select(t=u32 13816530, s=w464, f=u32 16776770) -> (s? t:f=w461:u32)
                n171 = Select(t=u32 16776770, s=w460, f=u32 6618880) -> (s? t:f=w458:u32)
                n172 = Select(t=w461, s=w466, f=w458) -> (s? t:f=w465:u32)
              }
              frame True {
              }
            }
          }
          n173 = Array To Cluster(array=w442) -> (cluster=w441:T14)
        }
        n174 = for {
          N: 25 -> [_]
          tunnel: w368 -> [w476]
          tunnel: [w472] -> w367 mode=indexing
          tunnel: w281 -> [w468]
          tunnel: w286 -> [w469]
          i -> [w471]
          w475 = 12 ("y")
          n175 = Multiply(x=w471, y=w475) -> (x*y=w470:i32)
          n176 = Array Subset(array=w476, index=w470, length=w475) -> (w474:dbl[])
          n177 = for {
            tunnel: w474 -> [w485] mode=indexing
            tunnel: [w486] -> w473 mode=indexing
            tunnel: w470 -> [w484]
            tunnel: w469 -> [w481]
            tunnel: w468 -> [w478]
            i -> [w483]
            n178 = Add(x=w484, y=w483) -> (x+y=w482:i32)
            n179 = Equal To 0?(x=w485) -> (x = 0?=w477:bool)
            n180 = Index Array(array=w481, index=w482) -> (element=w480:i32)
            n181 = Index Array(array=w478, index=w480) -> (element=w479:dbl)
            n182 = case shown="假" w477 {
              tunnel: w477 -> [w497 _]
              tunnel: [w496 u32 13816530] -> w486
              tunnel: w479 -> [w487 _]
              frame False {
                n183 = Equal To 0?(x=w487) -> (x = 0?=w495:bool)
                n184 = Equal To 0?(x=w487) -> (x = 0?=w492:bool)
                n185 = Select(t=u32 13816530, s=w492, f=u32 16776770) -> (s? t:f=w490:u32)
                n186 = Select(t=u32 16776770, s=w495, f=u32 16860) -> (s? t:f=w494:u32)
                n187 = Select(t=w490, s=w497, f=w494) -> (s? t:f=w496:u32)
              }
              frame True {
              }
            }
          }
          n188 = Array To Cluster(array=w473) -> (cluster=w472:T14)
        }
        n189 = Add Array Elements(numeric array=w270) -> (sum=w275:u16)
        n190 = global write "单体信息全局.vi" "PF"(w275) -> ()
        n191 = Quotient & Remainder(x=w275, y=12) -> (x-y*floor(x/y)=w372:i32, floor(x/y)=w370:i32)
        n192 = for {
          N: 25 -> [_]
          tunnel: w315 -> [w436]
          tunnel: [w432] -> w314 mode=indexing
          i -> [w435]
          w433 = 12 ("y")
          n193 = Multiply(x=w435, y=w433) -> (x*y=w434:i32)
          n194 = Array Subset(array=w436, index=w434, length=w433) -> (w431:dbl[])
          n195 = Array To Cluster(array=w431) -> (cluster=w432:T15)
        }
        n196 = Insert Into Array(array=w274, new element=dbl[] [0.0, 0.0, 0.0, 0.0, 0.0, 0.0, 0.0, 0.0, 8.0]) -> (w272:dbl[])  [unwired: 1 in]
        n197 = Equal To 0?(x=w372) -> (x = 0?=w371:bool)
        n198 = Increment(x=w370) -> (x+1=w369:i32)
        n199 = global write "单体信息全局.vi" "数据"(w272) -> ()
        n200 = Select(t=w370, s=w371, f=w369) -> (s? t:f=w285:i32)
        n201 = for {
          N: w285 -> [_]
          tunnel: w272 -> [w507]
          tunnel: w276 -> [w499]
          tunnel: [w500] -> w404 mode=indexing
          i -> [w506]
          w504 = 12 ("y")
          n202 = Multiply(x=w506, y=w504) -> (x*y=w505:i32)
          n203 = Array Subset(array=w499, index=w505, length=w504) -> (w502:u16[])
          n204 = Array Subset(array=w507, index=w505, length=w504) -> (w503:dbl[])
          n205 = Insert Into Array(array=w503, new element=w502) -> (w501:dbl[])  [unwired: 1 in]
          n206 = Array To Cluster(array=w501) -> (cluster=w500:T16)
        }
        n207 = Index Array(array=w314) -> (element #1=w313:T15, element #2=w312:T15, element #3=w311:T15, element #4=w310:T15, element #5=w309:T15, element #6=w308:T15, element #7=w307:T15, element #8=w306:T15, element #9=w305:T15, element #10=w304:T15, element #11=w303:T15, element #12=w302:T15, element #13=w301:T15, element #14=w300:T15, element #15=w299:T15, element #16=w298:T15, element #17=w297:T15, element #18=w296:T15, element #19=w295:T15, element #20=w294:T15, element #21=w293:T15, element #22=w292:T15, element #23=w291:T15, element #24=w290:T15, element #25=w289:T15)  [unwired: 25 in]
        n208 = Index Array(array=w340) -> (element #1=w339:T14, element #2=w338:T14, element #3=w337:T14, element #4=w336:T14, element #5=w335:T14, element #6=w334:T14, element #7=w333:T14, element #8=w332:T14, element #9=w331:T14, element #10=w330:T14, element #11=w329:T14, element #12=w328:T14, element #13=w327:T14, element #14=w326:T14, element #15=w325:T14, element #16=w324:T14, element #17=w323:T14, element #18=w322:T14, element #19=w321:T14, element #20=w320:T14, element #21=w319:T14, element #22=w318:T14, element #23=w317:T14, element #24=w316:T14, element #25=w288:T14)  [unwired: 25 in]
        n209 = local write "1 13"(w289) -> ()
        n210 = Index Array(array=w367) -> (element #1=w366:T14, element #2=w365:T14, element #3=w364:T14, element #4=w363:T14, element #5=w362:T14, element #6=w361:T14, element #7=w360:T14, element #8=w359:T14, element #9=w358:T14, element #10=w357:T14, element #11=w356:T14, element #12=w355:T14, element #13=w354:T14, element #14=w353:T14, element #15=w352:T14, element #16=w351:T14, element #17=w350:T14, element #18=w349:T14, element #19=w348:T14, element #20=w347:T14, element #21=w346:T14, element #22=w345:T14, element #23=w344:T14, element #24=w343:T14, element #25=w342:T14)  [unwired: 25 in]
        n211 = local write "放电均衡"(w288) -> ()
        n212 = local write "充电均衡"(w342) -> ()
        n213 = Index Array(array=w404) -> (element #1=w403:T16, element #2=w402:T16, element #3=w401:T16, element #4=w400:T16, element #5=w399:T16, element #6=w398:T16, element #7=w397:T16, element #8=w396:T16, element #9=w392:T16, element #10=w391:T16, element #11=w390:T16, element #12=w389:T16, element #13=w388:T16, element #14=w387:T16, element #15=w386:T16, element #16=w385:T16, element #17=w382:T16, element #18=w381:T16, element #19=w380:T16, element #20=w379:T16, element #21=w378:T16, element #22=w377:T16, element #23=w376:T16, element #24=w375:T16, element #25=w374:T16)  [unwired: 25 in]
        n214 = local read "1"() -> (w405:T4)
        n215 = local write "1 5"(w374) -> ()
        n216 = Bundle(cluster=w405, "1 102"=w403, "1 3"=w402, "1 4"=w401, "1 6"=w400, "1 7"=w399, "1 8"=w398, "1 9"=w397, "1 10"=w396, "1 12"=w366, "1 28"=w365, "1 25"=w364, "1 31"=w363, "1 16"=w362, "1 19"=w361, "1 22"=w360, "1 34"=w359, "1 11"=w339, "1 27"=w338, "1 24"=w337, "1 30"=w336, "1 15"=w335, "1 18"=w334, "1 21"=w333, "1 33"=w332, "1 13"=w313, "1 26"=w312, "1 23"=w311, "1 29"=w310, "1 14"=w309, "1 17"=w308, "1 20"=w307, "1 32"=w306) -> (w395:T4)
        n217 = local read "2"() -> (w394:T5)
        n218 = Bundle(cluster=w394, "1 26"=w392, "1 27"=w391, "1 28"=w390, "1 29"=w389, "1 30"=w388, "1 31"=w387, "1 32"=w386, "1 33"=w385, "1 16"=w358, "1 44"=w357, "1 36"=w356, "1 47"=w355, "1 19"=w354, "1 38"=w353, "1 41"=w352, "1 50"=w351, "1 15"=w331, "1 43"=w330, "1 35"=w329, "1 46"=w328, "1 18"=w327, "1 37"=w326, "1 40"=w325, "1 49"=w324, "1 14"=w305, "1 42"=w304, "1 34"=w303, "1 45"=w302, "1 17"=w301, "1 20"=w300, "1 39"=w299, "1 48"=w298) -> (w393:T5)
        n219 = local write "1"(w395) -> ()
        n220 = local write "2"(w393) -> ()
        n221 = local read "3"() -> (w383:T6)
        n222 = Bundle(cluster=w383, "1 18"=w382, "1 19"=w381, "1 20"=w380, "1 21"=w379, "1 22"=w378, "1 23"=w377, "1 24"=w376, "1 25"=w375, "1 12"=w350, "1 39"=w349, "1 28"=w348, "1 42"=w347, "1 16"=w346, "1 30"=w345, "1 33"=w344, "1 36"=w343, "1 11"=w323, "1 38"=w322, "1 27"=w321, "1 41"=w320, "1 15"=w319, "1 29"=w318, "1 32"=w317, "1 35"=w316, "1 13"=w297, "1 37"=w296, "1 26"=w295, "1 40"=w294, "1 14"=w293, "1 17"=w292, "1 31"=w291, "1 34"=w290) -> (w384:T6)
        n223 = local write "3"(w384) -> ()
      }
      frame "单体温度" {
        (unwired) 12 ("y")
        n224 = global read "从板全局变量.vi" "温度个数"() -> (w515:u8[])
        n225 = global read "单体信息全局.vi" "温度数据"() -> (w513:sgl[][])
        n226 = Add Array Elements(numeric array=w515) -> (sum=w512:u8)
        n227 = Wait Until Next ms Multiple(millisecond multiple=u32 500 ("毫秒倍数")) -> ()  [unwired: 1 out]
        n228 = for {
          tunnel: w515 -> [w561] mode=indexing
          tunnel: w513 -> [w564]
          shift-right: [w559] -> w510
          shift-left: dbl[] [] -> [w560]
          tunnel: w515 -> [w558]
          shift-right: [w556] -> w511
          shift-left: u16[] [] -> [w557]
          i -> [w563]
          n229 = Greater Than 0?(x=w561) -> (x > 0?=w562:bool)
          n230 = case shown="真" w562 {
            tunnel: w564 -> [_ w580]
            tunnel: w563 -> [_ w569]
            tunnel: w561 -> [_ w568]
            tunnel: w560 -> [w566 w577]
            tunnel: [w566 w578] -> w559
            tunnel: w558 -> [_ w575]
            tunnel: w557 -> [w565 w572]
            tunnel: [w565 w571] -> w556
            frame False {
            }
            frame True {
              n231 = Index Array(array=w580, index (row)=w569) -> (element=w579:sgl[])  [unwired: 1 in]
              n232 = Increment(x=w569) -> (x+1=w573:i32)
              n233 = Initialize Array(w573, w568) -> (w567:i32[])
              n234 = Array Subset(array=w579, length=w568) -> (w576:sgl[])  [unwired: 1 in]
              n235 = Array Subset(array=w575, length=w569) -> (w574:u8[])  [unwired: 1 in]
              n236 = Add Array Elements(numeric array=w574) -> (sum=w570:u8)
              n237 = Insert Into Array(array=w577, index=w570, new element=w576) -> (w578:dbl[])
              n238 = Insert Into Array(array=w572, index=w570, new element=w567) -> (w571:u16[])
            }
          }
        }
        n239 = Quotient & Remainder(x=w512, y=12) -> (x-y*floor(x/y)=w522:i32, floor(x/y)=w520:i32)
        n240 = Equal To 0?(x=w522) -> (x = 0?=w521:bool)
        n241 = Increment(x=w520) -> (x+1=w519:i32)
        n242 = Select(t=w520, s=w521, f=w519) -> (s? t:f=w518:i32)
        n243 = Insert Into Array(array=w510, new element=dbl[] [0.0, 0.0, 0.0, 0.0, 0.0, 0.0, 0.0, 0.0, 0.0]) -> (w508:dbl[])  [unwired: 1 in]
        n244 = for {
          N: w518 -> [w584]
          tunnel: w508 -> [w592]
          tunnel: w511 -> [w585]
          tunnel: [w586] -> w554 mode=indexing
          i -> [w583]
          w590 = 12 ("y")
          n245 = Increment(x=w583) -> (x+1=w582:i32)
          n246 = Equal?(x=w584, y=w582) -> ()  [unwired: 1 out]
          n247 = Multiply(x=w583, y=w590) -> (x*y=w591:i32)
          n248 = Array Subset(array=w585, index=w591, length=w590) -> (w588:u16[])
          n249 = Array Subset(array=w592, index=w591, length=w590) -> (w589:dbl[])
          n250 = Insert Into Array(array=w589, index=12 ("索引"), new element=w588) -> (w587:dbl[])
          n251 = Array To Cluster(array=w587) -> (cluster=w586:T16)
        }
        n252 = global write "单体信息全局.vi" "数据 2"(w508) -> ()
        n253 = Index Array(array=w554) -> (element #1=w553:T16, element #2=w552:T16, element #3=w551:T16, element #4=w550:T16, element #5=w549:T16, element #6=w548:T16, element #7=w547:T16, element #8=w546:T16, element #9=w542:T16, element #10=w541:T16, element #11=w540:T16, element #12=w539:T16, element #13=w538:T16, element #14=w537:T16, element #15=w536:T16, element #16=w535:T16, element #17=w532:T16, element #18=w531:T16, element #19=w530:T16, element #20=w529:T16, element #21=w528:T16, element #22=w527:T16, element #23=w526:T16, element #24=w525:T16, element #25=w524:T16)  [unwired: 25 in]
        n254 = local read "6"() -> (w533:T12)
        n255 = local read "5"() -> (w544:T11)
        n256 = Bundle(cluster=w544, "1 26"=w542, "1 27"=w541, "1 28"=w540, "1 29"=w539, "1 30"=w538, "1 31"=w537, "1 32"=w536, "1 33"=w535) -> (w543:T11)
        n257 = Bundle(cluster=w533, "1 18"=w532, "1 19"=w531, "1 20"=w530, "1 21"=w529, "1 22"=w528, "1 23"=w527, "1 24"=w526, "1 25"=w525) -> (w534:T12)
        n258 = local write "1 6"(w524) -> ()
        n259 = local write "5"(w543) -> ()
        n260 = local read "4"() -> (w555:T10)
        n261 = local write "6"(w534) -> ()
        n262 = Bundle(cluster=w555, "1 102"=w553, "1 3"=w552, "1 4"=w551, "1 6"=w550, "1 7"=w549, "1 8"=w548, "1 9"=w547, "1 10"=w546) -> (w545:T10)
        n263 = local write "4"(w545) -> ()
      }
    }
    n264 = disable-structure shown="禁用" {
      frame Disabled {
        n265 = global read "单体信息全局.vi" "PF"() -> ()  [unwired: 1 out]
        n266 = global read "单体信息全局.vi" "数据"() -> ()  [unwired: 1 out]
      }
      frame Enabled {
      }
    }
  }
  n267 = disable-structure shown="启用" {
    frame Enabled {
      n268 = while {
        stop <- w597 stop-if-true
        n269 = local read "选项卡控件"() -> (w596:enum32{"单体电压", "单体温度", "单体内阻", "单体SOC"})
        n270 = local read "停止"() -> (w597:bool)
        n271 = Wait Until Next ms Multiple(millisecond multiple=u32 500 ("毫秒倍数")) -> ()  [unwired: 1 out]
        n272 = Or(x="布尔", y="布尔 2") -> (x .or. y?=w595:bool)
        n273 = case shown="真" w595 {
          tunnel: w596 -> [w599 w866]
          frame False {
            n274 = case shown="真" "一次置位" {
              tunnel: w599 -> [_ w601]
              frame False {
              }
              frame True {
                n275 = case shown="\"单体温度\"" w601 {
                  frame "单体电压", Default {
                    n276 = for {
                      N: 9 -> [_]
                      i -> [w687]
                      n277 = case shown="0" w687 {
                        tunnel: bool[] [FALSE, FALSE, FALSE, FALSE, FALSE, FALSE, FALSE, FALSE, FALSE, FALSE, FALSE, FALSE, FALSE] -> [w690 w695 w700 w705 w710 w715 w720 w725 w730 _]
                        frame 0 {
                          n278 = control-ref of="1 18"() -> (w689:refnum<vi>)
                          n279 = property class="Clust (严格)"(reference=w689) -> ("Controls[]"=w691:refnum<vi>[])  [unwired: 1 in, 2 out]
                          n280 = for {
                            tunnel: w691 -> [w692] mode=indexing
                            tunnel: w690 -> [w693] mode=indexing
                            n281 = property class="Ctl"(reference=w692, "Blinking"=w693) -> ()  [unwired: 1 in, 2 out]
                          }
                        }
                        frame 1 {
                          n282 = control-ref of="1 19"() -> (w694:refnum<vi>)
                          n283 = property class="Clust (严格)"(reference=w694) -> ("Controls[]"=w696:refnum<vi>[])  [unwired: 1 in, 2 out]
                          n284 = for {
                            tunnel: w696 -> [w697] mode=indexing
                            tunnel: w695 -> [w698] mode=indexing
                            n285 = property class="Ctl"(reference=w697, "Blinking"=w698) -> ()  [unwired: 1 in, 2 out]
                          }
                        }
                        frame 2 {
                          n286 = control-ref of="1 20"() -> (w699:refnum<vi>)
                          n287 = property class="Clust (严格)"(reference=w699) -> ("Controls[]"=w701:refnum<vi>[])  [unwired: 1 in, 2 out]
                          n288 = for {
                            tunnel: w701 -> [w702] mode=indexing
                            tunnel: w700 -> [w703] mode=indexing
                            n289 = property class="Ctl"(reference=w702, "Blinking"=w703) -> ()  [unwired: 1 in, 2 out]
                          }
                        }
                        frame 3 {
                          n290 = control-ref of="1 21"() -> (w704:refnum<vi>)
                          n291 = property class="Clust (严格)"(reference=w704) -> ("Controls[]"=w706:refnum<vi>[])  [unwired: 1 in, 2 out]
                          n292 = for {
                            tunnel: w706 -> [w707] mode=indexing
                            tunnel: w705 -> [w708] mode=indexing
                            n293 = property class="Ctl"(reference=w707, "Blinking"=w708) -> ()  [unwired: 1 in, 2 out]
                          }
                        }
                        frame 4 {
                          n294 = control-ref of="1 22"() -> (w709:refnum<vi>)
                          n295 = property class="Clust (严格)"(reference=w709) -> ("Controls[]"=w711:refnum<vi>[])  [unwired: 1 in, 2 out]
                          n296 = for {
                            tunnel: w711 -> [w712] mode=indexing
                            tunnel: w710 -> [w713] mode=indexing
                            n297 = property class="Ctl"(reference=w712, "Blinking"=w713) -> ()  [unwired: 1 in, 2 out]
                          }
                        }
                        frame 5 {
                          n298 = control-ref of="1 23"() -> (w714:refnum<vi>)
                          n299 = property class="Clust (严格)"(reference=w714) -> ("Controls[]"=w716:refnum<vi>[])  [unwired: 1 in, 2 out]
                          n300 = for {
                            tunnel: w716 -> [w717] mode=indexing
                            tunnel: w715 -> [w718] mode=indexing
                            n301 = property class="Ctl"(reference=w717, "Blinking"=w718) -> ()  [unwired: 1 in, 2 out]
                          }
                        }
                        frame 6 {
                          n302 = control-ref of="1 24"() -> (w719:refnum<vi>)
                          n303 = property class="Clust (严格)"(reference=w719) -> ("Controls[]"=w721:refnum<vi>[])  [unwired: 1 in, 2 out]
                          n304 = for {
                            tunnel: w721 -> [w722] mode=indexing
                            tunnel: w720 -> [w723] mode=indexing
                            n305 = property class="Ctl"(reference=w722, "Blinking"=w723) -> ()  [unwired: 1 in, 2 out]
                          }
                        }
                        frame 7 {
                          n306 = control-ref of="1 25"() -> (w724:refnum<vi>)
                          n307 = property class="Clust (严格)"(reference=w724) -> ("Controls[]"=w726:refnum<vi>[])  [unwired: 1 in, 2 out]
                          n308 = for {
                            tunnel: w726 -> [w727] mode=indexing
                            tunnel: w725 -> [w728] mode=indexing
                            n309 = property class="Ctl"(reference=w727, "Blinking"=w728) -> ()  [unwired: 1 in, 2 out]
                          }
                        }
                        frame 8 {
                          n310 = control-ref of="1 5"() -> (w729:refnum<vi>)
                          n311 = property class="Clust (严格)"(reference=w729) -> ("Controls[]"=w731:refnum<vi>[])  [unwired: 1 in, 2 out]
                          n312 = for {
                            tunnel: w731 -> [w732] mode=indexing
                            tunnel: w730 -> [w733] mode=indexing
                            n313 = property class="Ctl"(reference=w732, "Blinking"=w733) -> ()  [unwired: 1 in, 2 out]
                          }
                        }
                        frame 99, Default {
                        }
                      }
                    }
                    n314 = for {
                      N: 16 -> [_]
                      i -> [w606]
                      n315 = case shown="6" w606 {
                        tunnel: bool[] [FALSE, FALSE, FALSE, FALSE, FALSE, FALSE, FALSE, FALSE, FALSE, FALSE, FALSE, FALSE, FALSE] -> [w607 w613 w618 w623 w628 w633 w638 w643 w648 w653 w658 w663 w668 w673 w678 w683 _]
                        frame 0 {
                          n316 = control-ref of="1 102"() -> (w609:refnum<vi>)
                          n317 = property class="Clust (严格)"(reference=w609) -> ("Controls[]"=w608:refnum<vi>[])  [unwired: 1 in, 2 out]
                          n318 = for {
                            tunnel: w608 -> [w610] mode=indexing
                            tunnel: w607 -> [w611] mode=indexing
                            n319 = property class="Ctl"(reference=w610, "Blinking"=w611) -> ()  [unwired: 1 in, 2 out]
                          }
                        }
                        frame 1 {
                          n320 = control-ref of="1 3"() -> (w612:refnum<vi>)
                          n321 = property class="Clust (严格)"(reference=w612) -> ("Controls[]"=w614:refnum<vi>[])  [unwired: 1 in, 2 out]
                          n322 = for {
                            tunnel: w614 -> [w615] mode=indexing
                            tunnel: w613 -> [w616] mode=indexing
                            n323 = property class="Ctl"(reference=w615, "Blinking"=w616) -> ()  [unwired: 1 in, 2 out]
                          }
                        }
                        frame 2 {
                          n324 = control-ref of="1 4"() -> (w617:refnum<vi>)
                          n325 = property class="Clust (严格)"(reference=w617) -> ("Controls[]"=w619:refnum<vi>[])  [unwired: 1 in, 2 out]
                          n326 = for {
                            tunnel: w619 -> [w620] mode=indexing
                            tunnel: w618 -> [w621] mode=indexing
                            n327 = property class="Ctl"(reference=w620, "Blinking"=w621) -> ()  [unwired: 1 in, 2 out]
                          }
                        }
                        frame 3 {
                          n328 = control-ref of="1 6"() -> (w622:refnum<vi>)
                          n329 = property class="Clust (严格)"(reference=w622) -> ("Controls[]"=w624:refnum<vi>[])  [unwired: 1 in, 2 out]
                          n330 = for {
                            tunnel: w624 -> [w625] mode=indexing
                            tunnel: w623 -> [w626] mode=indexing
                            n331 = property class="Ctl"(reference=w625, "Blinking"=w626) -> ()  [unwired: 1 in, 2 out]
                          }
                        }
                        frame 4 {
                          n332 = control-ref of="1 7"() -> (w627:refnum<vi>)
                          n333 = property class="Clust (严格)"(reference=w627) -> ("Controls[]"=w629:refnum<vi>[])  [unwired: 1 in, 2 out]
                          n334 = for {
                            tunnel: w629 -> [w630] mode=indexing
                            tunnel: w628 -> [w631] mode=indexing
                            n335 = property class="Ctl"(reference=w630, "Blinking"=w631) -> ()  [unwired: 1 in, 2 out]
                          }
                        }
                        frame 5 {
                          n336 = control-ref of="1 8"() -> (w632:refnum<vi>)
                          n337 = property class="Clust (严格)"(reference=w632) -> ("Controls[]"=w634:refnum<vi>[])  [unwired: 1 in, 2 out]
                          n338 = for {
                            tunnel: w634 -> [w635] mode=indexing
                            tunnel: w633 -> [w636] mode=indexing
                            n339 = property class="Ctl"(reference=w635, "Blinking"=w636) -> ()  [unwired: 1 in, 2 out]
                          }
                        }
                        frame 6 {
                          n340 = control-ref of="1 9"() -> (w637:refnum<vi>)
                          n341 = property class="Clust (严格)"(reference=w637) -> ("Controls[]"=w639:refnum<vi>[])  [unwired: 1 in, 2 out]
                          n342 = for {
                            tunnel: w639 -> [w640] mode=indexing
                            tunnel: w638 -> [w641] mode=indexing
                            n343 = property class="Ctl"(reference=w640, "Blinking"=w641) -> ()  [unwired: 1 in, 2 out]
                          }
                        }
                        frame 7 {
                          n344 = control-ref of="1 10"() -> (w642:refnum<vi>)
                          n345 = property class="Clust (严格)"(reference=w642) -> ("Controls[]"=w644:refnum<vi>[])  [unwired: 1 in, 2 out]
                          n346 = for {
                            tunnel: w644 -> [w645] mode=indexing
                            tunnel: w643 -> [w646] mode=indexing
                            n347 = property class="Ctl"(reference=w645, "Blinking"=w646) -> ()  [unwired: 1 in, 2 out]
                          }
                        }
                        frame 8 {
                          n348 = control-ref of="1 26"() -> (w647:refnum<vi>)
                          n349 = property class="Clust (严格)"(reference=w647) -> ("Controls[]"=w649:refnum<vi>[])  [unwired: 1 in, 2 out]
                          n350 = for {
                            tunnel: w649 -> [w650] mode=indexing
                            tunnel: w648 -> [w651] mode=indexing
                            n351 = property class="Ctl"(reference=w650, "Blinking"=w651) -> ()  [unwired: 1 in, 2 out]
                          }
                        }
                        frame 9 {
                          n352 = control-ref of="1 27"() -> (w652:refnum<vi>)
                          n353 = property class="Clust (严格)"(reference=w652) -> ("Controls[]"=w654:refnum<vi>[])  [unwired: 1 in, 2 out]
                          n354 = for {
                            tunnel: w654 -> [w655] mode=indexing
                            tunnel: w653 -> [w656] mode=indexing
                            n355 = property class="Ctl"(reference=w655, "Blinking"=w656) -> ()  [unwired: 1 in, 2 out]
                          }
                        }
                        frame 10 {
                          n356 = control-ref of="1 28"() -> (w657:refnum<vi>)
                          n357 = property class="Clust (严格)"(reference=w657) -> ("Controls[]"=w659:refnum<vi>[])  [unwired: 1 in, 2 out]
                          n358 = for {
                            tunnel: w659 -> [w660] mode=indexing
                            tunnel: w658 -> [w661] mode=indexing
                            n359 = property class="Ctl"(reference=w660, "Blinking"=w661) -> ()  [unwired: 1 in, 2 out]
                          }
                        }
                        frame 11 {
                          n360 = control-ref of="1 29"() -> (w662:refnum<vi>)
                          n361 = property class="Clust (严格)"(reference=w662) -> ("Controls[]"=w664:refnum<vi>[])  [unwired: 1 in, 2 out]
                          n362 = for {
                            tunnel: w664 -> [w665] mode=indexing
                            tunnel: w663 -> [w666] mode=indexing
                            n363 = property class="Ctl"(reference=w665, "Blinking"=w666) -> ()  [unwired: 1 in, 2 out]
                          }
                        }
                        frame 12 {
                          n364 = control-ref of="1 30"() -> (w667:refnum<vi>)
                          n365 = property class="Clust (严格)"(reference=w667) -> ("Controls[]"=w669:refnum<vi>[])  [unwired: 1 in, 2 out]
                          n366 = for {
                            tunnel: w669 -> [w670] mode=indexing
                            tunnel: w668 -> [w671] mode=indexing
                            n367 = property class="Ctl"(reference=w670, "Blinking"=w671) -> ()  [unwired: 1 in, 2 out]
                          }
                        }
                        frame 13 {
                          n368 = control-ref of="1 31"() -> (w672:refnum<vi>)
                          n369 = property class="Clust (严格)"(reference=w672) -> ("Controls[]"=w674:refnum<vi>[])  [unwired: 1 in, 2 out]
                          n370 = for {
                            tunnel: w674 -> [w675] mode=indexing
                            tunnel: w673 -> [w676] mode=indexing
                            n371 = property class="Ctl"(reference=w675, "Blinking"=w676) -> ()  [unwired: 1 in, 2 out]
                          }
                        }
                        frame 14 {
                          n372 = control-ref of="1 32"() -> (w677:refnum<vi>)
                          n373 = property class="Clust (严格)"(reference=w677) -> ("Controls[]"=w679:refnum<vi>[])  [unwired: 1 in, 2 out]
                          n374 = for {
                            tunnel: w679 -> [w680] mode=indexing
                            tunnel: w678 -> [w681] mode=indexing
                            n375 = property class="Ctl"(reference=w680, "Blinking"=w681) -> ()  [unwired: 1 in, 2 out]
                          }
                        }
                        frame 15 {
                          n376 = control-ref of="1 33"() -> (w682:refnum<vi>)
                          n377 = property class="Clust (严格)"(reference=w682) -> ("Controls[]"=w684:refnum<vi>[])  [unwired: 1 in, 2 out]
                          n378 = for {
                            tunnel: w684 -> [w685] mode=indexing
                            tunnel: w683 -> [w686] mode=indexing
                            n379 = property class="Ctl"(reference=w685, "Blinking"=w686) -> ()  [unwired: 1 in, 2 out]
                          }
                        }
                        frame 99, Default {
                        }
                      }
                    }
                  }
                  frame "单体温度" {
                    n380 = for {
                      N: 16 -> [_]
                      i -> [w737]
                      n381 = case shown="4" w737 {
                        tunnel: bool[] [FALSE, FALSE, FALSE, FALSE, FALSE, FALSE, FALSE, FALSE, FALSE, FALSE, FALSE, FALSE, FALSE] -> [w739 w744 w749 w754 w759 w764 w769 w774 w779 w784 w789 w794 w799 w804 w809 w814 _]
                        frame 0 {
                          n382 = control-ref of="1 102"() -> (w738:refnum<vi>)
                          n383 = property class="Clust (严格)"(reference=w738) -> ("Controls[]"=w740:refnum<vi>[])  [unwired: 1 in, 2 out]
                          n384 = for {
                            tunnel: w740 -> [w741] mode=indexing
                            tunnel: w739 -> [w742] mode=indexing
                            n385 = property class="Ctl"(reference=w741, "Blinking"=w742) -> ()  [unwired: 1 in, 2 out]
                          }
                        }
                        frame 1 {
                          n386 = control-ref of="1 3"() -> (w743:refnum<vi>)
                          n387 = property class="Clust (严格)"(reference=w743) -> ("Controls[]"=w745:refnum<vi>[])  [unwired: 1 in, 2 out]
                          n388 = for {
                            tunnel: w745 -> [w746] mode=indexing
                            tunnel: w744 -> [w747] mode=indexing
                            n389 = property class="Ctl"(reference=w746, "Blinking"=w747) -> ()  [unwired: 1 in, 2 out]
                          }
                        }
                        frame 2 {
                          n390 = control-ref of="1 4"() -> (w748:refnum<vi>)
                          n391 = property class="Clust (严格)"(reference=w748) -> ("Controls[]"=w750:refnum<vi>[])  [unwired: 1 in, 2 out]
                          n392 = for {
                            tunnel: w750 -> [w751] mode=indexing
                            tunnel: w749 -> [w752] mode=indexing
                            n393 = property class="Ctl"(reference=w751, "Blinking"=w752) -> ()  [unwired: 1 in, 2 out]
                          }
                        }
                        frame 3 {
                          n394 = control-ref of="1 6"() -> (w753:refnum<vi>)
                          n395 = property class="Clust (严格)"(reference=w753) -> ("Controls[]"=w755:refnum<vi>[])  [unwired: 1 in, 2 out]
                          n396 = for {
                            tunnel: w755 -> [w756] mode=indexing
                            tunnel: w754 -> [w757] mode=indexing
                            n397 = property class="Ctl"(reference=w756, "Blinking"=w757) -> ()  [unwired: 1 in, 2 out]
                          }
                        }
                        frame 4 {
                          n398 = control-ref of="1 7"() -> (w758:refnum<vi>)
                          n399 = property class="Clust (严格)"(reference=w758) -> ("Controls[]"=w760:refnum<vi>[])  [unwired: 1 in, 2 out]
                          n400 = for {
                            tunnel: w760 -> [w761] mode=indexing
                            tunnel: w759 -> [w762] mode=indexing
                            n401 = property class="Ctl"(reference=w761, "Blinking"=w762) -> ()  [unwired: 1 in, 2 out]
                          }
                        }
                        frame 5 {
                          n402 = control-ref of="1 8"() -> (w763:refnum<vi>)
                          n403 = property class="Clust (严格)"(reference=w763) -> ("Controls[]"=w765:refnum<vi>[])  [unwired: 1 in, 2 out]
                          n404 = for {
                            tunnel: w765 -> [w766] mode=indexing
                            tunnel: w764 -> [w767] mode=indexing
                            n405 = property class="Ctl"(reference=w766, "Blinking"=w767) -> ()  [unwired: 1 in, 2 out]
                          }
                        }
                        frame 6 {
                          n406 = control-ref of="1 9"() -> (w768:refnum<vi>)
                          n407 = property class="Clust (严格)"(reference=w768) -> ("Controls[]"=w770:refnum<vi>[])  [unwired: 1 in, 2 out]
                          n408 = for {
                            tunnel: w770 -> [w771] mode=indexing
                            tunnel: w769 -> [w772] mode=indexing
                            n409 = property class="Ctl"(reference=w771, "Blinking"=w772) -> ()  [unwired: 1 in, 2 out]
                          }
                        }
                        frame 7 {
                          n410 = control-ref of="1 10"() -> (w773:refnum<vi>)
                          n411 = property class="Clust (严格)"(reference=w773) -> ("Controls[]"=w775:refnum<vi>[])  [unwired: 1 in, 2 out]
                          n412 = for {
                            tunnel: w775 -> [w776] mode=indexing
                            tunnel: w774 -> [w777] mode=indexing
                            n413 = property class="Ctl"(reference=w776, "Blinking"=w777) -> ()  [unwired: 1 in, 2 out]
                          }
                        }
                        frame 8 {
                          n414 = control-ref of="1 26"() -> (w778:refnum<vi>)
                          n415 = property class="Clust (严格)"(reference=w778) -> ("Controls[]"=w780:refnum<vi>[])  [unwired: 1 in, 2 out]
                          n416 = for {
                            tunnel: w780 -> [w781] mode=indexing
                            tunnel: w779 -> [w782] mode=indexing
                            n417 = property class="Ctl"(reference=w781, "Blinking"=w782) -> ()  [unwired: 1 in, 2 out]
                          }
                        }
                        frame 9 {
                          n418 = control-ref of="1 27"() -> (w783:refnum<vi>)
                          n419 = property class="Clust (严格)"(reference=w783) -> ("Controls[]"=w785:refnum<vi>[])  [unwired: 1 in, 2 out]
                          n420 = for {
                            tunnel: w785 -> [w786] mode=indexing
                            tunnel: w784 -> [w787] mode=indexing
                            n421 = property class="Ctl"(reference=w786, "Blinking"=w787) -> ()  [unwired: 1 in, 2 out]
                          }
                        }
                        frame 10 {
                          n422 = control-ref of="1 28"() -> (w788:refnum<vi>)
                          n423 = property class="Clust (严格)"(reference=w788) -> ("Controls[]"=w790:refnum<vi>[])  [unwired: 1 in, 2 out]
                          n424 = for {
                            tunnel: w790 -> [w791] mode=indexing
                            tunnel: w789 -> [w792] mode=indexing
                            n425 = property class="Ctl"(reference=w791, "Blinking"=w792) -> ()  [unwired: 1 in, 2 out]
                          }
                        }
                        frame 11 {
                          n426 = control-ref of="1 29"() -> (w793:refnum<vi>)
                          n427 = property class="Clust (严格)"(reference=w793) -> ("Controls[]"=w795:refnum<vi>[])  [unwired: 1 in, 2 out]
                          n428 = for {
                            tunnel: w795 -> [w796] mode=indexing
                            tunnel: w794 -> [w797] mode=indexing
                            n429 = property class="Ctl"(reference=w796, "Blinking"=w797) -> ()  [unwired: 1 in, 2 out]
                          }
                        }
                        frame 12 {
                          n430 = control-ref of="1 30"() -> (w798:refnum<vi>)
                          n431 = property class="Clust (严格)"(reference=w798) -> ("Controls[]"=w800:refnum<vi>[])  [unwired: 1 in, 2 out]
                          n432 = for {
                            tunnel: w800 -> [w801] mode=indexing
                            tunnel: w799 -> [w802] mode=indexing
                            n433 = property class="Ctl"(reference=w801, "Blinking"=w802) -> ()  [unwired: 1 in, 2 out]
                          }
                        }
                        frame 13 {
                          n434 = control-ref of="1 31"() -> (w803:refnum<vi>)
                          n435 = property class="Clust (严格)"(reference=w803) -> ("Controls[]"=w805:refnum<vi>[])  [unwired: 1 in, 2 out]
                          n436 = for {
                            tunnel: w805 -> [w806] mode=indexing
                            tunnel: w804 -> [w807] mode=indexing
                            n437 = property class="Ctl"(reference=w806, "Blinking"=w807) -> ()  [unwired: 1 in, 2 out]
                          }
                        }
                        frame 14 {
                          n438 = control-ref of="1 32"() -> (w808:refnum<vi>)
                          n439 = property class="Clust (严格)"(reference=w808) -> ("Controls[]"=w810:refnum<vi>[])  [unwired: 1 in, 2 out]
                          n440 = for {
                            tunnel: w810 -> [w811] mode=indexing
                            tunnel: w809 -> [w812] mode=indexing
                            n441 = property class="Ctl"(reference=w811, "Blinking"=w812) -> ()  [unwired: 1 in, 2 out]
                          }
                        }
                        frame 15 {
                          n442 = control-ref of="1 33"() -> (w813:refnum<vi>)
                          n443 = property class="Clust (严格)"(reference=w813) -> ("Controls[]"=w815:refnum<vi>[])  [unwired: 1 in, 2 out]
                          n444 = for {
                            tunnel: w815 -> [w816] mode=indexing
                            tunnel: w814 -> [w817] mode=indexing
                            n445 = property class="Ctl"(reference=w816, "Blinking"=w817) -> ()  [unwired: 1 in, 2 out]
                          }
                        }
                        frame 99, Default {
                        }
                      }
                    }
                    n446 = for {
                      N: 9 -> [_]
                      i -> [w819]
                      n447 = case shown="8" w819 {
                        tunnel: bool[] [FALSE, FALSE, FALSE, FALSE, FALSE, FALSE, FALSE, FALSE, FALSE, FALSE, FALSE, FALSE, FALSE] -> [w821 w826 w831 w836 w841 w846 w851 w856 w861 _]
                        frame 0 {
                          n448 = control-ref of="1 18"() -> (w820:refnum<vi>)
                          n449 = property class="Clust (严格)"(reference=w820) -> ("Controls[]"=w822:refnum<vi>[])  [unwired: 1 in, 2 out]
                          n450 = for {
                            tunnel: w822 -> [w823] mode=indexing
                            tunnel: w821 -> [w824] mode=indexing
                            n451 = property class="Ctl"(reference=w823, "Blinking"=w824) -> ()  [unwired: 1 in, 2 out]
                          }
                        }
                        frame 1 {
                          n452 = control-ref of="1 19"() -> (w825:refnum<vi>)
                          n453 = property class="Clust (严格)"(reference=w825) -> ("Controls[]"=w827:refnum<vi>[])  [unwired: 1 in, 2 out]
                          n454 = for {
                            tunnel: w827 -> [w828] mode=indexing
                            tunnel: w826 -> [w829] mode=indexing
                            n455 = property class="Ctl"(reference=w828, "Blinking"=w829) -> ()  [unwired: 1 in, 2 out]
                          }
                        }
                        frame 2 {
                          n456 = control-ref of="1 20"() -> (w830:refnum<vi>)
                          n457 = property class="Clust (严格)"(reference=w830) -> ("Controls[]"=w832:refnum<vi>[])  [unwired: 1 in, 2 out]
                          n458 = for {
                            tunnel: w832 -> [w833] mode=indexing
                            tunnel: w831 -> [w834] mode=indexing
                            n459 = property class="Ctl"(reference=w833, "Blinking"=w834) -> ()  [unwired: 1 in, 2 out]
                          }
                        }
                        frame 3 {
                          n460 = control-ref of="1 21"() -> (w835:refnum<vi>)
                          n461 = property class="Clust (严格)"(reference=w835) -> ("Controls[]"=w837:refnum<vi>[])  [unwired: 1 in, 2 out]
                          n462 = for {
                            tunnel: w837 -> [w838] mode=indexing
                            tunnel: w836 -> [w839] mode=indexing
                            n463 = property class="Ctl"(reference=w838, "Blinking"=w839) -> ()  [unwired: 1 in, 2 out]
                          }
                        }
                        frame 4 {
                          n464 = control-ref of="1 22"() -> (w840:refnum<vi>)
                          n465 = property class="Clust (严格)"(reference=w840) -> ("Controls[]"=w842:refnum<vi>[])  [unwired: 1 in, 2 out]
                          n466 = for {
                            tunnel: w842 -> [w843] mode=indexing
                            tunnel: w841 -> [w844] mode=indexing
                            n467 = property class="Ctl"(reference=w843, "Blinking"=w844) -> ()  [unwired: 1 in, 2 out]
                          }
                        }
                        frame 5 {
                          n468 = control-ref of="1 23"() -> (w845:refnum<vi>)
                          n469 = property class="Clust (严格)"(reference=w845) -> ("Controls[]"=w847:refnum<vi>[])  [unwired: 1 in, 2 out]
                          n470 = for {
                            tunnel: w847 -> [w848] mode=indexing
                            tunnel: w846 -> [w849] mode=indexing
                            n471 = property class="Ctl"(reference=w848, "Blinking"=w849) -> ()  [unwired: 1 in, 2 out]
                          }
                        }
                        frame 6 {
                          n472 = control-ref of="1 24"() -> (w850:refnum<vi>)
                          n473 = property class="Clust (严格)"(reference=w850) -> ("Controls[]"=w852:refnum<vi>[])  [unwired: 1 in, 2 out]
                          n474 = for {
                            tunnel: w852 -> [w853] mode=indexing
                            tunnel: w851 -> [w854] mode=indexing
                            n475 = property class="Ctl"(reference=w853, "Blinking"=w854) -> ()  [unwired: 1 in, 2 out]
                          }
                        }
                        frame 7 {
                          n476 = control-ref of="1 25"() -> (w855:refnum<vi>)
                          n477 = property class="Clust (严格)"(reference=w855) -> ("Controls[]"=w857:refnum<vi>[])  [unwired: 1 in, 2 out]
                          n478 = for {
                            tunnel: w857 -> [w858] mode=indexing
                            tunnel: w856 -> [w859] mode=indexing
                            n479 = property class="Ctl"(reference=w858, "Blinking"=w859) -> ()  [unwired: 1 in, 2 out]
                          }
                        }
                        frame 8 {
                          n480 = control-ref of="1 6"() -> (w860:refnum<vi>)
                          n481 = property class="Clust (严格)"(reference=w860) -> ("Controls[]"=w862:refnum<vi>[])  [unwired: 1 in, 2 out]
                          n482 = for {
                            tunnel: w862 -> [w863] mode=indexing
                            tunnel: w861 -> [w864] mode=indexing
                            n483 = property class="Ctl"(reference=w863, "Blinking"=w864) -> ()  [unwired: 1 in, 2 out]
                          }
                        }
                        frame 99, Default {
                        }
                      }
                    }
                  }
                }
                n484 = local write "一次置位"(FALSE ("一次置位")) -> ()
              }
            }
          }
          frame True {
            n485 = case shown="\"单体电压\", 默认" w866 {
              frame "单体电压", Default {
                w870 = 17 ("y")
                n486 = global read "单体信息全局.vi" "数据"() -> (w883:dbl[])
                n487 = global read "单体信息全局.vi" "PF"() -> (w869:i32)
                n488 = Array Subset(array=w883, length=w869) -> (w882:dbl[])  [unwired: 1 in]
                n489 = Subtract(x="基准", y="偏差") -> (x-y=w879:dbl)
                n490 = Quotient & Remainder(x=w869, y=12) -> (x-y*floor(x/y)=w875:i32, floor(x/y)=w873:i32)
                n491 = Add(x="基准", y="偏差") -> (x+y=w878:dbl)
                n492 = Equal To 0?(x=w875) -> (x = 0?=w874:bool)
                n493 = In Range and Coerce(upper limit=w878, x=w882, lower limit=w879) -> (In Range?=w877:bool[])  [unwired: 1 out]
                n494 = Increment(x=w873) -> (x+1=w872:i32)
                n495 = Select(t=w873, s=w874, f=w872) -> (s? t:f=w868:i32)
                n496 = Not(x=w877) -> (.not. x?=w867:bool[])
                n497 = Greater Or Equal?(x=w868, y=w870) -> (x >= y?=w871:bool)
                n498 = case shown="真" w871 {
                  tunnel: w868 -> [w973 _]
                  tunnel: w870 -> [w970 _]
                  tunnel: w867 -> [w971 _]
                  frame True {
                    n499 = Decrement(x=w970) -> (x-1=w969:i32)
                    n500 = Subtract(x=w973, y=w969) -> (x-y=w972:i32)
                    n501 = for {
                      N: w972 -> [_]
                      tunnel: w971 -> [w979]
                      tunnel: w969 -> [w974]
                      i -> [w980]
                      w977 = 12 ("y")
                      n502 = Add(x=w974, y=w980) -> (x+y=w975:i32)
                      n503 = Multiply(x=w975, y=w977) -> (x*y=w978:i32)
                      n504 = Array Subset(array=w979, index=w978, length=w977) -> (w976:bool[])
                      n505 = case shown="0" w980 {
                        tunnel: w976 -> [w982 w987 w992 w997 w1002 w1007 w1012 w1017 w1022 _]
                        frame 0 {
                          n506 = control-ref of="1 18"() -> (w981:refnum<vi>)
                          n507 = property class="Clust (严格)"(reference=w981) -> ("Controls[]"=w983:refnum<vi>[])  [unwired: 1 in, 2 out]
                          n508 = for {
                            tunnel: w983 -> [w984] mode=indexing
                            tunnel: w982 -> [w985] mode=indexing
                            n509 = property class="Ctl"(reference=w984, "Blinking"=w985) -> ()  [unwired: 1 in, 2 out]
                          }
                        }
                        frame 1 {
                          n510 = control-ref of="1 19"() -> (w986:refnum<vi>)
                          n511 = property class="Clust (严格)"(reference=w986) -> ("Controls[]"=w988:refnum<vi>[])  [unwired: 1 in, 2 out]
                          n512 = for {
                            tunnel: w988 -> [w989] mode=indexing
                            tunnel: w987 -> [w990] mode=indexing
                            n513 = property class="Ctl"(reference=w989, "Blinking"=w990) -> ()  [unwired: 1 in, 2 out]
                          }
                        }
                        frame 2 {
                          n514 = control-ref of="1 20"() -> (w991:refnum<vi>)
                          n515 = property class="Clust (严格)"(reference=w991) -> ("Controls[]"=w993:refnum<vi>[])  [unwired: 1 in, 2 out]
                          n516 = for {
                            tunnel: w993 -> [w994] mode=indexing
                            tunnel: w992 -> [w995] mode=indexing
                            n517 = property class="Ctl"(reference=w994, "Blinking"=w995) -> ()  [unwired: 1 in, 2 out]
                          }
                        }
                        frame 3 {
                          n518 = control-ref of="1 21"() -> (w996:refnum<vi>)
                          n519 = property class="Clust (严格)"(reference=w996) -> ("Controls[]"=w998:refnum<vi>[])  [unwired: 1 in, 2 out]
                          n520 = for {
                            tunnel: w998 -> [w999] mode=indexing
                            tunnel: w997 -> [w1000] mode=indexing
                            n521 = property class="Ctl"(reference=w999, "Blinking"=w1000) -> ()  [unwired: 1 in, 2 out]
                          }
                        }
                        frame 4 {
                          n522 = control-ref of="1 22"() -> (w1001:refnum<vi>)
                          n523 = property class="Clust (严格)"(reference=w1001) -> ("Controls[]"=w1003:refnum<vi>[])  [unwired: 1 in, 2 out]
                          n524 = for {
                            tunnel: w1003 -> [w1004] mode=indexing
                            tunnel: w1002 -> [w1005] mode=indexing
                            n525 = property class="Ctl"(reference=w1004, "Blinking"=w1005) -> ()  [unwired: 1 in, 2 out]
                          }
                        }
                        frame 5 {
                          n526 = control-ref of="1 23"() -> (w1006:refnum<vi>)
                          n527 = property class="Clust (严格)"(reference=w1006) -> ("Controls[]"=w1008:refnum<vi>[])  [unwired: 1 in, 2 out]
                          n528 = for {
                            tunnel: w1008 -> [w1009] mode=indexing
                            tunnel: w1007 -> [w1010] mode=indexing
                            n529 = property class="Ctl"(reference=w1009, "Blinking"=w1010) -> ()  [unwired: 1 in, 2 out]
                          }
                        }
                        frame 6 {
                          n530 = control-ref of="1 24"() -> (w1011:refnum<vi>)
                          n531 = property class="Clust (严格)"(reference=w1011) -> ("Controls[]"=w1013:refnum<vi>[])  [unwired: 1 in, 2 out]
                          n532 = for {
                            tunnel: w1013 -> [w1014] mode=indexing
                            tunnel: w1012 -> [w1015] mode=indexing
                            n533 = property class="Ctl"(reference=w1014, "Blinking"=w1015) -> ()  [unwired: 1 in, 2 out]
                          }
                        }
                        frame 7 {
                          n534 = control-ref of="1 25"() -> (w1016:refnum<vi>)
                          n535 = property class="Clust (严格)"(reference=w1016) -> ("Controls[]"=w1018:refnum<vi>[])  [unwired: 1 in, 2 out]
                          n536 = for {
                            tunnel: w1018 -> [w1019] mode=indexing
                            tunnel: w1017 -> [w1020] mode=indexing
                            n537 = property class="Ctl"(reference=w1019, "Blinking"=w1020) -> ()  [unwired: 1 in, 2 out]
                          }
                        }
                        frame 8 {
                          n538 = control-ref of="1 5"() -> (w1021:refnum<vi>)
                          n539 = property class="Clust (严格)"(reference=w1021) -> ("Controls[]"=w1023:refnum<vi>[])  [unwired: 1 in, 2 out]
                          n540 = for {
                            tunnel: w1023 -> [w1024] mode=indexing
                            tunnel: w1022 -> [w1025] mode=indexing
                            n541 = property class="Ctl"(reference=w1024, "Blinking"=w1025) -> ()  [unwired: 1 in, 2 out]
                          }
                        }
                        frame 99, Default {
                        }
                      }
                    }
                  }
                  frame False {
                  }
                }
                n542 = for {
                  N: w868 -> [_]
                  tunnel: w867 -> [w887]
                  i -> [w888]
                  w885 = 12 ("y")
                  n543 = Multiply(x=w888, y=w885) -> (x*y=w886:i32)
                  n544 = Array Subset(array=w887, index=w886, length=w885) -> (w884:bool[])
                  n545 = case shown="7" w888 {
                    tunnel: w884 -> [w889 w895 w900 w905 w910 w915 w920 w925 w930 w935 w940 w945 w950 w955 w960 w965 _]
                    frame 0 {
                      n546 = control-ref of="1 102"() -> (w891:refnum<vi>)
                      n547 = property class="Clust (严格)"(reference=w891) -> ("Controls[]"=w890:refnum<vi>[])  [unwired: 1 in, 2 out]
                      n548 = for {
                        tunnel: w890 -> [w892] mode=indexing
                        tunnel: w889 -> [w893] mode=indexing
                        n549 = property class="Ctl"(reference=w892, "Blinking"=w893) -> ()  [unwired: 1 in, 2 out]
                      }
                    }
                    frame 1 {
                      n550 = control-ref of="1 3"() -> (w894:refnum<vi>)
                      n551 = property class="Clust (严格)"(reference=w894) -> ("Controls[]"=w896:refnum<vi>[])  [unwired: 1 in, 2 out]
                      n552 = for {
                        tunnel: w896 -> [w897] mode=indexing
                        tunnel: w895 -> [w898] mode=indexing
                        n553 = property class="Ctl"(reference=w897, "Blinking"=w898) -> ()  [unwired: 1 in, 2 out]
                      }
                    }
                    frame 2 {
                      n554 = control-ref of="1 4"() -> (w899:refnum<vi>)
                      n555 = property class="Clust (严格)"(reference=w899) -> ("Controls[]"=w901:refnum<vi>[])  [unwired: 1 in, 2 out]
                      n556 = for {
                        tunnel: w901 -> [w902] mode=indexing
                        tunnel: w900 -> [w903] mode=indexing
                        n557 = property class="Ctl"(reference=w902, "Blinking"=w903) -> ()  [unwired: 1 in, 2 out]
                      }
                    }
                    frame 3 {
                      n558 = control-ref of="1 6"() -> (w904:refnum<vi>)
                      n559 = property class="Clust (严格)"(reference=w904) -> ("Controls[]"=w906:refnum<vi>[])  [unwired: 1 in, 2 out]
                      n560 = for {
                        tunnel: w906 -> [w907] mode=indexing
                        tunnel: w905 -> [w908] mode=indexing
                        n561 = property class="Ctl"(reference=w907, "Blinking"=w908) -> ()  [unwired: 1 in, 2 out]
                      }
                    }
                    frame 4 {
                      n562 = control-ref of="1 7"() -> (w909:refnum<vi>)
                      n563 = property class="Clust (严格)"(reference=w909) -> ("Controls[]"=w911:refnum<vi>[])  [unwired: 1 in, 2 out]
                      n564 = for {
                        tunnel: w911 -> [w912] mode=indexing
                        tunnel: w910 -> [w913] mode=indexing
                        n565 = property class="Ctl"(reference=w912, "Blinking"=w913) -> ()  [unwired: 1 in, 2 out]
                      }
                    }
                    frame 5 {
                      n566 = control-ref of="1 8"() -> (w914:refnum<vi>)
                      n567 = property class="Clust (严格)"(reference=w914) -> ("Controls[]"=w916:refnum<vi>[])  [unwired: 1 in, 2 out]
                      n568 = for {
                        tunnel: w916 -> [w917] mode=indexing
                        tunnel: w915 -> [w918] mode=indexing
                        n569 = property class="Ctl"(reference=w917, "Blinking"=w918) -> ()  [unwired: 1 in, 2 out]
                      }
                    }
                    frame 6 {
                      n570 = control-ref of="1 9"() -> (w919:refnum<vi>)
                      n571 = property class="Clust (严格)"(reference=w919) -> ("Controls[]"=w921:refnum<vi>[])  [unwired: 1 in, 2 out]
                      n572 = for {
                        tunnel: w921 -> [w922] mode=indexing
                        tunnel: w920 -> [w923] mode=indexing
                        n573 = property class="Ctl"(reference=w922, "Blinking"=w923) -> ()  [unwired: 1 in, 2 out]
                      }
                    }
                    frame 7 {
                      n574 = control-ref of="1 10"() -> (w924:refnum<vi>)
                      n575 = property class="Clust (严格)"(reference=w924) -> ("Controls[]"=w926:refnum<vi>[])  [unwired: 1 in, 2 out]
                      n576 = for {
                        tunnel: w926 -> [w927] mode=indexing
                        tunnel: w925 -> [w928] mode=indexing
                        n577 = property class="Ctl"(reference=w927, "Blinking"=w928) -> ()  [unwired: 1 in, 2 out]
                      }
                    }
                    frame 8 {
                      n578 = control-ref of="1 26"() -> (w929:refnum<vi>)
                      n579 = property class="Clust (严格)"(reference=w929) -> ("Controls[]"=w931:refnum<vi>[])  [unwired: 1 in, 2 out]
                      n580 = for {
                        tunnel: w931 -> [w932] mode=indexing
                        tunnel: w930 -> [w933] mode=indexing
                        n581 = property class="Ctl"(reference=w932, "Blinking"=w933) -> ()  [unwired: 1 in, 2 out]
                      }
                    }
                    frame 9 {
                      n582 = control-ref of="1 27"() -> (w934:refnum<vi>)
                      n583 = property class="Clust (严格)"(reference=w934) -> ("Controls[]"=w936:refnum<vi>[])  [unwired: 1 in, 2 out]
                      n584 = for {
                        tunnel: w936 -> [w937] mode=indexing
                        tunnel: w935 -> [w938] mode=indexing
                        n585 = property class="Ctl"(reference=w937, "Blinking"=w938) -> ()  [unwired: 1 in, 2 out]
                      }
                    }
                    frame 10 {
                      n586 = control-ref of="1 28"() -> (w939:refnum<vi>)
                      n587 = property class="Clust (严格)"(reference=w939) -> ("Controls[]"=w941:refnum<vi>[])  [unwired: 1 in, 2 out]
                      n588 = for {
                        tunnel: w941 -> [w942] mode=indexing
                        tunnel: w940 -> [w943] mode=indexing
                        n589 = property class="Ctl"(reference=w942, "Blinking"=w943) -> ()  [unwired: 1 in, 2 out]
                      }
                    }
                    frame 11 {
                      n590 = control-ref of="1 29"() -> (w944:refnum<vi>)
                      n591 = property class="Clust (严格)"(reference=w944) -> ("Controls[]"=w946:refnum<vi>[])  [unwired: 1 in, 2 out]
                      n592 = for {
                        tunnel: w946 -> [w947] mode=indexing
                        tunnel: w945 -> [w948] mode=indexing
                        n593 = property class="Ctl"(reference=w947, "Blinking"=w948) -> ()  [unwired: 1 in, 2 out]
                      }
                    }
                    frame 12 {
                      n594 = control-ref of="1 30"() -> (w949:refnum<vi>)
                      n595 = property class="Clust (严格)"(reference=w949) -> ("Controls[]"=w951:refnum<vi>[])  [unwired: 1 in, 2 out]
                      n596 = for {
                        tunnel: w951 -> [w952] mode=indexing
                        tunnel: w950 -> [w953] mode=indexing
                        n597 = property class="Ctl"(reference=w952, "Blinking"=w953) -> ()  [unwired: 1 in, 2 out]
                      }
                    }
                    frame 13 {
                      n598 = control-ref of="1 31"() -> (w954:refnum<vi>)
                      n599 = property class="Clust (严格)"(reference=w954) -> ("Controls[]"=w956:refnum<vi>[])  [unwired: 1 in, 2 out]
                      n600 = for {
                        tunnel: w956 -> [w957] mode=indexing
                        tunnel: w955 -> [w958] mode=indexing
                        n601 = property class="Ctl"(reference=w957, "Blinking"=w958) -> ()  [unwired: 1 in, 2 out]
                      }
                    }
                    frame 14 {
                      n602 = control-ref of="1 32"() -> (w959:refnum<vi>)
                      n603 = property class="Clust (严格)"(reference=w959) -> ("Controls[]"=w961:refnum<vi>[])  [unwired: 1 in, 2 out]
                      n604 = for {
                        tunnel: w961 -> [w962] mode=indexing
                        tunnel: w960 -> [w963] mode=indexing
                        n605 = property class="Ctl"(reference=w962, "Blinking"=w963) -> ()  [unwired: 1 in, 2 out]
                      }
                    }
                    frame 15 {
                      n606 = control-ref of="1 33"() -> (w964:refnum<vi>)
                      n607 = property class="Clust (严格)"(reference=w964) -> ("Controls[]"=w966:refnum<vi>[])  [unwired: 1 in, 2 out]
                      n608 = for {
                        tunnel: w966 -> [w967] mode=indexing
                        tunnel: w965 -> [w968] mode=indexing
                        n609 = property class="Ctl"(reference=w967, "Blinking"=w968) -> ()  [unwired: 1 in, 2 out]
                      }
                    }
                    frame 99, Default {
                    }
                  }
                }
              }
              frame "单体温度" {
                w1029 = 17 ("y")
                n610 = global read "单体信息全局.vi" "PF2"() -> (w1028:i32)
                n611 = global read "单体信息全局.vi" "数据 2"() -> (w1042:dbl[])
                n612 = Array Subset(array=w1042, length=w1028) -> (w1041:dbl[])  [unwired: 1 in]
                n613 = Subtract(x="基准", y="偏差") -> (x-y=w1038:dbl)
                n614 = Quotient & Remainder(x=w1028, y=12) -> (x-y*floor(x/y)=w1034:i32, floor(x/y)=w1032:i32)
                n615 = Add(x="基准", y="偏差") -> (x+y=w1037:dbl)
                n616 = Equal To 0?(x=w1034) -> (x = 0?=w1033:bool)
                n617 = In Range and Coerce(upper limit=w1037, x=w1041, lower limit=w1038) -> (In Range?=w1036:bool[])  [unwired: 1 out]
                n618 = Increment(x=w1032) -> (x+1=w1031:i32)
                n619 = Select(t=w1032, s=w1033, f=w1031) -> (s? t:f=w1027:i32)
                n620 = Not(x=w1036) -> (.not. x?=w1026:bool[])
                n621 = Greater Or Equal?(x=w1027, y=w1029) -> (x >= y?=w1030:bool)
                n622 = case shown="真" w1030 {
                  tunnel: w1027 -> [w1132 _]
                  tunnel: w1029 -> [w1129 _]
                  tunnel: w1026 -> [w1130 _]
                  frame True {
                    n623 = Decrement(x=w1129) -> (x-1=w1128:i32)
                    n624 = Subtract(x=w1132, y=w1128) -> (x-y=w1131:i32)
                    n625 = for {
                      N: w1131 -> [_]
                      tunnel: w1130 -> [w1138]
                      tunnel: w1128 -> [w1133]
                      i -> [w1139]
                      w1136 = 12 ("y")
                      n626 = Add(x=w1133, y=w1139) -> (x+y=w1134:i32)
                      n627 = Multiply(x=w1134, y=w1136) -> (x*y=w1137:i32)
                      n628 = Array Subset(array=w1138, index=w1137, length=w1136) -> (w1135:bool[])
                      n629 = case shown="0" w1139 {
                        tunnel: w1135 -> [w1141 w1146 w1151 w1156 w1161 w1166 w1171 w1176 w1181 _]
                        frame 0 {
                          n630 = control-ref of="1 18"() -> (w1140:refnum<vi>)
                          n631 = property class="Clust (严格)"(reference=w1140) -> ("Controls[]"=w1142:refnum<vi>[])  [unwired: 1 in, 2 out]
                          n632 = for {
                            tunnel: w1142 -> [w1143] mode=indexing
                            tunnel: w1141 -> [w1144] mode=indexing
                            n633 = property class="Ctl"(reference=w1143, "Blinking"=w1144) -> ()  [unwired: 1 in, 2 out]
                          }
                        }
                        frame 1 {
                          n634 = control-ref of="1 19"() -> (w1145:refnum<vi>)
                          n635 = property class="Clust (严格)"(reference=w1145) -> ("Controls[]"=w1147:refnum<vi>[])  [unwired: 1 in, 2 out]
                          n636 = for {
                            tunnel: w1147 -> [w1148] mode=indexing
                            tunnel: w1146 -> [w1149] mode=indexing
                            n637 = property class="Ctl"(reference=w1148, "Blinking"=w1149) -> ()  [unwired: 1 in, 2 out]
                          }
                        }
                        frame 2 {
                          n638 = control-ref of="1 20"() -> (w1150:refnum<vi>)
                          n639 = property class="Clust (严格)"(reference=w1150) -> ("Controls[]"=w1152:refnum<vi>[])  [unwired: 1 in, 2 out]
                          n640 = for {
                            tunnel: w1152 -> [w1153] mode=indexing
                            tunnel: w1151 -> [w1154] mode=indexing
                            n641 = property class="Ctl"(reference=w1153, "Blinking"=w1154) -> ()  [unwired: 1 in, 2 out]
                          }
                        }
                        frame 3 {
                          n642 = control-ref of="1 21"() -> (w1155:refnum<vi>)
                          n643 = property class="Clust (严格)"(reference=w1155) -> ("Controls[]"=w1157:refnum<vi>[])  [unwired: 1 in, 2 out]
                          n644 = for {
                            tunnel: w1157 -> [w1158] mode=indexing
                            tunnel: w1156 -> [w1159] mode=indexing
                            n645 = property class="Ctl"(reference=w1158, "Blinking"=w1159) -> ()  [unwired: 1 in, 2 out]
                          }
                        }
                        frame 4 {
                          n646 = control-ref of="1 22"() -> (w1160:refnum<vi>)
                          n647 = property class="Clust (严格)"(reference=w1160) -> ("Controls[]"=w1162:refnum<vi>[])  [unwired: 1 in, 2 out]
                          n648 = for {
                            tunnel: w1162 -> [w1163] mode=indexing
                            tunnel: w1161 -> [w1164] mode=indexing
                            n649 = property class="Ctl"(reference=w1163, "Blinking"=w1164) -> ()  [unwired: 1 in, 2 out]
                          }
                        }
                        frame 5 {
                          n650 = control-ref of="1 23"() -> (w1165:refnum<vi>)
                          n651 = property class="Clust (严格)"(reference=w1165) -> ("Controls[]"=w1167:refnum<vi>[])  [unwired: 1 in, 2 out]
                          n652 = for {
                            tunnel: w1167 -> [w1168] mode=indexing
                            tunnel: w1166 -> [w1169] mode=indexing
                            n653 = property class="Ctl"(reference=w1168, "Blinking"=w1169) -> ()  [unwired: 1 in, 2 out]
                          }
                        }
                        frame 6 {
                          n654 = control-ref of="1 24"() -> (w1170:refnum<vi>)
                          n655 = property class="Clust (严格)"(reference=w1170) -> ("Controls[]"=w1172:refnum<vi>[])  [unwired: 1 in, 2 out]
                          n656 = for {
                            tunnel: w1172 -> [w1173] mode=indexing
                            tunnel: w1171 -> [w1174] mode=indexing
                            n657 = property class="Ctl"(reference=w1173, "Blinking"=w1174) -> ()  [unwired: 1 in, 2 out]
                          }
                        }
                        frame 7 {
                          n658 = control-ref of="1 25"() -> (w1175:refnum<vi>)
                          n659 = property class="Clust (严格)"(reference=w1175) -> ("Controls[]"=w1177:refnum<vi>[])  [unwired: 1 in, 2 out]
                          n660 = for {
                            tunnel: w1177 -> [w1178] mode=indexing
                            tunnel: w1176 -> [w1179] mode=indexing
                            n661 = property class="Ctl"(reference=w1178, "Blinking"=w1179) -> ()  [unwired: 1 in, 2 out]
                          }
                        }
                        frame 8 {
                          n662 = control-ref of="1 6"() -> (w1180:refnum<vi>)
                          n663 = property class="Clust (严格)"(reference=w1180) -> ("Controls[]"=w1182:refnum<vi>[])  [unwired: 1 in, 2 out]
                          n664 = for {
                            tunnel: w1182 -> [w1183] mode=indexing
                            tunnel: w1181 -> [w1184] mode=indexing
                            n665 = property class="Ctl"(reference=w1183, "Blinking"=w1184) -> ()  [unwired: 1 in, 2 out]
                          }
                        }
                        frame 99, Default {
                        }
                      }
                    }
                  }
                  frame False {
                  }
                }
                n666 = for {
                  N: w1027 -> [_]
                  tunnel: w1026 -> [w1046]
                  i -> [w1047]
                  w1044 = 12 ("y")
                  n667 = Multiply(x=w1047, y=w1044) -> (x*y=w1045:i32)
                  n668 = Array Subset(array=w1046, index=w1045, length=w1044) -> (w1043:bool[])
                  n669 = case shown="15" w1047 {
                    tunnel: w1043 -> [w1049 w1054 w1059 w1064 w1069 w1074 w1079 w1084 w1089 w1094 w1099 w1104 w1109 w1114 w1119 w1124 _]
                    frame 0 {
                      n670 = control-ref of="1 102"() -> (w1048:refnum<vi>)
                      n671 = property class="Clust (严格)"(reference=w1048) -> ("Controls[]"=w1050:refnum<vi>[])  [unwired: 1 in, 2 out]
                      n672 = for {
                        tunnel: w1050 -> [w1051] mode=indexing
                        tunnel: w1049 -> [w1052] mode=indexing
                        n673 = property class="Ctl"(reference=w1051, "Blinking"=w1052) -> ()  [unwired: 1 in, 2 out]
                      }
                    }
                    frame 1 {
                      n674 = control-ref of="1 3"() -> (w1053:refnum<vi>)
                      n675 = property class="Clust (严格)"(reference=w1053) -> ("Controls[]"=w1055:refnum<vi>[])  [unwired: 1 in, 2 out]
                      n676 = for {
                        tunnel: w1055 -> [w1056] mode=indexing
                        tunnel: w1054 -> [w1057] mode=indexing
                        n677 = property class="Ctl"(reference=w1056, "Blinking"=w1057) -> ()  [unwired: 1 in, 2 out]
                      }
                    }
                    frame 2 {
                      n678 = control-ref of="1 4"() -> (w1058:refnum<vi>)
                      n679 = property class="Clust (严格)"(reference=w1058) -> ("Controls[]"=w1060:refnum<vi>[])  [unwired: 1 in, 2 out]
                      n680 = for {
                        tunnel: w1060 -> [w1061] mode=indexing
                        tunnel: w1059 -> [w1062] mode=indexing
                        n681 = property class="Ctl"(reference=w1061, "Blinking"=w1062) -> ()  [unwired: 1 in, 2 out]
                      }
                    }
                    frame 3 {
                      n682 = control-ref of="1 6"() -> (w1063:refnum<vi>)
                      n683 = property class="Clust (严格)"(reference=w1063) -> ("Controls[]"=w1065:refnum<vi>[])  [unwired: 1 in, 2 out]
                      n684 = for {
                        tunnel: w1065 -> [w1066] mode=indexing
                        tunnel: w1064 -> [w1067] mode=indexing
                        n685 = property class="Ctl"(reference=w1066, "Blinking"=w1067) -> ()  [unwired: 1 in, 2 out]
                      }
                    }
                    frame 4 {
                      n686 = control-ref of="1 7"() -> (w1068:refnum<vi>)
                      n687 = property class="Clust (严格)"(reference=w1068) -> ("Controls[]"=w1070:refnum<vi>[])  [unwired: 1 in, 2 out]
                      n688 = for {
                        tunnel: w1070 -> [w1071] mode=indexing
                        tunnel: w1069 -> [w1072] mode=indexing
                        n689 = property class="Ctl"(reference=w1071, "Blinking"=w1072) -> ()  [unwired: 1 in, 2 out]
                      }
                    }
                    frame 5 {
                      n690 = control-ref of="1 8"() -> (w1073:refnum<vi>)
                      n691 = property class="Clust (严格)"(reference=w1073) -> ("Controls[]"=w1075:refnum<vi>[])  [unwired: 1 in, 2 out]
                      n692 = for {
                        tunnel: w1075 -> [w1076] mode=indexing
                        tunnel: w1074 -> [w1077] mode=indexing
                        n693 = property class="Ctl"(reference=w1076, "Blinking"=w1077) -> ()  [unwired: 1 in, 2 out]
                      }
                    }
                    frame 6 {
                      n694 = control-ref of="1 9"() -> (w1078:refnum<vi>)
                      n695 = property class="Clust (严格)"(reference=w1078) -> ("Controls[]"=w1080:refnum<vi>[])  [unwired: 1 in, 2 out]
                      n696 = for {
                        tunnel: w1080 -> [w1081] mode=indexing
                        tunnel: w1079 -> [w1082] mode=indexing
                        n697 = property class="Ctl"(reference=w1081, "Blinking"=w1082) -> ()  [unwired: 1 in, 2 out]
                      }
                    }
                    frame 7 {
                      n698 = control-ref of="1 10"() -> (w1083:refnum<vi>)
                      n699 = property class="Clust (严格)"(reference=w1083) -> ("Controls[]"=w1085:refnum<vi>[])  [unwired: 1 in, 2 out]
                      n700 = for {
                        tunnel: w1085 -> [w1086] mode=indexing
                        tunnel: w1084 -> [w1087] mode=indexing
                        n701 = property class="Ctl"(reference=w1086, "Blinking"=w1087) -> ()  [unwired: 1 in, 2 out]
                      }
                    }
                    frame 8 {
                      n702 = control-ref of="1 26"() -> (w1088:refnum<vi>)
                      n703 = property class="Clust (严格)"(reference=w1088) -> ("Controls[]"=w1090:refnum<vi>[])  [unwired: 1 in, 2 out]
                      n704 = for {
                        tunnel: w1090 -> [w1091] mode=indexing
                        tunnel: w1089 -> [w1092] mode=indexing
                        n705 = property class="Ctl"(reference=w1091, "Blinking"=w1092) -> ()  [unwired: 1 in, 2 out]
                      }
                    }
                    frame 9 {
                      n706 = control-ref of="1 27"() -> (w1093:refnum<vi>)
                      n707 = property class="Clust (严格)"(reference=w1093) -> ("Controls[]"=w1095:refnum<vi>[])  [unwired: 1 in, 2 out]
                      n708 = for {
                        tunnel: w1095 -> [w1096] mode=indexing
                        tunnel: w1094 -> [w1097] mode=indexing
                        n709 = property class="Ctl"(reference=w1096, "Blinking"=w1097) -> ()  [unwired: 1 in, 2 out]
                      }
                    }
                    frame 10 {
                      n710 = control-ref of="1 28"() -> (w1098:refnum<vi>)
                      n711 = property class="Clust (严格)"(reference=w1098) -> ("Controls[]"=w1100:refnum<vi>[])  [unwired: 1 in, 2 out]
                      n712 = for {
                        tunnel: w1100 -> [w1101] mode=indexing
                        tunnel: w1099 -> [w1102] mode=indexing
                        n713 = property class="Ctl"(reference=w1101, "Blinking"=w1102) -> ()  [unwired: 1 in, 2 out]
                      }
                    }
                    frame 11 {
                      n714 = control-ref of="1 29"() -> (w1103:refnum<vi>)
                      n715 = property class="Clust (严格)"(reference=w1103) -> ("Controls[]"=w1105:refnum<vi>[])  [unwired: 1 in, 2 out]
                      n716 = for {
                        tunnel: w1105 -> [w1106] mode=indexing
                        tunnel: w1104 -> [w1107] mode=indexing
                        n717 = property class="Ctl"(reference=w1106, "Blinking"=w1107) -> ()  [unwired: 1 in, 2 out]
                      }
                    }
                    frame 12 {
                      n718 = control-ref of="1 30"() -> (w1108:refnum<vi>)
                      n719 = property class="Clust (严格)"(reference=w1108) -> ("Controls[]"=w1110:refnum<vi>[])  [unwired: 1 in, 2 out]
                      n720 = for {
                        tunnel: w1110 -> [w1111] mode=indexing
                        tunnel: w1109 -> [w1112] mode=indexing
                        n721 = property class="Ctl"(reference=w1111, "Blinking"=w1112) -> ()  [unwired: 1 in, 2 out]
                      }
                    }
                    frame 13 {
                      n722 = control-ref of="1 31"() -> (w1113:refnum<vi>)
                      n723 = property class="Clust (严格)"(reference=w1113) -> ("Controls[]"=w1115:refnum<vi>[])  [unwired: 1 in, 2 out]
                      n724 = for {
                        tunnel: w1115 -> [w1116] mode=indexing
                        tunnel: w1114 -> [w1117] mode=indexing
                        n725 = property class="Ctl"(reference=w1116, "Blinking"=w1117) -> ()  [unwired: 1 in, 2 out]
                      }
                    }
                    frame 14 {
                      n726 = control-ref of="1 32"() -> (w1118:refnum<vi>)
                      n727 = property class="Clust (严格)"(reference=w1118) -> ("Controls[]"=w1120:refnum<vi>[])  [unwired: 1 in, 2 out]
                      n728 = for {
                        tunnel: w1120 -> [w1121] mode=indexing
                        tunnel: w1119 -> [w1122] mode=indexing
                        n729 = property class="Ctl"(reference=w1121, "Blinking"=w1122) -> ()  [unwired: 1 in, 2 out]
                      }
                    }
                    frame 15 {
                      n730 = control-ref of="1 33"() -> (w1123:refnum<vi>)
                      n731 = property class="Clust (严格)"(reference=w1123) -> ("Controls[]"=w1125:refnum<vi>[])  [unwired: 1 in, 2 out]
                      n732 = for {
                        tunnel: w1125 -> [w1126] mode=indexing
                        tunnel: w1124 -> [w1127] mode=indexing
                        n733 = property class="Ctl"(reference=w1126, "Blinking"=w1127) -> ()  [unwired: 1 in, 2 out]
                      }
                    }
                    frame 99, Default {
                    }
                  }
                }
              }
            }
            n734 = local write "一次置位"(TRUE ("一次置位")) -> ()
          }
        }
      }
    }
    frame Disabled {
    }
  }
  n735 = while {
    shift-right: [w1188] -> _
    shift-left: w1 -> [w1187]
    shift-left: w1 -> [w1186]
    stop <- w1189 stop-if-true
    n736 = event shown="[0] 超时" {
      selector: _ -> [_ _ _ _]
      dyn-events: _ -> [_ _ _ _]
      timeout: 100 -> [_ _ _ _]
      tunnel: [_ _ w1367 w1373] -> w1189
      tunnel: [w1194 _ _ _] -> w1188
      tunnel: w1187 -> [w1193 _ _ _]
      tunnel: w1186 -> [w1192 _ _ _]
      event Timeout {
        n737 = event-data() -> ()  [unwired: 3 out]
        n738 = local read "选项卡控件"() -> (w1196:enum32{"单体电压", "单体温度", "单体内阻", "单体SOC"})
        n739 = local read "主界面选项"() -> (w1206:T3)
        n740 = case shown="\"单体电压\", 默认" w1196 {
          frame "单体电压", Default {
            n741 = control-ref of="单选选项2 3"() -> (w1208:refnum<vi>)
            n742 = control-ref of="单选选项2 2"() -> (w1209:refnum<vi>)
            n743 = control-ref of="单选选项2"() -> (w1210:refnum<vi>)
            n744 = control-ref of="单选选项1"() -> (w1207:refnum<vi>)
            n745 = local read "故障信息选择按键 2"() -> (w1211:enum32{"单选选项2", "单选选项2 2", "单选选项2 3", "单选选项1"})
            n746 = Build Array(w1210, w1209, w1208, w1207) -> (w1216:refnum<vi>[])
            n747 = case shown="\"单选选项2\"" w1211 {
              selector: w1211 -> [w1223 w1228 w1233 w1238]
              tunnel: [w1222 w1227 w1232 w1237] -> w1213
              tunnel: [w1221 w1226 w1231 w1236] -> w1215
              tunnel: w1216 -> [w1224 w1229 w1234 w1239]
              tunnel: [enum32{"1-96", "97-192", "193-288", "289-300"}."1-96" ("电压选择") enum32{"1-96", "97-192", "193-288", "289-300"}."289-300" ("电压选择") enum32{"1-96", "97-192", "193-288", "289-300"}."193-288" ("电压选择") enum32{"1-96", "97-192", "193-288", "289-300"}."97-192" ("电压选择")] -> w1212
              frame "单选选项1", Default {
                n748 = Delete From Array(array=w1224, index=w1223) -> (deleted portion=w1221:refnum<vi>, array with subset deleted=w1222:refnum<vi>[])  [unwired: 1 in]
              }
              frame "单选选项2 3" {
                n749 = Delete From Array(array=w1229, index=w1228) -> (deleted portion=w1226:refnum<vi>, array with subset deleted=w1227:refnum<vi>[])  [unwired: 1 in]
              }
              frame "单选选项2 2" {
                n750 = Delete From Array(array=w1234, index=w1233) -> (deleted portion=w1231:refnum<vi>, array with subset deleted=w1232:refnum<vi>[])  [unwired: 1 in]
              }
              frame "单选选项2" {
                n751 = Delete From Array(array=w1239, index=w1238) -> (deleted portion=w1236:refnum<vi>, array with subset deleted=w1237:refnum<vi>[])  [unwired: 1 in]
              }
            }
            n752 = local write "电压选择"(w1212) -> ()
            n753 = for {
              tunnel: u32 87470 -> [w1219]
              tunnel: w1213 -> [w1218] mode=indexing
              n754 = property class="Bool (严格)"(reference=w1218, "BoolText.TextColor"=w1219) -> ()  [unwired: 1 in, 2 out]
            }
            n755 = property class="Bool (严格)"(reference=w1215, "BoolText.TextColor"=u32 16777215) -> ()  [unwired: 1 in, 2 out]
          }
          frame "单体温度" {
            n756 = control-ref of="单选选项1"() -> (w1244:refnum<vi>)
            n757 = control-ref of="单选选项2"() -> (w1242:refnum<vi>)
            n758 = control-ref of="单选选项2 3"() -> (w1245:refnum<vi>)
            n759 = control-ref of="单选选项2 2"() -> (w1243:refnum<vi>)
            n760 = local read "故障信息选择按键 3"() -> (w1241:enum32{"单选选项2", "单选选项2 2", "单选选项2 3", "单选选项1"})
            n761 = Build Array(w1242, w1243, w1245, w1244) -> (w1249:refnum<vi>[])
            n762 = case shown="\"单选选项2\"" w1241 {
              selector: w1241 -> [w1256 w1261 w1266 w1271]
              tunnel: [w1255 w1260 w1265 w1270] -> w1246
              tunnel: [w1254 w1259 w1264 w1269] -> w1248
              tunnel: w1249 -> [w1257 w1262 w1267 w1272]
              tunnel: [enum32{"1-96", "97-192", "193-288", "289-300"}."1-96" ("电压选择") enum32{"1-96", "97-192", "193-288", "289-300"}."289-300" ("电压选择") enum32{"1-96", "97-192", "193-288", "289-300"}."193-288" ("电压选择") enum32{"1-96", "97-192", "193-288", "289-300"}."97-192" ("电压选择")] -> w1240
              frame "单选选项1", Default {
                n763 = Delete From Array(array=w1257, index=w1256) -> (deleted portion=w1254:refnum<vi>, array with subset deleted=w1255:refnum<vi>[])  [unwired: 1 in]
              }
              frame "单选选项2 3" {
                n764 = Delete From Array(array=w1262, index=w1261) -> (deleted portion=w1259:refnum<vi>, array with subset deleted=w1260:refnum<vi>[])  [unwired: 1 in]
              }
              frame "单选选项2 2" {
                n765 = Delete From Array(array=w1267, index=w1266) -> (deleted portion=w1264:refnum<vi>, array with subset deleted=w1265:refnum<vi>[])  [unwired: 1 in]
              }
              frame "单选选项2" {
                n766 = Delete From Array(array=w1272, index=w1271) -> (deleted portion=w1269:refnum<vi>, array with subset deleted=w1270:refnum<vi>[])  [unwired: 1 in]
              }
            }
            n767 = local write "电压选择 2"(w1240) -> ()
            n768 = for {
              tunnel: u32 87470 -> [w1252]
              tunnel: w1246 -> [w1251] mode=indexing
              n769 = property class="Bool (严格)"(reference=w1251, "BoolText.TextColor"=w1252) -> ()  [unwired: 1 in, 2 out]
            }
            n770 = property class="Bool (严格)"(reference=w1248, "BoolText.TextColor"=u32 16777215) -> ()  [unwired: 1 in, 2 out]
          }
          frame "单体内阻" {
            n771 = control-ref of="单选选项2 3"() -> (w1278:refnum<vi>)
            n772 = control-ref of="单选选项2"() -> (w1275:refnum<vi>)
            n773 = control-ref of="单选选项2 2"() -> (w1276:refnum<vi>)
            n774 = control-ref of="单选选项1"() -> (w1277:refnum<vi>)
            n775 = local read "故障信息选择按键 4"() -> (w1274:enum32{"单选选项2", "单选选项2 2", "单选选项2 3", "单选选项1"})
            n776 = Build Array(w1275, w1276, w1278, w1277) -> (w1282:refnum<vi>[])
            n777 = case shown="\"单选选项2\"" w1274 {
              selector: w1274 -> [w1289 w1294 w1299 w1304]
              tunnel: [w1288 w1293 w1298 w1303] -> w1279
              tunnel: [w1287 w1292 w1297 w1302] -> w1281
              tunnel: w1282 -> [w1290 w1295 w1300 w1305]
              tunnel: [enum32{"1-96", "97-192", "193-288", "289-300"}."1-96" ("电压选择") enum32{"1-96", "97-192", "193-288", "289-300"}."289-300" ("电压选择") enum32{"1-96", "97-192", "193-288", "289-300"}."193-288" ("电压选择") enum32{"1-96", "97-192", "193-288", "289-300"}."97-192" ("电压选择")] -> w1273
              frame "单选选项1", Default {
                n778 = Delete From Array(array=w1290, index=w1289) -> (deleted portion=w1287:refnum<vi>, array with subset deleted=w1288:refnum<vi>[])  [unwired: 1 in]
              }
              frame "单选选项2 3" {
                n779 = Delete From Array(array=w1295, index=w1294) -> (deleted portion=w1292:refnum<vi>, array with subset deleted=w1293:refnum<vi>[])  [unwired: 1 in]
              }
              frame "单选选项2 2" {
                n780 = Delete From Array(array=w1300, index=w1299) -> (deleted portion=w1297:refnum<vi>, array with subset deleted=w1298:refnum<vi>[])  [unwired: 1 in]
              }
              frame "单选选项2" {
                n781 = Delete From Array(array=w1305, index=w1304) -> (deleted portion=w1302:refnum<vi>, array with subset deleted=w1303:refnum<vi>[])  [unwired: 1 in]
              }
            }
            n782 = local write "电压选择 3"(w1273) -> ()
            n783 = for {
              tunnel: u32 87470 -> [w1285]
              tunnel: w1279 -> [w1284] mode=indexing
              n784 = property class="Bool (严格)"(reference=w1284, "BoolText.TextColor"=w1285) -> ()  [unwired: 1 in, 2 out]
            }
            n785 = property class="Bool (严格)"(reference=w1281, "BoolText.TextColor"=u32 16777215) -> ()  [unwired: 1 in, 2 out]
          }
          frame "单体SOC" {
            n786 = control-ref of="单选选项1"() -> (w1311:refnum<vi>)
            n787 = control-ref of="单选选项2 2"() -> (w1309:refnum<vi>)
            n788 = control-ref of="单选选项2 3"() -> (w1310:refnum<vi>)
            n789 = control-ref of="单选选项2"() -> (w1308:refnum<vi>)
            n790 = local read "故障信息选择按键 5"() -> (w1307:enum32{"单选选项2", "单选选项2 2", "单选选项2 3", "单选选项1"})
            n791 = Build Array(w1308, w1309, w1310, w1311) -> (w1315:refnum<vi>[])
            n792 = case shown="\"单选选项2\"" w1307 {
              selector: w1307 -> [w1322 w1327 w1332 w1337]
              tunnel: [w1321 w1326 w1331 w1336] -> w1312
              tunnel: [w1320 w1325 w1330 w1335] -> w1314
              tunnel: w1315 -> [w1323 w1328 w1333 w1338]
              tunnel: [enum32{"1-96", "97-192", "193-288", "289-300"}."1-96" ("电压选择") enum32{"1-96", "97-192", "193-288", "289-300"}."289-300" ("电压选择") enum32{"1-96", "97-192", "193-288", "289-300"}."193-288" ("电压选择") enum32{"1-96", "97-192", "193-288", "289-300"}."97-192" ("电压选择")] -> w1306
              frame "单选选项1", Default {
                n793 = Delete From Array(array=w1323, index=w1322) -> (deleted portion=w1320:refnum<vi>, array with subset deleted=w1321:refnum<vi>[])  [unwired: 1 in]
              }
              frame "单选选项2 3" {
                n794 = Delete From Array(array=w1328, index=w1327) -> (deleted portion=w1325:refnum<vi>, array with subset deleted=w1326:refnum<vi>[])  [unwired: 1 in]
              }
              frame "单选选项2 2" {
                n795 = Delete From Array(array=w1333, index=w1332) -> (deleted portion=w1330:refnum<vi>, array with subset deleted=w1331:refnum<vi>[])  [unwired: 1 in]
              }
              frame "单选选项2" {
                n796 = Delete From Array(array=w1338, index=w1337) -> (deleted portion=w1335:refnum<vi>, array with subset deleted=w1336:refnum<vi>[])  [unwired: 1 in]
              }
            }
            n797 = local write "电压选择 4"(w1306) -> ()
            n798 = for {
              tunnel: u32 87470 -> [w1318]
              tunnel: w1312 -> [w1317] mode=indexing
              n799 = property class="Bool (严格)"(reference=w1317, "BoolText.TextColor"=w1318) -> ()  [unwired: 1 in, 2 out]
            }
            n800 = property class="Bool (严格)"(reference=w1314, "BoolText.TextColor"=u32 16777215) -> ()  [unwired: 1 in, 2 out]
          }
        }
        n801 = control-ref of="单选选项2 5"() -> (w1200:refnum<vi>)
        n802 = control-ref of="单选选项2 6"() -> (w1199:refnum<vi>)
        n803 = control-ref of="单选选项2 7"() -> (w1198:refnum<vi>)
        n804 = control-ref of="单选选项2 8"() -> (w1197:refnum<vi>)
        n805 = Not Equal?(x=w1193, y=w1192) -> (x != y?=→"状态":bool)
        n806 = Build Array(w1200, w1199, w1198, w1197) -> (w1201:refnum<vi>[])
        n807 = case shown="\"单选选项2 8\"" w1206 {
          selector: w1206 -> [w1345 w1350 w1355 w1360]
          tunnel: [w1344 w1349 w1354 w1359] -> w1203
          tunnel: [w1343 w1348 w1353 w1358] -> w1202
          tunnel: w1201 -> [w1342 w1347 w1352 w1357]
          tunnel: [enum32{"单体电压", "单体温度", "单体内阻", "单体SOC"}."单体电压" ("选项卡控件") enum32{"单体电压", "单体温度", "单体内阻", "单体SOC"}."单体温度" ("选项卡控件") enum32{"单体电压", "单体温度", "单体内阻", "单体SOC"}."单体内阻" ("选项卡控件") enum32{"单体电压", "单体温度", "单体内阻", "单体SOC"}."单体SOC" ("选项卡控件")] -> w1195
          frame "单选选项2 5" {
            n808 = Delete From Array(array=w1342, index=w1345) -> (deleted portion=w1343:refnum<vi>, array with subset deleted=w1344:refnum<vi>[])  [unwired: 1 in]
          }
          frame "单选选项2 6" {
            n809 = Delete From Array(array=w1347, index=w1350) -> (deleted portion=w1348:refnum<vi>, array with subset deleted=w1349:refnum<vi>[])  [unwired: 1 in]
          }
          frame "单选选项2 7" {
            n810 = Delete From Array(array=w1352, index=w1355) -> (deleted portion=w1353:refnum<vi>, array with subset deleted=w1354:refnum<vi>[])  [unwired: 1 in]
          }
          frame "单选选项2 8" {
            n811 = Delete From Array(array=w1357, index=w1360) -> (deleted portion=w1358:refnum<vi>, array with subset deleted=w1359:refnum<vi>[])  [unwired: 1 in]
          }
        }
        n812 = global read "EV05全局变量1.vi" "life"() -> (w1194:dbl)
        "Life:" <- w1194
        n813 = for {
          tunnel: w1203 -> [w1340] mode=indexing
          tunnel: u32 16777215 -> [w1339]
          n814 = property class="Bool (严格)"(reference=w1340, "BoolText.TextColor"=w1339) -> ()  [unwired: 1 in, 2 out]
        }
        n815 = property class="Bool (严格)"(reference=w1202, "BoolText.TextColor"=u32 8977151) -> ()  [unwired: 1 in, 2 out]
        n816 = local write "选项卡控件"(w1195) -> ()
      }
      event "刷新": Value Change {
        n817 = event-data() -> ("NewVal"=w1361:bool)  [unwired: 6 out]
        n818 = case shown="真" w1361 {
          frame False {
          }
          frame True {
            n819 = global write "单体信息全局.vi" "单体数据"(dbl[][] [[0.0, 0.0, 0.0, 0.0, 0.0, 0.0, 0.0, 0.0, 0.0, 0.0, 0.0, 0.0, 0.0, 0.0, 0.0, 0.0, 0.0, 0.0, 0.0, 0.0, 0.0, 0.0, 0.0, 0.0, 0.0, 0.0, 0.0, 0.0, 0.0, 0.0, 0.0, 0.0, 0.0, 0.0, 0.0, 0.0, 0.0, 0.0, 0.0, 0.0, 0.0, 0.0, 0.0, 0.0, 0.0, 0.0, 0.0, 0.0, 0.0, 0.0, 0.0, 0.0, 0.0, 0.0, 0.0, 0.0, 0.0, 0.0, 0.0, 0.0, 0.0], [0.0, 0.0, 0.0, 0.0, 0.0, 0.0, 0.0, 0.0, 0.0, 0.0, 0.0, 0.0, 0.0, 0.0, 0.0, 0.0, 0.0, 0.0, 0.0, 0.0, 0.0, 0.0, 0.0, 0.0, 0.0, 0.0, 0.0, 0.0, 0.0, 0.0, 0.0, 0.0, 0.0, 0.0, 0.0, 0.0, 0.0, 0.0, 0.0, 0.0, 0.0, 0.0, 0.0, 0.0, 0.0, 0.0, 0.0, 0.0, 0.0, 0.0, 0.0, 0.0, 0.0, 0.0, 0.0, 0.0, 0.0, 0.0, 0.0, 0.0, 0.0], [0.0, 0.0, 0.0, 0.0, 0.0, 0.0, 0.0, 0.0, 0.0, 0.0, 0.0, 0.0, 0.0, 0.0, 0.0, 0.0, 0.0, 0.0, 0.0, 0.0, 0.0, 0.0, 0.0, 0.0, 0.0, 0.0, 0.0, 0.0, 0.0, 0.0, 0.0, 0.0, 0.0, 0.0, 0.0, 0.0, 0.0, 0.0, 0.0, 0.0, 0.0, 0.0, 0.0, 0.0, 0.0, 0.0, 0.0, 0.0, 0.0, 0.0, 0.0, 0.0, 0.0, 0.0, 0.0, 0.0, 0.0, 0.0, 0.0, 0.0, 0.0], [0.0, 0.0, 0.0, 0.0, 0.0, 0.0, 0.0, 0.0, 0.0, 0.0, 0.0, 0.0, 0.0, 0.0, 0.0, 0.0, 0.0, 0.0, 0.0, 0.0, 0.0, 0.0, 0.0, 0.0, 0.0, 0.0, 0.0, 0.0, 0.0, 0.0, 0.0, 0.0, 0.0, 0.0, 0.0, 0.0, 0.0, 0.0, 0.0, 0.0, 0.0, 0.0, 0.0, 0.0, 0.0, 0.0, 0.0, 0.0, 0.0, 0.0, 0.0, 0.0, 0.0, 0.0, 0.0, 0.0, 0.0, 0.0, 0.0, 0.0, 0.0], [0.0, 0.0, 0.0, 0.0, 0.0, 0.0, 0.0, 0.0, 0.0, 0.0, 0.0, 0.0, 0.0, 0.0, 0.0, 0.0, 0.0, 0.0, 0.0, 0.0, 0.0, 0.0, 0.0, 0.0, 0.0, 0.0, 0.0, 0.0, 0.0, 0.0, 0.0, 0.0, 0.0, 0.0, 0.0, 0.0, 0.0, 0.0, 0.0, 0.0, 0.0, 0.0, 0.0, 0.0, 0.0, 0.0, 0.0, 0.0, 0.0, 0.0, 0.0, 0.0, 0.0, 0.0, 0.0, 0.0, 0.0, 0.0, 0.0, 0.0, 0.0], [0.0, 0.0, 0.0, 0.0, 0.0, 0.0, 0.0, 0.0, 0.0, 0.0, 0.0, 0.0, 0.0, 0.0, 0.0, 0.0, 0.0, 0.0, 0.0, 0.0, 0.0, 0.0, 0.0, 0.0, 0.0, 0.0, 0.0, 0.0, 0.0, 0.0, 0.0, 0.0, 0.0, 0.0, 0.0, 0.0, 0.0, 0.0, 0.0, 0.0, 0.0, 0.0, 0.0, 0.0, 0.0, 0.0, 0.0, 0.0, 0.0, 0.0, 0.0, 0.0, 0.0, 0.0, 0.0, 0.0, 0.0, 0.0, 0.0, 0.0, 0.0], [0.0, 0.0, 0.0, 0.0, 0.0, 0.0, 0.0, 0.0, 0.0, 0.0, 0.0, 0.0, 0.0, 0.0, 0.0, 0.0, 0.0, 0.0, 0.0, 0.0, 0.0, 0.0, 0.0, 0.0, 0.0, 0.0, 0.0, 0.0, 0.0, 0.0, 0.0, 0.0, 0.0, 0.0, 0.0, 0.0, 0.0, 0.0, 0.0, 0.0, 0.0, 0.0, 0.0, 0.0, 0.0, 0.0, 0.0, 0.0, 0.0, 0.0, 0.0, 0.0, 0.0, 0.0, 0.0, 0.0, 0.0, 0.0, 0.0, 0.0, 0.0], [0.0, 0.0, 0.0, 0.0, 0.0, 0.0, 0.0, 0.0, 0.0, 0.0, 0.0, 0.0, 0.0, 0.0, 0.0, 0.0, 0.0, 0.0, 0.0, 0.0, 0.0, 0.0, 0.0, 0.0, 0.0, 0.0, 0.0, 0.0, 0.0, 0.0, 0.0, 0.0, 0.0, 0.0, 0.0, 0.0, 0.0, 0.0, 0.0, 0.0, 0.0, 0.0, 0.0, 0.0, 0.0, 0.0, 0.0, 0.0, 0.0, 0.0, 0.0, 0.0, 0.0, 0.0, 0.0, 0.0, 0.0, 0.0, 0.0, 0.0, 0.0], [0.0, 0.0, 0.0, 0.0, 0.0, 0.0, 0.0, 0.0, 0.0, 0.0, 0.0, 0.0, 0.0, 0.0, 0.0, 0.0, 0.0, 0.0, 0.0, 0.0, 0.0, 0.0, 0.0, 0.0, 0.0, 0.0, 0.0, 0.0, 0.0, 0.0, 0.0, 0.0, 0.0, 0.0, 0.0, 0.0, 0.0, 0.0, 0.0, 0.0, 0.0, 0.0, 0.0, 0.0, 0.0, 0.0, 0.0, 0.0, 0.0, 0.0, 0.0, 0.0, 0.0, 0.0, 0.0, 0.0, 0.0, 0.0, 0.0, 0.0, 0.0], [0.0, 0.0, 0.0, 0.0, 0.0, 0.0, 0.0, 0.0, 0.0, 0.0, 0.0, 0.0, 0.0, 0.0, 0.0, 0.0, 0.0, 0.0, 0.0, 0.0, 0.0, 0.0, 0.0, 0.0, 0.0, 0.0, 0.0, 0.0, 0.0, 0.0, 0.0, 0.0, 0.0, 0.0, 0.0, 0.0, 0.0, 0.0, 0.0, 0.0, 0.0, 0.0, 0.0, 0.0, 0.0, 0.0, 0.0, 0.0, 0.0, 0.0, 0.0, 0.0, 0.0, 0.0, 0.0, 0.0, 0.0, 0.0, 0.0, 0.0, 0.0], [0.0, 0.0, 0.0, 0.0, 0.0, 0.0, 0.0, 0.0, 0.0, 0.0, 0.0, 0.0, 0.0, 0.0, 0.0, 0.0, 0.0, 0.0, 0.0, 0.0, 0.0, 0.0, 0.0, 0.0, 0.0, 0.0, 0.0, 0.0, 0.0, 0.0, 0.0, 0.0, 0.0, 0.0, 0.0, 0.0, 0.0, 0.0, 0.0, 0.0, 0.0, 0.0, 0.0, 0.0, 0.0, 0.0, 0.0, 0.0, 0.0, 0.0, 0.0, 0.0, 0.0, 0.0, 0.0, 0.0, 0.0, 0.0, 0.0, 0.0, 0.0], [0.0, 0.0, 0.0, 0.0, 0.0, 0.0, 0.0, 0.0, 0.0, 0.0, 0.0, 0.0, 0.0, 0.0, 0.0, 0.0, 0.0, 0.0, 0.0, 0.0, 0.0, 0.0, 0.0, 0.0, 0.0, 0.0, 0.0, 0.0, 0.0, 0.0, 0.0, 0.0, 0.0, 0.0, 0.0, 0.0, 0.0, 0.0, 0.0, 0.0, 0.0, 0.0, 0.0, 0.0, 0.0, 0.0, 0.0, 0.0, 0.0, 0.0, 0.0, 0.0, 0.0, 0.0, 0.0, 0.0, 0.0, 0.0, 0.0, 0.0, 0.0], [0.0, 0.0, 0.0, 0.0, 0.0, 0.0, 0.0, 0.0, 0.0, 0.0, 0.0, 0.0, 0.0, 0.0, 0.0, 0.0, 0.0, 0.0, 0.0, 0.0, 0.0, 0.0, 0.0, 0.0, 0.0, 0.0, 0.0, 0.0, 0.0, 0.0, 0.0, 0.0, 0.0, 0.0, 0.0, 0.0, 0.0, 0.0, 0.0, 0.0, 0.0, 0.0, 0.0, 0.0, 0.0, 0.0, 0.0, 0.0, 0.0, 0.0, 0.0, 0.0, 0.0, 0.0, 0.0, 0.0, 0.0, 0.0, 0.0, 0.0, 0.0], [0.0, 0.0, 0.0, 0.0, 0.0, 0.0, 0.0, 0.0, 0.0, 0.0, 0.0, 0.0, 0.0, 0.0, 0.0, 0.0, 0.0, 0.0, 0.0, 0.0, 0.0, 0.0, 0.0, 0.0, 0.0, 0.0, 0.0, 0.0, 0.0, 0.0, 0.0, 0.0, 0.0, 0.0, 0.0, 0.0, 0.0, 0.0, 0.0, 0.0, 0.0, 0.0, 0.0, 0.0, 0.0, 0.0, 0.0, 0.0, 0.0, 0.0, 0.0, 0.0, 0.0, 0.0, 0.0, 0.0, 0.0, 0.0, 0.0, 0.0, 0.0], [0.0, 0.0, 0.0, 0.0, 0.0, 0.0, 0.0, 0.0, 0.0, 0.0, 0.0, 0.0, 0.0, 0.0, 0.0, 0.0, 0.0, 0.0, 0.0, 0.0, 0.0, 0.0, 0.0, 0.0, 0.0, 0.0, 0.0, 0.0, 0.0, 0.0, 0.0, 0.0, 0.0, 0.0, 0.0, 0.0, 0.0, 0.0, 0.0, 0.0, 0.0, 0.0, 0.0, 0.0, 0.0, 0.0, 0.0, 0.0, 0.0, 0.0, 0.0, 0.0, 0.0, 0.0, 0.0, 0.0, 0.0, 0.0, 0.0, 0.0, 0.0], [0.0, 0.0, 0.0, 0.0, 0.0, 0.0, 0.0, 0.0, 0.0, 0.0, 0.0, 0.0, 0.0, 0.0, 0.0, 0.0, 0.0, 0.0, 0.0, 0.0, 0.0, 0.0, 0.0, 0.0, 0.0, 0.0, 0.0, 0.0, 0.0, 0.0, 0.0, 0.0, 0.0, 0.0, 0.0, 0.0, 0.0, 0.0, 0.0, 0.0, 0.0, 0.0, 0.0, 0.0, 0.0, 0.0, 0.0, 0.0, 0.0, 0.0, 0.0, 0.0, 0.0, 0.0, 0.0, 0.0, 0.0, 0.0, 0.0, 0.0, 0.0], [0.0, 0.0, 0.0, 0.0, 0.0, 0.0, 0.0, 0.0, 0.0, 0.0, 0.0, 0.0, 0.0, 0.0, 0.0, 0.0, 0.0, 0.0, 0.0, 0.0, 0.0, 0.0, 0.0, 0.0, 0.0, 0.0, 0.0, 0.0, 0.0, 0.0, 0.0, 0.0, 0.0, 0.0, 0.0, 0.0, 0.0, 0.0, 0.0, 0.0, 0.0, 0.0, 0.0, 0.0, 0.0, 0.0, 0.0, 0.0, 0.0, 0.0, 0.0, 0.0, 0.0, 0.0, 0.0, 0.0, 0.0, 0.0, 0.0, 0.0, 0.0], [0.0, 0.0, 0.0, 0.0, 0.0, 0.0, 0.0, 0.0, 0.0, 0.0, 0.0, 0.0, 0.0, 0.0, 0.0, 0.0, 0.0, 0.0, 0.0, 0.0, 0.0, 0.0, 0.0, 0.0, 0.0, 0.0, 0.0, 0.0, 0.0, 0.0, 0.0, 0.0, 0.0, 0.0, 0.0, 0.0, 0.0, 0.0, 0.0, 0.0, 0.0, 0.0, 0.0, 0.0, 0.0, 0.0, 0.0, 0.0, 0.0, 0.0, 0.0, 0.0, 0.0, 0.0, 0.0, 0.0, 0.0, 0.0, 0.0, 0.0, 0.0], [0.0, 0.0, 0.0, 0.0, 0.0, 0.0, 0.0, 0.0, 0.0, 0.0, 0.0, 0.0, 0.0, 0.0, 0.0, 0.0, 0.0, 0.0, 0.0, 0.0, 0.0, 0.0, 0.0, 0.0, 0.0, 0.0, 0.0, 0.0, 0.0, 0.0, 0.0, 0.0, 0.0, 0.0, 0.0, 0.0, 0.0, 0.0, 0.0, 0.0, 0.0, 0.0, 0.0, 0.0, 0.0, 0.0, 0.0, 0.0, 0.0, 0.0, 0.0, 0.0, 0.0, 0.0, 0.0, 0.0, 0.0, 0.0, 0.0, 0.0, 0.0], [0.0, 0.0, 0.0, 0.0, 0.0, 0.0, 0.0, 0.0, 0.0, 0.0, 0.0, 0.0, 0.0, 0.0, 0.0, 0.0, 0.0, 0.0, 0.0, 0.0, 0.0, 0.0, 0.0, 0.0, 0.0, 0.0, 0.0, 0.0, 0.0, 0.0, 0.0, 0.0, 0.0, 0.0, 0.0, 0.0, 0.0, 0.0, 0.0, 0.0, 0.0, 0.0, 0.0, 0.0, 0.0, 0.0, 0.0, 0.0, 0.0, 0.0, 0.0, 0.0, 0.0, 0.0, 0.0, 0.0, 0.0, 0.0, 0.0, 0.0, 0.0], [0.0, 0.0, 0.0, 0.0, 0.0, 0.0, 0.0, 0.0, 0.0, 0.0, 0.0, 0.0, 0.0, 0.0, 0.0, 0.0, 0.0, 0.0, 0.0, 0.0, 0.0, 0.0, 0.0, 0.0, 0.0, 0.0, 0.0, 0.0, 0.0, 0.0, 0.0, 0.0, 0.0, 0.0, 0.0, 0.0, 0.0, 0.0, 0.0, 0.0, 0.0, 0.0, 0.0, 0.0, 0.0, 0.0, 0.0, 0.0, 0.0, 0.0, 0.0, 0.0, 0.0, 0.0, 0.0, 0.0, 0.0, 0.0, 0.0, 0.0, 0.0], [0.0, 0.0, 0.0, 0.0, 0.0, 0.0, 0.0, 0.0, 0.0, 0.0, 0.0, 0.0, 0.0, 0.0, 0.0, 0.0, 0.0, 0.0, 0.0, 0.0, 0.0, 0.0, 0.0, 0.0, 0.0, 0.0, 0.0, 0.0, 0.0, 0.0, 0.0, 0.0, 0.0, 0.0, 0.0, 0.0, 0.0, 0.0, 0.0, 0.0, 0.0, 0.0, 0.0, 0.0, 0.0, 0.0, 0.0, 0.0, 0.0, 0.0, 0.0, 0.0, 0.0, 0.0, 0.0, 0.0, 0.0, 0.0, 0.0, 0.0, 0.0], [0.0, 0.0, 0.0, 0.0, 0.0, 0.0, 0.0, 0.0, 0.0, 0.0, 0.0, 0.0, 0.0, 0.0, 0.0, 0.0, 0.0, 0.0, 0.0, 0.0, 0.0, 0.0, 0.0, 0.0, 0.0, 0.0, 0.0, 0.0, 0.0, 0.0, 0.0, 0.0, 0.0, 0.0, 0.0, 0.0, 0.0, 0.0, 0.0, 0.0, 0.0, 0.0, 0.0, 0.0, 0.0, 0.0, 0.0, 0.0, 0.0, 0.0, 0.0, 0.0, 0.0, 0.0, 0.0, 0.0, 0.0, 0.0, 0.0, 0.0, 0.0], [0.0, 0.0, 0.0, 0.0, 0.0, 0.0, 0.0, 0.0, 0.0, 0.0, 0.0, 0.0, 0.0, 0.0, 0.0, 0.0, 0.0, 0.0, 0.0, 0.0, 0.0, 0.0, 0.0, 0.0, 0.0, 0.0, 0.0, 0.0, 0.0, 0.0, 0.0, 0.0, 0.0, 0.0, 0.0, 0.0, 0.0, 0.0, 0.0, 0.0, 0.0, 0.0, 0.0, 0.0, 0.0, 0.0, 0.0, 0.0, 0.0, 0.0, 0.0, 0.0, 0.0, 0.0, 0.0, 0.0, 0.0, 0.0, 0.0, 0.0, 0.0], [0.0, 0.0, 0.0, 0.0, 0.0, 0.0, 0.0, 0.0, 0.0, 0.0, 0.0, 0.0, 0.0, 0.0, 0.0, 0.0, 0.0, 0.0, 0.0, 0.0, 0.0, 0.0, 0.0, 0.0, 0.0, 0.0, 0.0, 0.0, 0.0, 0.0, 0.0, 0.0, 0.0, 0.0, 0.0, 0.0, 0.0, 0.0, 0.0, 0.0, 0.0, 0.0, 0.0, 0.0, 0.0, 0.0, 0.0, 0.0, 0.0, 0.0, 0.0, 0.0, 0.0, 0.0, 0.0, 0.0, 0.0, 0.0, 0.0, 0.0, 0.0], [0.0, 0.0, 0.0, 0.0, 0.0, 0.0, 0.0, 0.0, 0.0, 0.0, 0.0, 0.0, 0.0, 0.0, 0.0, 0.0, 0.0, 0.0, 0.0, 0.0, 0.0, 0.0, 0.0, 0.0, 0.0, 0.0, 0.0, 0.0, 0.0, 0.0, 0.0, 0.0, 0.0, 0.0, 0.0, 0.0, 0.0, 0.0, 0.0, 0.0, 0.0, 0.0, 0.0, 0.0, 0.0, 0.0, 0.0, 0.0, 0.0, 0.0, 0.0, 0.0, 0.0, 0.0, 0.0, 0.0, 0.0, 0.0, 0.0, 0.0, 0.0], [0.0, 0.0, 0.0, 0.0, 0.0, 0.0, 0.0, 0.0, 0.0, 0.0, 0.0, 0.0, 0.0, 0.0, 0.0, 0.0, 0.0, 0.0, 0.0, 0.0, 0.0, 0.0, 0.0, 0.0, 0.0, 0.0, 0.0, 0.0, 0.0, 0.0, 0.0, 0.0, 0.0, 0.0, 0.0, 0.0, 0.0, 0.0, 0.0, 0.0, 0.0, 0.0, 0.0, 0.0, 0.0, 0.0, 0.0, 0.0, 0.0, 0.0, 0.0, 0.0, 0.0, 0.0, 0.0, 0.0, 0.0, 0.0, 0.0, 0.0, 0.0], [0.0, 0.0, 0.0, 0.0, 0.0, 0.0, 0.0, 0.0, 0.0, 0.0, 0.0, 0.0, 0.0, 0.0, 0.0, 0.0, 0.0, 0.0, 0.0, 0.0, 0.0, 0.0, 0.0, 0.0, 0.0, 0.0, 0.0, 0.0, 0.0, 0.0, 0.0, 0.0, 0.0, 0.0, 0.0, 0.0, 0.0, 0.0, 0.0, 0.0, 0.0, 0.0, 0.0, 0.0, 0.0, 0.0, 0.0, 0.0, 0.0, 0.0, 0.0, 0.0, 0.0, 0.0, 0.0, 0.0, 0.0, 0.0, 0.0, 0.0, 0.0], [0.0, 0.0, 0.0, 0.0, 0.0, 0.0, 0.0, 0.0, 0.0, 0.0, 0.0, 0.0, 0.0, 0.0, 0.0, 0.0, 0.0, 0.0, 0.0, 0.0, 0.0, 0.0, 0.0, 0.0, 0.0, 0.0, 0.0, 0.0, 0.0, 0.0, 0.0, 0.0, 0.0, 0.0, 0.0, 0.0, 0.0, 0.0, 0.0, 0.0, 0.0, 0.0, 0.0, 0.0, 0.0, 0.0, 0.0, 0.0, 0.0, 0.0, 0.0, 0.0, 0.0, 0.0, 0.0, 0.0, 0.0, 0.0, 0.0, 0.0, 0.0], [0.0, 0.0, 0.0, 0.0, 0.0, 0.0, 0.0, 0.0, 0.0, 0.0, 0.0, 0.0, 0.0, 0.0, 0.0, 0.0, 0.0, 0.0, 0.0, 0.0, 0.0, 0.0, 0.0, 0.0, 0.0, 0.0, 0.0, 0.0, 0.0, 0.0, 0.0, 0.0, 0.0, 0.0, 0.0, 0.0, 0.0, 0.0, 0.0, 0.0, 0.0, 0.0, 0.0, 0.0, 0.0, 0.0, 0.0, 0.0, 0.0, 0.0, 0.0, 0.0, 0.0, 0.0, 0.0, 0.0, 0.0, 0.0, 0.0, 0.0, 0.0], [0.0, 0.0, 0.0, 0.0, 0.0, 0.0, 0.0, 0.0, 0.0, 0.0, 0.0, 0.0, 0.0, 0.0, 0.0, 0.0, 0.0, 0.0, 0.0, 0.0, 0.0, 0.0, 0.0, 0.0, 0.0, 0.0, 0.0, 0.0, 0.0, 0.0, 0.0, 0.0, 0.0, 0.0, 0.0, 0.0, 0.0, 0.0, 0.0, 0.0, 0.0, 0.0, 0.0, 0.0, 0.0, 0.0, 0.0, 0.0, 0.0, 0.0, 0.0, 0.0, 0.0, 0.0, 0.0, 0.0, 0.0, 0.0, 0.0, 0.0, 0.0]] ("单体数据")) -> ()
            n820 = global write "单体信息全局.vi" "温度数据"(u8[][] [[0, 0, 0, 0, 0, 0, 0, 0, 0, 0, 0], [0, 0, 0, 0, 0, 0, 0, 0, 0, 0, 0], [0, 0, 0, 0, 0, 0, 0, 0, 0, 0, 0], [0, 0, 0, 0, 0, 0, 0, 0, 0, 0, 0], [0, 0, 0, 0, 0, 0, 0, 0, 0, 0, 0], [0, 0, 0, 0, 0, 0, 0, 0, 0, 0, 0], [0, 0, 0, 0, 0, 0, 0, 0, 0, 0, 0], [0, 0, 0, 0, 0, 0, 0, 0, 0, 0, 0], [0, 0, 0, 0, 0, 0, 0, 0, 0, 0, 0], [0, 0, 0, 0, 0, 0, 0, 0, 0, 0, 0], [0, 0, 0, 0, 0, 0, 0, 0, 0, 0, 0], [0, 0, 0, 0, 0, 0, 0, 0, 0, 0, 0], [0, 0, 0, 0, 0, 0, 0, 0, 0, 0, 0], [0, 0, 0, 0, 0, 0, 0, 0, 0, 0, 0], [0, 0, 0, 0, 0, 0, 0, 0, 0, 0, 0], [0, 0, 0, 0, 0, 0, 0, 0, 0, 0, 0], [0, 0, 0, 0, 0, 0, 0, 0, 0, 0, 0], [0, 0, 0, 0, 0, 0, 0, 0, 0, 0, 0], [0, 0, 0, 0, 0, 0, 0, 0, 0, 0, 0], [0, 0, 0, 0, 0, 0, 0, 0, 0, 0, 0], [0, 0, 0, 0, 0, 0, 0, 0, 0, 0, 0], [0, 0, 0, 0, 0, 0, 0, 0, 0, 0, 0], [0, 0, 0, 0, 0, 0, 0, 0, 0, 0, 0], [0, 0, 0, 0, 0, 0, 0, 0, 0, 0, 0], [0, 0, 0, 0, 0, 0, 0, 0, 0, 0, 0], [0, 0, 0, 0, 0, 0, 0, 0, 0, 0, 0], [0, 0, 0, 0, 0, 0, 0, 0, 0, 0, 0], [0, 0, 0, 0, 0, 0, 0, 0, 0, 0, 0], [0, 0, 0, 0, 0, 0, 0, 0, 0, 0, 0], [0, 0, 0, 0, 0, 0, 0, 0, 0, 0, 0], [0, 0, 0, 0, 0, 0, 0, 0, 0, 0, 0]] ("温度数据")) -> ()
            n821 = global write "电池信息全局变量.vi" "允许保存数据"(FALSE ("允许保存数据")) -> ()
            n822 = global write "电池信息全局变量.vi" "刷新计数"(0.0 ("刷新计数")) -> ()
          }
        }
      }
      event "停止": Value Change {
        n823 = event-data() -> ("NewVal"=w1367:bool)  [unwired: 6 out]
        n824 = disable-structure shown="启用" {
          disable-tunnel: w1367 -> [_ w1372]
          frame Enabled {
            n825 = property class="VI"("FP.State"=T17."Hidden" ("前面板窗口:状态")) -> (reference out=w1369:refnum<vi>, error out=w1368:errorcluster)  [unwired: 2 in]
            n826 = property class="VI"(reference=w1369, error in=w1368, "Front Panel.Open"=FALSE ("前面板窗口:打开")) -> ()  [unwired: 2 out]
          }
          frame Disabled {
            n827 = Stop(stop? (T)=w1372) -> ()
          }
        }
        n828 = local write "停止"(TRUE ("停止")) -> ()
      }
      event Panel Close? {
        w1373 = TRUE ("停止")
        n829 = event-data() -> ()  [unwired: 5 out]
        n830 = disable-structure shown="启用" {
          disable-tunnel: w1373 -> [_ w1379]
          frame Enabled {
            n831 = property class="VI"("FP.State"=T17."Hidden" ("前面板窗口:状态")) -> (reference out=w1376:refnum<vi>, error out=w1375:errorcluster)  [unwired: 2 in]
            n832 = property class="VI"(reference=w1376, error in=w1375, "Front Panel.Open"=FALSE ("前面板窗口:打开")) -> ()  [unwired: 2 out]
          }
          frame Disabled {
            n833 = Stop(stop? (T)=w1379) -> ()
          }
        }
        n834 = local write "停止"(w1373) -> ()
        n835 = event-data("Discard?"=FALSE ("放弃？")) -> ()  [unwired: 1 in, 1 out]
      }
    }
    n836 = local write "状态"(FALSE ("状态")) -> ()
  }
  n837 = disable-structure shown="启用" {
    frame Disabled {
      n838 = while {
        stop <- w1381 stop-if-true
        n839 = local read "停止"() -> (w1381:bool)
        n840 = Wait Until Next ms Multiple(millisecond multiple=u32 500 ("毫秒倍数")) -> ()  [unwired: 1 out]
        n841 = case shown="真" "213" {
          frame False {
          }
          frame True {
            n842 = local read "选项卡控件"() -> (w1384:enum32{"单体电压", "单体温度", "单体内阻", "单体SOC"})
            n843 = local write "213"(FALSE ("213")) -> ()
            n844 = case shown="\"单体温度\"" w1384 {
              frame "单体电压", Default {
                n845 = for {
                  N: 300 -> [_]
                  tunnel: [TRUE] -> w1386 mode=indexing
                }
                n846 = for {
                  N: 16 -> [_]
                  tunnel: w1386 -> [w1393]
                  i -> [w1394]
                  w1391 = 12 ("y")
                  n847 = Multiply(x=w1394, y=w1391) -> (x*y=w1392:i32)
                  n848 = Array Subset(array=w1393, index=w1392, length=w1391) -> (w1390:bool[])
                  n849 = case shown="0" w1394 {
                    tunnel: w1390 -> [w1396 w1406 w1417 w1428 w1439 w1450 w1461 w1472 w1483 w1494 w1505 w1516 w1527 w1538 w1549 w1560 _]
                    frame 0 {
                      n850 = control-ref of="1 102"() -> (w1398:refnum<vi>)
                      n851 = property class="Clust (严格)"(reference=w1398) -> ("Controls[]"=w1397:refnum<vi>[])  [unwired: 1 in, 2 out]
                      n852 = for {
                        N: 12 -> [_]
                        tunnel: w1397 -> [w1404] mode=indexing
                        tunnel: w1396 -> [w1405]
                        i -> [w1402]
                        n853 = Index Array(array=w1405, index=w1402) -> (element=w1403:bool)
                        n854 = Select(t=0, s=w1403, f=2) -> (s? t:f=w1401:i32)
                        n855 = property class="Ctl"(reference=w1404, "DisabledEnum"=w1401) -> ()  [unwired: 1 in, 2 out]
                      }
                    }
                    frame 1 {
                      n856 = control-ref of="1 3"() -> (w1409:refnum<vi>)
                      n857 = property class="Clust (严格)"(reference=w1409) -> ("Controls[]"=w1407:refnum<vi>[])  [unwired: 1 in, 2 out]
                      n858 = for {
                        N: 12 -> [_]
                        tunnel: w1407 -> [w1415] mode=indexing
                        tunnel: w1406 -> [w1416]
                        i -> [w1413]
                        n859 = Index Array(array=w1416, index=w1413) -> (element=w1414:bool)
                        n860 = Select(t=0, s=w1414, f=2) -> (s? t:f=w1412:i32)
                        n861 = property class="Ctl"(reference=w1415, "DisabledEnum"=w1412) -> ()  [unwired: 1 in, 2 out]
                      }
                    }
                    frame 2 {
                      n862 = control-ref of="1 4"() -> (w1420:refnum<vi>)
                      n863 = property class="Clust (严格)"(reference=w1420) -> ("Controls[]"=w1418:refnum<vi>[])  [unwired: 1 in, 2 out]
                      n864 = for {
                        N: 12 -> [_]
                        tunnel: w1418 -> [w1426] mode=indexing
                        tunnel: w1417 -> [w1427]
                        i -> [w1424]
                        n865 = Index Array(array=w1427, index=w1424) -> (element=w1425:bool)
                        n866 = Select(t=0, s=w1425, f=2) -> (s? t:f=w1423:i32)
                        n867 = property class="Ctl"(reference=w1426, "DisabledEnum"=w1423) -> ()  [unwired: 1 in, 2 out]
                      }
                    }
                    frame 3 {
                      n868 = control-ref of="1 6"() -> (w1431:refnum<vi>)
                      n869 = property class="Clust (严格)"(reference=w1431) -> ("Controls[]"=w1429:refnum<vi>[])  [unwired: 1 in, 2 out]
                      n870 = for {
                        N: 12 -> [_]
                        tunnel: w1429 -> [w1437] mode=indexing
                        tunnel: w1428 -> [w1438]
                        i -> [w1435]
                        n871 = Index Array(array=w1438, index=w1435) -> (element=w1436:bool)
                        n872 = Select(t=0, s=w1436, f=2) -> (s? t:f=w1434:i32)
                        n873 = property class="Ctl"(reference=w1437, "DisabledEnum"=w1434) -> ()  [unwired: 1 in, 2 out]
                      }
                    }
                    frame 4 {
                      n874 = control-ref of="1 7"() -> (w1442:refnum<vi>)
                      n875 = property class="Clust (严格)"(reference=w1442) -> ("Controls[]"=w1440:refnum<vi>[])  [unwired: 1 in, 2 out]
                      n876 = for {
                        N: 12 -> [_]
                        tunnel: w1440 -> [w1448] mode=indexing
                        tunnel: w1439 -> [w1449]
                        i -> [w1446]
                        n877 = Index Array(array=w1449, index=w1446) -> (element=w1447:bool)
                        n878 = Select(t=0, s=w1447, f=2) -> (s? t:f=w1445:i32)
                        n879 = property class="Ctl"(reference=w1448, "DisabledEnum"=w1445) -> ()  [unwired: 1 in, 2 out]
                      }
                    }
                    frame 5 {
                      n880 = control-ref of="1 8"() -> (w1453:refnum<vi>)
                      n881 = property class="Clust (严格)"(reference=w1453) -> ("Controls[]"=w1451:refnum<vi>[])  [unwired: 1 in, 2 out]
                      n882 = for {
                        N: 12 -> [_]
                        tunnel: w1451 -> [w1459] mode=indexing
                        tunnel: w1450 -> [w1460]
                        i -> [w1457]
                        n883 = Index Array(array=w1460, index=w1457) -> (element=w1458:bool)
                        n884 = Select(t=0, s=w1458, f=2) -> (s? t:f=w1456:i32)
                        n885 = property class="Ctl"(reference=w1459, "DisabledEnum"=w1456) -> ()  [unwired: 1 in, 2 out]
                      }
                    }
                    frame 6 {
                      n886 = control-ref of="1 9"() -> (w1464:refnum<vi>)
                      n887 = property class="Clust (严格)"(reference=w1464) -> ("Controls[]"=w1462:refnum<vi>[])  [unwired: 1 in, 2 out]
                      n888 = for {
                        N: 12 -> [_]
                        tunnel: w1462 -> [w1470] mode=indexing
                        tunnel: w1461 -> [w1471]
                        i -> [w1468]
                        n889 = Index Array(array=w1471, index=w1468) -> (element=w1469:bool)
                        n890 = Select(t=0, s=w1469, f=2) -> (s? t:f=w1467:i32)
                        n891 = property class="Ctl"(reference=w1470, "DisabledEnum"=w1467) -> ()  [unwired: 1 in, 2 out]
                      }
                    }
                    frame 7 {
                      n892 = control-ref of="1 10"() -> (w1475:refnum<vi>)
                      n893 = property class="Clust (严格)"(reference=w1475) -> ("Controls[]"=w1473:refnum<vi>[])  [unwired: 1 in, 2 out]
                      n894 = for {
                        N: 12 -> [_]
                        tunnel: w1473 -> [w1481] mode=indexing
                        tunnel: w1472 -> [w1482]
                        i -> [w1479]
                        n895 = Index Array(array=w1482, index=w1479) -> (element=w1480:bool)
                        n896 = Select(t=0, s=w1480, f=2) -> (s? t:f=w1478:i32)
                        n897 = property class="Ctl"(reference=w1481, "DisabledEnum"=w1478) -> ()  [unwired: 1 in, 2 out]
                      }
                    }
                    frame 8 {
                      n898 = control-ref of="1 26"() -> (w1486:refnum<vi>)
                      n899 = property class="Clust (严格)"(reference=w1486) -> ("Controls[]"=w1484:refnum<vi>[])  [unwired: 1 in, 2 out]
                      n900 = for {
                        N: 12 -> [_]
                        tunnel: w1484 -> [w1492] mode=indexing
                        tunnel: w1483 -> [w1493]
                        i -> [w1490]
                        n901 = Index Array(array=w1493, index=w1490) -> (element=w1491:bool)
                        n902 = Select(t=0, s=w1491, f=2) -> (s? t:f=w1489:i32)
                        n903 = property class="Ctl"(reference=w1492, "DisabledEnum"=w1489) -> ()  [unwired: 1 in, 2 out]
                      }
                    }
                    frame 9 {
                      n904 = control-ref of="1 27"() -> (w1497:refnum<vi>)
                      n905 = property class="Clust (严格)"(reference=w1497) -> ("Controls[]"=w1495:refnum<vi>[])  [unwired: 1 in, 2 out]
                      n906 = for {
                        N: 12 -> [_]
                        tunnel: w1495 -> [w1503] mode=indexing
                        tunnel: w1494 -> [w1504]
                        i -> [w1501]
                        n907 = Index Array(array=w1504, index=w1501) -> (element=w1502:bool)
                        n908 = Select(t=0, s=w1502, f=2) -> (s? t:f=w1500:i32)
                        n909 = property class="Ctl"(reference=w1503, "DisabledEnum"=w1500) -> ()  [unwired: 1 in, 2 out]
                      }
                    }
                    frame 10 {
                      n910 = control-ref of="1 28"() -> (w1508:refnum<vi>)
                      n911 = property class="Clust (严格)"(reference=w1508) -> ("Controls[]"=w1506:refnum<vi>[])  [unwired: 1 in, 2 out]
                      n912 = for {
                        N: 12 -> [_]
                        tunnel: w1506 -> [w1514] mode=indexing
                        tunnel: w1505 -> [w1515]
                        i -> [w1512]
                        n913 = Index Array(array=w1515, index=w1512) -> (element=w1513:bool)
                        n914 = Select(t=0, s=w1513, f=2) -> (s? t:f=w1511:i32)
                        n915 = property class="Ctl"(reference=w1514, "DisabledEnum"=w1511) -> ()  [unwired: 1 in, 2 out]
                      }
                    }
                    frame 11 {
                      n916 = control-ref of="1 29"() -> (w1519:refnum<vi>)
                      n917 = property class="Clust (严格)"(reference=w1519) -> ("Controls[]"=w1517:refnum<vi>[])  [unwired: 1 in, 2 out]
                      n918 = for {
                        N: 12 -> [_]
                        tunnel: w1517 -> [w1525] mode=indexing
                        tunnel: w1516 -> [w1526]
                        i -> [w1523]
                        n919 = Index Array(array=w1526, index=w1523) -> (element=w1524:bool)
                        n920 = Select(t=0, s=w1524, f=2) -> (s? t:f=w1522:i32)
                        n921 = property class="Ctl"(reference=w1525, "DisabledEnum"=w1522) -> ()  [unwired: 1 in, 2 out]
                      }
                    }
                    frame 12 {
                      n922 = control-ref of="1 30"() -> (w1530:refnum<vi>)
                      n923 = property class="Clust (严格)"(reference=w1530) -> ("Controls[]"=w1528:refnum<vi>[])  [unwired: 1 in, 2 out]
                      n924 = for {
                        N: 12 -> [_]
                        tunnel: w1528 -> [w1536] mode=indexing
                        tunnel: w1527 -> [w1537]
                        i -> [w1534]
                        n925 = Index Array(array=w1537, index=w1534) -> (element=w1535:bool)
                        n926 = Select(t=0, s=w1535, f=2) -> (s? t:f=w1533:i32)
                        n927 = property class="Ctl"(reference=w1536, "DisabledEnum"=w1533) -> ()  [unwired: 1 in, 2 out]
                      }
                    }
                    frame 13 {
                      n928 = control-ref of="1 31"() -> (w1541:refnum<vi>)
                      n929 = property class="Clust (严格)"(reference=w1541) -> ("Controls[]"=w1539:refnum<vi>[])  [unwired: 1 in, 2 out]
                      n930 = for {
                        N: 12 -> [_]
                        tunnel: w1539 -> [w1547] mode=indexing
                        tunnel: w1538 -> [w1548]
                        i -> [w1545]
                        n931 = Index Array(array=w1548, index=w1545) -> (element=w1546:bool)
                        n932 = Select(t=0, s=w1546, f=2) -> (s? t:f=w1544:i32)
                        n933 = property class="Ctl"(reference=w1547, "DisabledEnum"=w1544) -> ()  [unwired: 1 in, 2 out]
                      }
                    }
                    frame 14 {
                      n934 = control-ref of="1 32"() -> (w1552:refnum<vi>)
                      n935 = property class="Clust (严格)"(reference=w1552) -> ("Controls[]"=w1550:refnum<vi>[])  [unwired: 1 in, 2 out]
                      n936 = for {
                        N: 12 -> [_]
                        tunnel: w1550 -> [w1558] mode=indexing
                        tunnel: w1549 -> [w1559]
                        i -> [w1556]
                        n937 = Index Array(array=w1559, index=w1556) -> (element=w1557:bool)
                        n938 = Select(t=0, s=w1557, f=2) -> (s? t:f=w1555:i32)
                        n939 = property class="Ctl"(reference=w1558, "DisabledEnum"=w1555) -> ()  [unwired: 1 in, 2 out]
                      }
                    }
                    frame 15 {
                      n940 = control-ref of="1 33"() -> (w1563:refnum<vi>)
                      n941 = property class="Clust (严格)"(reference=w1563) -> ("Controls[]"=w1561:refnum<vi>[])  [unwired: 1 in, 2 out]
                      n942 = for {
                        N: 12 -> [_]
                        tunnel: w1561 -> [w1569] mode=indexing
                        tunnel: w1560 -> [w1570]
                        i -> [w1567]
                        n943 = Index Array(array=w1570, index=w1567) -> (element=w1568:bool)
                        n944 = Select(t=0, s=w1568, f=2) -> (s? t:f=w1566:i32)
                        n945 = property class="Ctl"(reference=w1569, "DisabledEnum"=w1566) -> ()  [unwired: 1 in, 2 out]
                      }
                    }
                    frame 99, Default {
                    }
                  }
                }
                n946 = for {
                  N: 9 -> [_]
                  tunnel: w1386 -> [w1576]
                  i -> [w1577]
                  w1574 = 12 ("y")
                  n947 = Add(x=16, y=w1577) -> (x+y=w1572:i32)
                  n948 = Multiply(x=w1572, y=w1574) -> (x*y=w1575:i32)
                  n949 = Array Subset(array=w1576, index=w1575, length=w1574) -> (w1573:bool[])
                  n950 = case shown="8" w1577 {
                    tunnel: w1573 -> [w1578 w1589 w1600 w1611 w1622 w1633 w1644 w1655 w1666 _]
                    frame 0 {
                      n951 = control-ref of="1 18"() -> (w1581:refnum<vi>)
                      n952 = property class="Clust (严格)"(reference=w1581) -> ("Controls[]"=w1579:refnum<vi>[])  [unwired: 1 in, 2 out]
                      n953 = for {
                        N: 12 -> [_]
                        tunnel: w1579 -> [w1587] mode=indexing
                        tunnel: w1578 -> [w1588]
                        i -> [w1585]
                        n954 = Index Array(array=w1588, index=w1585) -> (element=w1586:bool)
                        n955 = Select(t=0, s=w1586, f=2) -> (s? t:f=w1584:i32)
                        n956 = property class="Ctl"(reference=w1587, "DisabledEnum"=w1584) -> ()  [unwired: 1 in, 2 out]
                      }
                    }
                    frame 1 {
                      n957 = control-ref of="1 19"() -> (w1592:refnum<vi>)
                      n958 = property class="Clust (严格)"(reference=w1592) -> ("Controls[]"=w1590:refnum<vi>[])  [unwired: 1 in, 2 out]
                      n959 = for {
                        N: 12 -> [_]
                        tunnel: w1590 -> [w1598] mode=indexing
                        tunnel: w1589 -> [w1599]
                        i -> [w1596]
                        n960 = Index Array(array=w1599, index=w1596) -> (element=w1597:bool)
                        n961 = Select(t=0, s=w1597, f=2) -> (s? t:f=w1595:i32)
                        n962 = property class="Ctl"(reference=w1598, "DisabledEnum"=w1595) -> ()  [unwired: 1 in, 2 out]
                      }
                    }
                    frame 2 {
                      n963 = control-ref of="1 20"() -> (w1603:refnum<vi>)
                      n964 = property class="Clust (严格)"(reference=w1603) -> ("Controls[]"=w1601:refnum<vi>[])  [unwired: 1 in, 2 out]
                      n965 = for {
                        N: 12 -> [_]
                        tunnel: w1601 -> [w1609] mode=indexing
                        tunnel: w1600 -> [w1610]
                        i -> [w1607]
                        n966 = Index Array(array=w1610, index=w1607) -> (element=w1608:bool)
                        n967 = Select(t=0, s=w1608, f=2) -> (s? t:f=w1606:i32)
                        n968 = property class="Ctl"(reference=w1609, "DisabledEnum"=w1606) -> ()  [unwired: 1 in, 2 out]
                      }
                    }
                    frame 3 {
                      n969 = control-ref of="1 21"() -> (w1614:refnum<vi>)
                      n970 = property class="Clust (严格)"(reference=w1614) -> ("Controls[]"=w1612:refnum<vi>[])  [unwired: 1 in, 2 out]
                      n971 = for {
                        N: 12 -> [_]
                        tunnel: w1612 -> [w1620] mode=indexing
                        tunnel: w1611 -> [w1621]
                        i -> [w1618]
                        n972 = Index Array(array=w1621, index=w1618) -> (element=w1619:bool)
                        n973 = Select(t=0, s=w1619, f=2) -> (s? t:f=w1617:i32)
                        n974 = property class="Ctl"(reference=w1620, "DisabledEnum"=w1617) -> ()  [unwired: 1 in, 2 out]
                      }
                    }
                    frame 4 {
                      n975 = control-ref of="1 22"() -> (w1625:refnum<vi>)
                      n976 = property class="Clust (严格)"(reference=w1625) -> ("Controls[]"=w1623:refnum<vi>[])  [unwired: 1 in, 2 out]
                      n977 = for {
                        N: 12 -> [_]
                        tunnel: w1623 -> [w1631] mode=indexing
                        tunnel: w1622 -> [w1632]
                        i -> [w1629]
                        n978 = Index Array(array=w1632, index=w1629) -> (element=w1630:bool)
                        n979 = Select(t=0, s=w1630, f=2) -> (s? t:f=w1628:i32)
                        n980 = property class="Ctl"(reference=w1631, "DisabledEnum"=w1628) -> ()  [unwired: 1 in, 2 out]
                      }
                    }
                    frame 5 {
                      n981 = control-ref of="1 23"() -> (w1636:refnum<vi>)
                      n982 = property class="Clust (严格)"(reference=w1636) -> ("Controls[]"=w1634:refnum<vi>[])  [unwired: 1 in, 2 out]
                      n983 = for {
                        N: 12 -> [_]
                        tunnel: w1634 -> [w1642] mode=indexing
                        tunnel: w1633 -> [w1643]
                        i -> [w1640]
                        n984 = Index Array(array=w1643, index=w1640) -> (element=w1641:bool)
                        n985 = Select(t=0, s=w1641, f=2) -> (s? t:f=w1639:i32)
                        n986 = property class="Ctl"(reference=w1642, "DisabledEnum"=w1639) -> ()  [unwired: 1 in, 2 out]
                      }
                    }
                    frame 6 {
                      n987 = control-ref of="1 24"() -> (w1647:refnum<vi>)
                      n988 = property class="Clust (严格)"(reference=w1647) -> ("Controls[]"=w1645:refnum<vi>[])  [unwired: 1 in, 2 out]
                      n989 = for {
                        N: 12 -> [_]
                        tunnel: w1645 -> [w1653] mode=indexing
                        tunnel: w1644 -> [w1654]
                        i -> [w1651]
                        n990 = Index Array(array=w1654, index=w1651) -> (element=w1652:bool)
                        n991 = Select(t=0, s=w1652, f=2) -> (s? t:f=w1650:i32)
                        n992 = property class="Ctl"(reference=w1653, "DisabledEnum"=w1650) -> ()  [unwired: 1 in, 2 out]
                      }
                    }
                    frame 7 {
                      n993 = control-ref of="1 25"() -> (w1658:refnum<vi>)
                      n994 = property class="Clust (严格)"(reference=w1658) -> ("Controls[]"=w1656:refnum<vi>[])  [unwired: 1 in, 2 out]
                      n995 = for {
                        N: 12 -> [_]
                        tunnel: w1656 -> [w1664] mode=indexing
                        tunnel: w1655 -> [w1665]
                        i -> [w1662]
                        n996 = Index Array(array=w1665, index=w1662) -> (element=w1663:bool)
                        n997 = Select(t=0, s=w1663, f=2) -> (s? t:f=w1661:i32)
                        n998 = property class="Ctl"(reference=w1664, "DisabledEnum"=w1661) -> ()  [unwired: 1 in, 2 out]
                      }
                    }
                    frame 8 {
                      n999 = control-ref of="1 5"() -> (w1669:refnum<vi>)
                      n1000 = property class="Clust (严格)"(reference=w1669) -> ("Controls[]"=w1667:refnum<vi>[])  [unwired: 1 in, 2 out]
                      n1001 = for {
                        N: 12 -> [_]
                        tunnel: w1667 -> [w1675] mode=indexing
                        tunnel: w1666 -> [w1676]
                        i -> [w1673]
                        n1002 = Index Array(array=w1676, index=w1673) -> (element=w1674:bool)
                        n1003 = Select(t=0, s=w1674, f=2) -> (s? t:f=w1672:i32)
                        n1004 = property class="Ctl"(reference=w1675, "DisabledEnum"=w1672) -> ()  [unwired: 1 in, 2 out]
                      }
                    }
                    frame 99, Default {
                    }
                  }
                }
              }
              frame "单体温度" {
                n1005 = for {
                  N: 300 -> [_]
                  tunnel: [TRUE] -> w1678 mode=indexing
                }
                n1006 = for {
                  N: 9 -> [_]
                  tunnel: w1678 -> [w1868]
                  i -> [w1869]
                  w1866 = 12 ("y")
                  n1007 = Add(x=16, y=w1869) -> (x+y=w1864:i32)
                  n1008 = Multiply(x=w1864, y=w1866) -> (x*y=w1867:i32)
                  n1009 = Array Subset(array=w1868, index=w1867, length=w1866) -> (w1865:bool[])
                  n1010 = case shown="0" w1869 {
                    tunnel: w1865 -> [w1870 w1881 w1892 w1903 w1914 w1925 w1936 w1947 w1958 _]
                    frame 0 {
                      n1011 = control-ref of="1 18"() -> (w1873:refnum<vi>)
                      n1012 = property class="Clust (严格)"(reference=w1873) -> ("Controls[]"=w1871:refnum<vi>[])  [unwired: 1 in, 2 out]
                      n1013 = for {
                        N: 12 -> [_]
                        tunnel: w1871 -> [w1879] mode=indexing
                        tunnel: w1870 -> [w1880]
                        i -> [w1877]
                        n1014 = Index Array(array=w1880, index=w1877) -> (element=w1878:bool)
                        n1015 = Select(t=0, s=w1878, f=2) -> (s? t:f=w1876:i32)
                        n1016 = property class="Ctl"(reference=w1879, "DisabledEnum"=w1876) -> ()  [unwired: 1 in, 2 out]
                      }
                    }
                    frame 1 {
                      n1017 = control-ref of="1 19"() -> (w1884:refnum<vi>)
                      n1018 = property class="Clust (严格)"(reference=w1884) -> ("Controls[]"=w1882:refnum<vi>[])  [unwired: 1 in, 2 out]
                      n1019 = for {
                        N: 12 -> [_]
                        tunnel: w1882 -> [w1890] mode=indexing
                        tunnel: w1881 -> [w1891]
                        i -> [w1888]
                        n1020 = Index Array(array=w1891, index=w1888) -> (element=w1889:bool)
                        n1021 = Select(t=0, s=w1889, f=2) -> (s? t:f=w1887:i32)
                        n1022 = property class="Ctl"(reference=w1890, "DisabledEnum"=w1887) -> ()  [unwired: 1 in, 2 out]
                      }
                    }
                    frame 2 {
                      n1023 = control-ref of="1 20"() -> (w1895:refnum<vi>)
                      n1024 = property class="Clust (严格)"(reference=w1895) -> ("Controls[]"=w1893:refnum<vi>[])  [unwired: 1 in, 2 out]
                      n1025 = for {
                        N: 12 -> [_]
                        tunnel: w1893 -> [w1901] mode=indexing
                        tunnel: w1892 -> [w1902]
                        i -> [w1899]
                        n1026 = Index Array(array=w1902, index=w1899) -> (element=w1900:bool)
                        n1027 = Select(t=0, s=w1900, f=2) -> (s? t:f=w1898:i32)
                        n1028 = property class="Ctl"(reference=w1901, "DisabledEnum"=w1898) -> ()  [unwired: 1 in, 2 out]
                      }
                    }
                    frame 3 {
                      n1029 = control-ref of="1 21"() -> (w1906:refnum<vi>)
                      n1030 = property class="Clust (严格)"(reference=w1906) -> ("Controls[]"=w1904:refnum<vi>[])  [unwired: 1 in, 2 out]
                      n1031 = for {
                        N: 12 -> [_]
                        tunnel: w1904 -> [w1912] mode=indexing
                        tunnel: w1903 -> [w1913]
                        i -> [w1910]
                        n1032 = Index Array(array=w1913, index=w1910) -> (element=w1911:bool)
                        n1033 = Select(t=0, s=w1911, f=2) -> (s? t:f=w1909:i32)
                        n1034 = property class="Ctl"(reference=w1912, "DisabledEnum"=w1909) -> ()  [unwired: 1 in, 2 out]
                      }
                    }
                    frame 4 {
                      n1035 = control-ref of="1 22"() -> (w1917:refnum<vi>)
                      n1036 = property class="Clust (严格)"(reference=w1917) -> ("Controls[]"=w1915:refnum<vi>[])  [unwired: 1 in, 2 out]
                      n1037 = for {
                        N: 12 -> [_]
                        tunnel: w1915 -> [w1923] mode=indexing
                        tunnel: w1914 -> [w1924]
                        i -> [w1921]
                        n1038 = Index Array(array=w1924, index=w1921) -> (element=w1922:bool)
                        n1039 = Select(t=0, s=w1922, f=2) -> (s? t:f=w1920:i32)
                        n1040 = property class="Ctl"(reference=w1923, "DisabledEnum"=w1920) -> ()  [unwired: 1 in, 2 out]
                      }
                    }
                    frame 5 {
                      n1041 = control-ref of="1 23"() -> (w1928:refnum<vi>)
                      n1042 = property class="Clust (严格)"(reference=w1928) -> ("Controls[]"=w1926:refnum<vi>[])  [unwired: 1 in, 2 out]
                      n1043 = for {
                        N: 12 -> [_]
                        tunnel: w1926 -> [w1934] mode=indexing
                        tunnel: w1925 -> [w1935]
                        i -> [w1932]
                        n1044 = Index Array(array=w1935, index=w1932) -> (element=w1933:bool)
                        n1045 = Select(t=0, s=w1933, f=2) -> (s? t:f=w1931:i32)
                        n1046 = property class="Ctl"(reference=w1934, "DisabledEnum"=w1931) -> ()  [unwired: 1 in, 2 out]
                      }
                    }
                    frame 6 {
                      n1047 = control-ref of="1 24"() -> (w1939:refnum<vi>)
                      n1048 = property class="Clust (严格)"(reference=w1939) -> ("Controls[]"=w1937:refnum<vi>[])  [unwired: 1 in, 2 out]
                      n1049 = for {
                        N: 12 -> [_]
                        tunnel: w1937 -> [w1945] mode=indexing
                        tunnel: w1936 -> [w1946]
                        i -> [w1943]
                        n1050 = Index Array(array=w1946, index=w1943) -> (element=w1944:bool)
                        n1051 = Select(t=0, s=w1944, f=2) -> (s? t:f=w1942:i32)
                        n1052 = property class="Ctl"(reference=w1945, "DisabledEnum"=w1942) -> ()  [unwired: 1 in, 2 out]
                      }
                    }
                    frame 7 {
                      n1053 = control-ref of="1 25"() -> (w1950:refnum<vi>)
                      n1054 = property class="Clust (严格)"(reference=w1950) -> ("Controls[]"=w1948:refnum<vi>[])  [unwired: 1 in, 2 out]
                      n1055 = for {
                        N: 12 -> [_]
                        tunnel: w1948 -> [w1956] mode=indexing
                        tunnel: w1947 -> [w1957]
                        i -> [w1954]
                        n1056 = Index Array(array=w1957, index=w1954) -> (element=w1955:bool)
                        n1057 = Select(t=0, s=w1955, f=2) -> (s? t:f=w1953:i32)
                        n1058 = property class="Ctl"(reference=w1956, "DisabledEnum"=w1953) -> ()  [unwired: 1 in, 2 out]
                      }
                    }
                    frame 8 {
                      n1059 = control-ref of="1 6"() -> (w1961:refnum<vi>)
                      n1060 = property class="Clust (严格)"(reference=w1961) -> ("Controls[]"=w1959:refnum<vi>[])  [unwired: 1 in, 2 out]
                      n1061 = for {
                        N: 12 -> [_]
                        tunnel: w1959 -> [w1967] mode=indexing
                        tunnel: w1958 -> [w1968]
                        i -> [w1965]
                        n1062 = Index Array(array=w1968, index=w1965) -> (element=w1966:bool)
                        n1063 = Select(t=0, s=w1966, f=2) -> (s? t:f=w1964:i32)
                        n1064 = property class="Ctl"(reference=w1967, "DisabledEnum"=w1964) -> ()  [unwired: 1 in, 2 out]
                      }
                    }
                    frame 99, Default {
                    }
                  }
                }
                n1065 = for {
                  N: 16 -> [_]
                  tunnel: w1678 -> [w1685]
                  i -> [w1686]
                  w1683 = 12 ("y")
                  n1066 = Multiply(x=w1686, y=w1683) -> (x*y=w1684:i32)
                  n1067 = Array Subset(array=w1685, index=w1684, length=w1683) -> (w1682:bool[])
                  n1068 = case shown="15" w1686 {
                    tunnel: w1682 -> [w1687 w1698 w1709 w1720 w1731 w1742 w1753 w1764 w1775 w1786 w1797 w1808 w1819 w1830 w1841 w1852 _]
                    frame 0 {
                      n1069 = control-ref of="1 102"() -> (w1690:refnum<vi>)
                      n1070 = property class="Clust (严格)"(reference=w1690) -> ("Controls[]"=w1688:refnum<vi>[])  [unwired: 1 in, 2 out]
                      n1071 = for {
                        N: 12 -> [_]
                        tunnel: w1688 -> [w1696] mode=indexing
                        tunnel: w1687 -> [w1697]
                        i -> [w1694]
                        n1072 = Index Array(array=w1697, index=w1694) -> (element=w1695:bool)
                        n1073 = Select(t=0, s=w1695, f=2) -> (s? t:f=w1693:i32)
                        n1074 = property class="Ctl"(reference=w1696, "DisabledEnum"=w1693) -> ()  [unwired: 1 in, 2 out]
                      }
                    }
                    frame 1 {
                      n1075 = control-ref of="1 3"() -> (w1701:refnum<vi>)
                      n1076 = property class="Clust (严格)"(reference=w1701) -> ("Controls[]"=w1699:refnum<vi>[])  [unwired: 1 in, 2 out]
                      n1077 = for {
                        N: 12 -> [_]
                        tunnel: w1699 -> [w1707] mode=indexing
                        tunnel: w1698 -> [w1708]
                        i -> [w1705]
                        n1078 = Index Array(array=w1708, index=w1705) -> (element=w1706:bool)
                        n1079 = Select(t=0, s=w1706, f=2) -> (s? t:f=w1704:i32)
                        n1080 = property class="Ctl"(reference=w1707, "DisabledEnum"=w1704) -> ()  [unwired: 1 in, 2 out]
                      }
                    }
                    frame 2 {
                      n1081 = control-ref of="1 4"() -> (w1712:refnum<vi>)
                      n1082 = property class="Clust (严格)"(reference=w1712) -> ("Controls[]"=w1710:refnum<vi>[])  [unwired: 1 in, 2 out]
                      n1083 = for {
                        N: 12 -> [_]
                        tunnel: w1710 -> [w1718] mode=indexing
                        tunnel: w1709 -> [w1719]
                        i -> [w1716]
                        n1084 = Index Array(array=w1719, index=w1716) -> (element=w1717:bool)
                        n1085 = Select(t=0, s=w1717, f=2) -> (s? t:f=w1715:i32)
                        n1086 = property class="Ctl"(reference=w1718, "DisabledEnum"=w1715) -> ()  [unwired: 1 in, 2 out]
                      }
                    }
                    frame 3 {
                      n1087 = control-ref of="1 6"() -> (w1723:refnum<vi>)
                      n1088 = property class="Clust (严格)"(reference=w1723) -> ("Controls[]"=w1721:refnum<vi>[])  [unwired: 1 in, 2 out]
                      n1089 = for {
                        N: 12 -> [_]
                        tunnel: w1721 -> [w1729] mode=indexing
                        tunnel: w1720 -> [w1730]
                        i -> [w1727]
                        n1090 = Index Array(array=w1730, index=w1727) -> (element=w1728:bool)
                        n1091 = Select(t=0, s=w1728, f=2) -> (s? t:f=w1726:i32)
                        n1092 = property class="Ctl"(reference=w1729, "DisabledEnum"=w1726) -> ()  [unwired: 1 in, 2 out]
                      }
                    }
                    frame 4 {
                      n1093 = control-ref of="1 7"() -> (w1734:refnum<vi>)
                      n1094 = property class="Clust (严格)"(reference=w1734) -> ("Controls[]"=w1732:refnum<vi>[])  [unwired: 1 in, 2 out]
                      n1095 = for {
                        N: 12 -> [_]
                        tunnel: w1732 -> [w1740] mode=indexing
                        tunnel: w1731 -> [w1741]
                        i -> [w1738]
                        n1096 = Index Array(array=w1741, index=w1738) -> (element=w1739:bool)
                        n1097 = Select(t=0, s=w1739, f=2) -> (s? t:f=w1737:i32)
                        n1098 = property class="Ctl"(reference=w1740, "DisabledEnum"=w1737) -> ()  [unwired: 1 in, 2 out]
                      }
                    }
                    frame 5 {
                      n1099 = control-ref of="1 8"() -> (w1745:refnum<vi>)
                      n1100 = property class="Clust (严格)"(reference=w1745) -> ("Controls[]"=w1743:refnum<vi>[])  [unwired: 1 in, 2 out]
                      n1101 = for {
                        N: 12 -> [_]
                        tunnel: w1743 -> [w1751] mode=indexing
                        tunnel: w1742 -> [w1752]
                        i -> [w1749]
                        n1102 = Index Array(array=w1752, index=w1749) -> (element=w1750:bool)
                        n1103 = Select(t=0, s=w1750, f=2) -> (s? t:f=w1748:i32)
                        n1104 = property class="Ctl"(reference=w1751, "DisabledEnum"=w1748) -> ()  [unwired: 1 in, 2 out]
                      }
                    }
                    frame 6 {
                      n1105 = control-ref of="1 9"() -> (w1756:refnum<vi>)
                      n1106 = property class="Clust (严格)"(reference=w1756) -> ("Controls[]"=w1754:refnum<vi>[])  [unwired: 1 in, 2 out]
                      n1107 = for {
                        N: 12 -> [_]
                        tunnel: w1754 -> [w1762] mode=indexing
                        tunnel: w1753 -> [w1763]
                        i -> [w1760]
                        n1108 = Index Array(array=w1763, index=w1760) -> (element=w1761:bool)
                        n1109 = Select(t=0, s=w1761, f=2) -> (s? t:f=w1759:i32)
                        n1110 = property class="Ctl"(reference=w1762, "DisabledEnum"=w1759) -> ()  [unwired: 1 in, 2 out]
                      }
                    }
                    frame 7 {
                      n1111 = control-ref of="1 10"() -> (w1767:refnum<vi>)
                      n1112 = property class="Clust (严格)"(reference=w1767) -> ("Controls[]"=w1765:refnum<vi>[])  [unwired: 1 in, 2 out]
                      n1113 = for {
                        N: 12 -> [_]
                        tunnel: w1765 -> [w1773] mode=indexing
                        tunnel: w1764 -> [w1774]
                        i -> [w1771]
                        n1114 = Index Array(array=w1774, index=w1771) -> (element=w1772:bool)
                        n1115 = Select(t=0, s=w1772, f=2) -> (s? t:f=w1770:i32)
                        n1116 = property class="Ctl"(reference=w1773, "DisabledEnum"=w1770) -> ()  [unwired: 1 in, 2 out]
                      }
                    }
                    frame 8 {
                      n1117 = control-ref of="1 26"() -> (w1778:refnum<vi>)
                      n1118 = property class="Clust (严格)"(reference=w1778) -> ("Controls[]"=w1776:refnum<vi>[])  [unwired: 1 in, 2 out]
                      n1119 = for {
                        N: 12 -> [_]
                        tunnel: w1776 -> [w1784] mode=indexing
                        tunnel: w1775 -> [w1785]
                        i -> [w1782]
                        n1120 = Index Array(array=w1785, index=w1782) -> (element=w1783:bool)
                        n1121 = Select(t=0, s=w1783, f=2) -> (s? t:f=w1781:i32)
                        n1122 = property class="Ctl"(reference=w1784, "DisabledEnum"=w1781) -> ()  [unwired: 1 in, 2 out]
                      }
                    }
                    frame 9 {
                      n1123 = control-ref of="1 27"() -> (w1789:refnum<vi>)
                      n1124 = property class="Clust (严格)"(reference=w1789) -> ("Controls[]"=w1787:refnum<vi>[])  [unwired: 1 in, 2 out]
                      n1125 = for {
                        N: 12 -> [_]
                        tunnel: w1787 -> [w1795] mode=indexing
                        tunnel: w1786 -> [w1796]
                        i -> [w1793]
                        n1126 = Index Array(array=w1796, index=w1793) -> (element=w1794:bool)
                        n1127 = Select(t=0, s=w1794, f=2) -> (s? t:f=w1792:i32)
                        n1128 = property class="Ctl"(reference=w1795, "DisabledEnum"=w1792) -> ()  [unwired: 1 in, 2 out]
                      }
                    }
                    frame 10 {
                      n1129 = control-ref of="1 28"() -> (w1800:refnum<vi>)
                      n1130 = property class="Clust (严格)"(reference=w1800) -> ("Controls[]"=w1798:refnum<vi>[])  [unwired: 1 in, 2 out]
                      n1131 = for {
                        N: 12 -> [_]
                        tunnel: w1798 -> [w1806] mode=indexing
                        tunnel: w1797 -> [w1807]
                        i -> [w1804]
                        n1132 = Index Array(array=w1807, index=w1804) -> (element=w1805:bool)
                        n1133 = Select(t=0, s=w1805, f=2) -> (s? t:f=w1803:i32)
                        n1134 = property class="Ctl"(reference=w1806, "DisabledEnum"=w1803) -> ()  [unwired: 1 in, 2 out]
                      }
                    }
                    frame 11 {
                      n1135 = control-ref of="1 29"() -> (w1811:refnum<vi>)
                      n1136 = property class="Clust (严格)"(reference=w1811) -> ("Controls[]"=w1809:refnum<vi>[])  [unwired: 1 in, 2 out]
                      n1137 = for {
                        N: 12 -> [_]
                        tunnel: w1809 -> [w1817] mode=indexing
                        tunnel: w1808 -> [w1818]
                        i -> [w1815]
                        n1138 = Index Array(array=w1818, index=w1815) -> (element=w1816:bool)
                        n1139 = Select(t=0, s=w1816, f=2) -> (s? t:f=w1814:i32)
                        n1140 = property class="Ctl"(reference=w1817, "DisabledEnum"=w1814) -> ()  [unwired: 1 in, 2 out]
                      }
                    }
                    frame 12 {
                      n1141 = control-ref of="1 30"() -> (w1822:refnum<vi>)
                      n1142 = property class="Clust (严格)"(reference=w1822) -> ("Controls[]"=w1820:refnum<vi>[])  [unwired: 1 in, 2 out]
                      n1143 = for {
                        N: 12 -> [_]
                        tunnel: w1820 -> [w1828] mode=indexing
                        tunnel: w1819 -> [w1829]
                        i -> [w1826]
                        n1144 = Index Array(array=w1829, index=w1826) -> (element=w1827:bool)
                        n1145 = Select(t=0, s=w1827, f=2) -> (s? t:f=w1825:i32)
                        n1146 = property class="Ctl"(reference=w1828, "DisabledEnum"=w1825) -> ()  [unwired: 1 in, 2 out]
                      }
                    }
                    frame 13 {
                      n1147 = control-ref of="1 31"() -> (w1833:refnum<vi>)
                      n1148 = property class="Clust (严格)"(reference=w1833) -> ("Controls[]"=w1831:refnum<vi>[])  [unwired: 1 in, 2 out]
                      n1149 = for {
                        N: 12 -> [_]
                        tunnel: w1831 -> [w1839] mode=indexing
                        tunnel: w1830 -> [w1840]
                        i -> [w1837]
                        n1150 = Index Array(array=w1840, index=w1837) -> (element=w1838:bool)
                        n1151 = Select(t=0, s=w1838, f=2) -> (s? t:f=w1836:i32)
                        n1152 = property class="Ctl"(reference=w1839, "DisabledEnum"=w1836) -> ()  [unwired: 1 in, 2 out]
                      }
                    }
                    frame 14 {
                      n1153 = control-ref of="1 32"() -> (w1844:refnum<vi>)
                      n1154 = property class="Clust (严格)"(reference=w1844) -> ("Controls[]"=w1842:refnum<vi>[])  [unwired: 1 in, 2 out]
                      n1155 = for {
                        N: 12 -> [_]
                        tunnel: w1842 -> [w1850] mode=indexing
                        tunnel: w1841 -> [w1851]
                        i -> [w1848]
                        n1156 = Index Array(array=w1851, index=w1848) -> (element=w1849:bool)
                        n1157 = Select(t=0, s=w1849, f=2) -> (s? t:f=w1847:i32)
                        n1158 = property class="Ctl"(reference=w1850, "DisabledEnum"=w1847) -> ()  [unwired: 1 in, 2 out]
                      }
                    }
                    frame 15 {
                      n1159 = control-ref of="1 33"() -> (w1855:refnum<vi>)
                      n1160 = property class="Clust (严格)"(reference=w1855) -> ("Controls[]"=w1853:refnum<vi>[])  [unwired: 1 in, 2 out]
                      n1161 = for {
                        N: 12 -> [_]
                        tunnel: w1853 -> [w1861] mode=indexing
                        tunnel: w1852 -> [w1862]
                        i -> [w1859]
                        n1162 = Index Array(array=w1862, index=w1859) -> (element=w1860:bool)
                        n1163 = Select(t=0, s=w1860, f=2) -> (s? t:f=w1858:i32)
                        n1164 = property class="Ctl"(reference=w1861, "DisabledEnum"=w1858) -> ()  [unwired: 1 in, 2 out]
                      }
                    }
                    frame 99, Default {
                    }
                  }
                }
              }
            }
          }
        }
      }
    }
    frame Enabled {
    }
  }
  n1165 = local write "213"(TRUE ("213")) -> ()
  n1166 = disable-structure shown="禁用" {
    frame Disabled {
      n1167 = control-ref of="选项卡控件"() -> (w1969:refnum<vi>)
      n1168 = control-ref of="均衡信息"() -> (w1970:refnum<vi>)
      n1169 = call "单数据解析_new.vi"(8:w1969) -> ("PF"=w1972:i32, "均衡标记"=w1971:i32[][])  [unwired: 1 in, 8 out]
      n1170 = call "均衡解析.vi"("位置"=w1972, "均衡标记"=w1971, "均衡引用"=w1970) -> ()  [unwired: 9 out]
    }
    frame Enabled {
    }
  }
  n1171 = local write "一次置位"(TRUE ("一次置位")) -> ()
  n1172 = for {
    N: 16 -> [_]
    i -> [w1974]
    n1173 = case shown="8" w1974 {
      tunnel: bool[] [FALSE, FALSE, FALSE, FALSE, FALSE, FALSE, FALSE, FALSE, FALSE, FALSE, FALSE, FALSE, FALSE] -> [w1976 w1981 w1986 w1991 w1996 w2001 w2006 w2011 w2016 w2021 w2026 w2031 w2036 w2041 w2046 w2051 _]
      frame 0 {
        n1174 = control-ref of="1 102"() -> (w1975:refnum<vi>)
        n1175 = property class="Clust (严格)"(reference=w1975) -> ("Controls[]"=w1977:refnum<vi>[])  [unwired: 1 in, 2 out]
        n1176 = for {
          tunnel: w1977 -> [w1978] mode=indexing
          tunnel: w1976 -> [w1979] mode=indexing
          n1177 = property class="Ctl"(reference=w1978, "Blinking"=w1979) -> ()  [unwired: 1 in, 2 out]
        }
      }
      frame 1 {
        n1178 = control-ref of="1 3"() -> (w1980:refnum<vi>)
        n1179 = property class="Clust (严格)"(reference=w1980) -> ("Controls[]"=w1982:refnum<vi>[])  [unwired: 1 in, 2 out]
        n1180 = for {
          tunnel: w1982 -> [w1983] mode=indexing
          tunnel: w1981 -> [w1984] mode=indexing
          n1181 = property class="Ctl"(reference=w1983, "Blinking"=w1984) -> ()  [unwired: 1 in, 2 out]
        }
      }
      frame 2 {
        n1182 = control-ref of="1 4"() -> (w1985:refnum<vi>)
        n1183 = property class="Clust (严格)"(reference=w1985) -> ("Controls[]"=w1987:refnum<vi>[])  [unwired: 1 in, 2 out]
        n1184 = for {
          tunnel: w1987 -> [w1988] mode=indexing
          tunnel: w1986 -> [w1989] mode=indexing
          n1185 = property class="Ctl"(reference=w1988, "Blinking"=w1989) -> ()  [unwired: 1 in, 2 out]
        }
      }
      frame 3 {
        n1186 = control-ref of="1 6"() -> (w1990:refnum<vi>)
        n1187 = property class="Clust (严格)"(reference=w1990) -> ("Controls[]"=w1992:refnum<vi>[])  [unwired: 1 in, 2 out]
        n1188 = for {
          tunnel: w1992 -> [w1993] mode=indexing
          tunnel: w1991 -> [w1994] mode=indexing
          n1189 = property class="Ctl"(reference=w1993, "Blinking"=w1994) -> ()  [unwired: 1 in, 2 out]
        }
      }
      frame 4 {
        n1190 = control-ref of="1 7"() -> (w1995:refnum<vi>)
        n1191 = property class="Clust (严格)"(reference=w1995) -> ("Controls[]"=w1997:refnum<vi>[])  [unwired: 1 in, 2 out]
        n1192 = for {
          tunnel: w1997 -> [w1998] mode=indexing
          tunnel: w1996 -> [w1999] mode=indexing
          n1193 = property class="Ctl"(reference=w1998, "Blinking"=w1999) -> ()  [unwired: 1 in, 2 out]
        }
      }
      frame 5 {
        n1194 = control-ref of="1 8"() -> (w2000:refnum<vi>)
        n1195 = property class="Clust (严格)"(reference=w2000) -> ("Controls[]"=w2002:refnum<vi>[])  [unwired: 1 in, 2 out]
        n1196 = for {
          tunnel: w2002 -> [w2003] mode=indexing
          tunnel: w2001 -> [w2004] mode=indexing
          n1197 = property class="Ctl"(reference=w2003, "Blinking"=w2004) -> ()  [unwired: 1 in, 2 out]
        }
      }
      frame 6 {
        n1198 = control-ref of="1 9"() -> (w2005:refnum<vi>)
        n1199 = property class="Clust (严格)"(reference=w2005) -> ("Controls[]"=w2007:refnum<vi>[])  [unwired: 1 in, 2 out]
        n1200 = for {
          tunnel: w2007 -> [w2008] mode=indexing
          tunnel: w2006 -> [w2009] mode=indexing
          n1201 = property class="Ctl"(reference=w2008, "Blinking"=w2009) -> ()  [unwired: 1 in, 2 out]
        }
      }
      frame 7 {
        n1202 = control-ref of="1 10"() -> (w2010:refnum<vi>)
        n1203 = property class="Clust (严格)"(reference=w2010) -> ("Controls[]"=w2012:refnum<vi>[])  [unwired: 1 in, 2 out]
        n1204 = for {
          tunnel: w2012 -> [w2013] mode=indexing
          tunnel: w2011 -> [w2014] mode=indexing
          n1205 = property class="Ctl"(reference=w2013, "Blinking"=w2014) -> ()  [unwired: 1 in, 2 out]
        }
      }
      frame 8 {
        n1206 = control-ref of="1 26"() -> (w2015:refnum<vi>)
        n1207 = property class="Clust (严格)"(reference=w2015) -> ("Controls[]"=w2017:refnum<vi>[])  [unwired: 1 in, 2 out]
        n1208 = for {
          tunnel: w2017 -> [w2018] mode=indexing
          tunnel: w2016 -> [w2019] mode=indexing
          n1209 = property class="Ctl"(reference=w2018, "Blinking"=w2019) -> ()  [unwired: 1 in, 2 out]
        }
      }
      frame 9 {
        n1210 = control-ref of="1 27"() -> (w2020:refnum<vi>)
        n1211 = property class="Clust (严格)"(reference=w2020) -> ("Controls[]"=w2022:refnum<vi>[])  [unwired: 1 in, 2 out]
        n1212 = for {
          tunnel: w2022 -> [w2023] mode=indexing
          tunnel: w2021 -> [w2024] mode=indexing
          n1213 = property class="Ctl"(reference=w2023, "Blinking"=w2024) -> ()  [unwired: 1 in, 2 out]
        }
      }
      frame 10 {
        n1214 = control-ref of="1 28"() -> (w2025:refnum<vi>)
        n1215 = property class="Clust (严格)"(reference=w2025) -> ("Controls[]"=w2027:refnum<vi>[])  [unwired: 1 in, 2 out]
        n1216 = for {
          tunnel: w2027 -> [w2028] mode=indexing
          tunnel: w2026 -> [w2029] mode=indexing
          n1217 = property class="Ctl"(reference=w2028, "Blinking"=w2029) -> ()  [unwired: 1 in, 2 out]
        }
      }
      frame 11 {
        n1218 = control-ref of="1 29"() -> (w2030:refnum<vi>)
        n1219 = property class="Clust (严格)"(reference=w2030) -> ("Controls[]"=w2032:refnum<vi>[])  [unwired: 1 in, 2 out]
        n1220 = for {
          tunnel: w2032 -> [w2033] mode=indexing
          tunnel: w2031 -> [w2034] mode=indexing
          n1221 = property class="Ctl"(reference=w2033, "Blinking"=w2034) -> ()  [unwired: 1 in, 2 out]
        }
      }
      frame 12 {
        n1222 = control-ref of="1 30"() -> (w2035:refnum<vi>)
        n1223 = property class="Clust (严格)"(reference=w2035) -> ("Controls[]"=w2037:refnum<vi>[])  [unwired: 1 in, 2 out]
        n1224 = for {
          tunnel: w2037 -> [w2038] mode=indexing
          tunnel: w2036 -> [w2039] mode=indexing
          n1225 = property class="Ctl"(reference=w2038, "Blinking"=w2039) -> ()  [unwired: 1 in, 2 out]
        }
      }
      frame 13 {
        n1226 = control-ref of="1 31"() -> (w2040:refnum<vi>)
        n1227 = property class="Clust (严格)"(reference=w2040) -> ("Controls[]"=w2042:refnum<vi>[])  [unwired: 1 in, 2 out]
        n1228 = for {
          tunnel: w2042 -> [w2043] mode=indexing
          tunnel: w2041 -> [w2044] mode=indexing
          n1229 = property class="Ctl"(reference=w2043, "Blinking"=w2044) -> ()  [unwired: 1 in, 2 out]
        }
      }
      frame 14 {
        n1230 = control-ref of="1 32"() -> (w2045:refnum<vi>)
        n1231 = property class="Clust (严格)"(reference=w2045) -> ("Controls[]"=w2047:refnum<vi>[])  [unwired: 1 in, 2 out]
        n1232 = for {
          tunnel: w2047 -> [w2048] mode=indexing
          tunnel: w2046 -> [w2049] mode=indexing
          n1233 = property class="Ctl"(reference=w2048, "Blinking"=w2049) -> ()  [unwired: 1 in, 2 out]
        }
      }
      frame 15 {
        n1234 = control-ref of="1 33"() -> (w2050:refnum<vi>)
        n1235 = property class="Clust (严格)"(reference=w2050) -> ("Controls[]"=w2052:refnum<vi>[])  [unwired: 1 in, 2 out]
        n1236 = for {
          tunnel: w2052 -> [w2053] mode=indexing
          tunnel: w2051 -> [w2054] mode=indexing
          n1237 = property class="Ctl"(reference=w2053, "Blinking"=w2054) -> ()  [unwired: 1 in, 2 out]
        }
      }
      frame 99, Default {
      }
    }
  }
  n1238 = for {
    N: 9 -> [_]
    i -> [w2056]
    n1239 = case shown="7" w2056 {
      tunnel: bool[] [FALSE, FALSE, FALSE, FALSE, FALSE, FALSE, FALSE, FALSE, FALSE, FALSE, FALSE, FALSE, FALSE] -> [w2058 w2063 w2068 w2073 w2078 w2083 w2088 w2093 w2098 _]
      frame 0 {
        n1240 = control-ref of="1 18"() -> (w2057:refnum<vi>)
        n1241 = property class="Clust (严格)"(reference=w2057) -> ("Controls[]"=w2059:refnum<vi>[])  [unwired: 1 in, 2 out]
        n1242 = for {
          tunnel: w2059 -> [w2060] mode=indexing
          tunnel: w2058 -> [w2061] mode=indexing
          n1243 = property class="Ctl"(reference=w2060, "Blinking"=w2061) -> ()  [unwired: 1 in, 2 out]
        }
      }
      frame 1 {
        n1244 = control-ref of="1 19"() -> (w2062:refnum<vi>)
        n1245 = property class="Clust (严格)"(reference=w2062) -> ("Controls[]"=w2064:refnum<vi>[])  [unwired: 1 in, 2 out]
        n1246 = for {
          tunnel: w2064 -> [w2065] mode=indexing
          tunnel: w2063 -> [w2066] mode=indexing
          n1247 = property class="Ctl"(reference=w2065, "Blinking"=w2066) -> ()  [unwired: 1 in, 2 out]
        }
      }
      frame 2 {
        n1248 = control-ref of="1 20"() -> (w2067:refnum<vi>)
        n1249 = property class="Clust (严格)"(reference=w2067) -> ("Controls[]"=w2069:refnum<vi>[])  [unwired: 1 in, 2 out]
        n1250 = for {
          tunnel: w2069 -> [w2070] mode=indexing
          tunnel: w2068 -> [w2071] mode=indexing
          n1251 = property class="Ctl"(reference=w2070, "Blinking"=w2071) -> ()  [unwired: 1 in, 2 out]
        }
      }
      frame 3 {
        n1252 = control-ref of="1 21"() -> (w2072:refnum<vi>)
        n1253 = property class="Clust (严格)"(reference=w2072) -> ("Controls[]"=w2074:refnum<vi>[])  [unwired: 1 in, 2 out]
        n1254 = for {
          tunnel: w2074 -> [w2075] mode=indexing
          tunnel: w2073 -> [w2076] mode=indexing
          n1255 = property class="Ctl"(reference=w2075, "Blinking"=w2076) -> ()  [unwired: 1 in, 2 out]
        }
      }
      frame 4 {
        n1256 = control-ref of="1 22"() -> (w2077:refnum<vi>)
        n1257 = property class="Clust (严格)"(reference=w2077) -> ("Controls[]"=w2079:refnum<vi>[])  [unwired: 1 in, 2 out]
        n1258 = for {
          tunnel: w2079 -> [w2080] mode=indexing
          tunnel: w2078 -> [w2081] mode=indexing
          n1259 = property class="Ctl"(reference=w2080, "Blinking"=w2081) -> ()  [unwired: 1 in, 2 out]
        }
      }
      frame 5 {
        n1260 = control-ref of="1 23"() -> (w2082:refnum<vi>)
        n1261 = property class="Clust (严格)"(reference=w2082) -> ("Controls[]"=w2084:refnum<vi>[])  [unwired: 1 in, 2 out]
        n1262 = for {
          tunnel: w2084 -> [w2085] mode=indexing
          tunnel: w2083 -> [w2086] mode=indexing
          n1263 = property class="Ctl"(reference=w2085, "Blinking"=w2086) -> ()  [unwired: 1 in, 2 out]
        }
      }
      frame 6 {
        n1264 = control-ref of="1 24"() -> (w2087:refnum<vi>)
        n1265 = property class="Clust (严格)"(reference=w2087) -> ("Controls[]"=w2089:refnum<vi>[])  [unwired: 1 in, 2 out]
        n1266 = for {
          tunnel: w2089 -> [w2090] mode=indexing
          tunnel: w2088 -> [w2091] mode=indexing
          n1267 = property class="Ctl"(reference=w2090, "Blinking"=w2091) -> ()  [unwired: 1 in, 2 out]
        }
      }
      frame 7 {
        n1268 = control-ref of="1 25"() -> (w2092:refnum<vi>)
        n1269 = property class="Clust (严格)"(reference=w2092) -> ("Controls[]"=w2094:refnum<vi>[])  [unwired: 1 in, 2 out]
        n1270 = for {
          tunnel: w2094 -> [w2095] mode=indexing
          tunnel: w2093 -> [w2096] mode=indexing
          n1271 = property class="Ctl"(reference=w2095, "Blinking"=w2096) -> ()  [unwired: 1 in, 2 out]
        }
      }
      frame 8 {
        n1272 = control-ref of="1 6"() -> (w2097:refnum<vi>)
        n1273 = property class="Clust (严格)"(reference=w2097) -> ("Controls[]"=w2099:refnum<vi>[])  [unwired: 1 in, 2 out]
        n1274 = for {
          tunnel: w2099 -> [w2100] mode=indexing
          tunnel: w2098 -> [w2101] mode=indexing
          n1275 = property class="Ctl"(reference=w2100, "Blinking"=w2101) -> ()  [unwired: 1 in, 2 out]
        }
      }
      frame 99, Default {
      }
    }
  }
  n1276 = local write "充电均衡"(T9 {"充电1"=13816530, "充电1"=13816530, "充电1"=13816530, "充电1"=13816530, "充电1"=13816530, "充电1"=13816530, "充电1"=13816530, "充电1"=13816530, "充电1"=13816530, "充电1"=13816530, "充电1"=13816530, "充电1"=13816530} ("充电均衡")) -> ()
  n1277 = disable-structure shown="禁用" {
    frame Disabled {
      n1278 = Not A Number/Path/Refnum?(number/path/refnum="数据") -> (NaN/Path/Refnum?=w2106:bool)
      n1279 = Not A Number/Path/Refnum?(number/path/refnum="数据位置") -> (NaN/Path/Refnum?=w2105:bool)
      n1280 = Or(x=w2106, y=w2105) -> (x .or. y?=w2104:bool)
      n1281 = case shown="假" w2104 {
        tunnel: "数据位置" -> [w2110 _]
        tunnel: "数据" -> [w2108 _]
        frame False {
          n1282 = property class="Arr (严格)"(reference=w2110) -> ("Value"=w2109:dbl[])  [unwired: 1 in, 2 out]
          n1283 = property class="Arr (严格)"(reference=w2108) -> ("Value"=w2107:dbl[])  [unwired: 1 in, 2 out]
          n1284 = call "数组去零.vi"("输入"=w2109) -> ("输出"=w2111:dbl[])
          n1285 = Array Size(array=w2111) -> (size(s)=w2112:i32)
          n1286 = Quotient & Remainder(x=w2112, y=24) -> (x-y*floor(x/y)=w2118:i32, floor(x/y)=w2115:i32)
          n1287 = Equal To 0?(x=w2118) -> (x = 0?=w2117:bool)
          n1288 = Increment(x=w2115) -> (x+1=w2114:i32)
          n1289 = Select(t=w2115, s=w2117, f=w2114) -> (s? t:f=w2116:i32)
          n1290 = Array Subset(array=w2107, length=w2112) -> (w2120:dbl[])  [unwired: 1 in]
          n1291 = for {
            N: w2116 -> [_]
            tunnel: w2120 -> [w2133]
            tunnel: [w2124] -> w2113
            tunnel: w2111 -> [w2127]
            i -> [w2130]
            w2125 = 24 ("y")
            n1292 = Multiply(x=w2130, y=w2125) -> (x*y=w2126:i32)
            n1293 = Increment(x=w2130) -> (x+1=w2128:i32)
            n1294 = Array Subset(array=w2133, index=w2126, length=w2125) -> (w2129:dbl[])
            n1295 = Array Subset(array=w2127, index=w2126, length=w2125) -> (w2123:dbl[])
            n1296 = Multiply(x=w2128, y=3) -> (x*y=w2131:i32)
            n1297 = Decrement(x=w2131) -> (x-1=w2122:i32)
            n1298 = Decrement(x=w2122) -> (x-1=w2121:i32)
            n1299 = call "表格数据输入(数值)-8.6.vi"("列数"=w2121, "数值数组"=w2123, "表格引用"=w2124) -> ()  [unwired: 9 out]
            n1300 = call "表格数据输入(数值)-8.6.vi"("列数"=w2122, "数值数组"=w2129, "表格引用"=w2124) -> ()  [unwired: 9 out]
          }
        }
        frame True {
        }
      }
    }
    frame Enabled {
    }
  }
  n1301 = disable-structure shown="禁用" {
    frame Disabled {
      n1302 = Multiply(x=12, y=24) -> (x*y=w2140:i32)
      n1303 = for {
        N: 12 -> [_]
        tunnel: [w2145] -> w2142 mode=indexing
        tunnel: [w2144] -> _
        tunnel: w2140 -> [w2144]
        i -> [w2151]
        n1304 = Increment(x=w2151) -> (x+1=w2150:i32)
        n1305 = Add(x=w2144, y=w2150) -> (x+y=w2146:i32)
        n1306 = Number To Decimal String(number=w2146) -> (decimal integer string=w2149:string)  [unwired: 1 out]
        n1307 = Concatenate Strings("第" ("字符串"), w2149, "串" ("字符串")) -> (w2145:string)
      }
      n1308 = Multiply(x=12, y=3) -> (x*y=w2137:i32)
      n1309 = call "表格数据输入-8.6.vi"("行数"=u32 0, "列数"=w2137, "字符串数组"=w2142) -> ("表格引用"=w2143:refnum<vi>)  [unwired: 8 out]
    }
    frame Enabled {
    }
  }
  n1310 = local write "停止"(FALSE ("停止")) -> ()
  "单选选项2" <- FALSE ("单选选项2")
